vi "SentinelCtrlSim v25 - Copy.vi"() -> ()   [LabVIEW 2011]
uses:
  <userlib>/configTool/configTool.llb/initConfigGlobal.vi
  <userlib>/configTool/configTool.llb/loadConfigFile.vi
  <userlib>/configTool/configTool.llb/closeConfig.vi
  <userlib>/configTool/configTool.llb/getProperty(DBL).vi
  <userlib>/configTool/configTool.llb/getProperty(I32).vi
  <userlib>/configTool/configTool.llb/getProperty(U32).vi
  <userlib>/configTool/configTool.llb/getProperty(BOOL).vi
  <userlib>/configTool/configTool.llb/getProperty(STR).vi
panel:
  in  "Data log path and filename":path=path "configuraitons/default_configuraiton.cfg"
  in  "Panels":T1(tab)
  in  "Test cell ID":string="default"
  in  "Operator name":string="default"
  in  "Lot number":string="default"
  in  "Configuration file path and filename":path
  in  "POWER":bool=TRUE
  in  "H1 low yield warning":dbl=95.0 min=0.0 max=100.0 step=1.0
  in  "Ignore alarms until AFTER this many cycles":i32=20
  in  "H1 low yield alarm":dbl=85.0 min=0.0 max=100.0 step=1.0
  in  "H1 low UPH warning (%)":dbl=95.0 min=1.0 max=48000.0 step=1.0
  in  "H1 low UPH alarm (%)":dbl=90.0 min=1.0 max=48000.0 step=1.0
  in  "Enable data logging of all events":bool=TRUE
  in  "Enable electronic notification of alarms":bool
  in  "H2 low UPH alarm (%)":dbl=90.0 min=1.0 max=48000.0 step=1.0
  in  "H2 low UPH warning (%)":dbl=95.0 min=1.0 max=48000.0 step=1.0
  in  "H2 low yield alarm":dbl=90.0 min=0.0 max=100.0 step=1.0
  in  "H2  low yield warning":dbl=95.0 min=0.0 max=100.0 step=1.0
  in  "H1 enable halt\non yield alarm":bool
  in  "H2 enable halt\non yield alarm":bool
  in  "H1 enable halt\non UPH alarm":bool
  in  "H2 enable halt\non UPH alarm":bool
  out "IT lock 1":bool caption="Index time\noptimization ON:\nmanual control of index time is LOCKED"
  in  "Parallelism":u32(slide)=8 min=1 max=16 step=1 scale=1.0..16.0
  in  "Simulate at max speed":bool=TRUE
  in  "H2 yield\nvariation (%)":i32(slide) min=-20 max=0 step=1
  in  "H1 yield\nvariation (%)":i32(slide) min=-20 max=0 step=1
  in  "H2 index time\nvariation (%)":i32(slide) min=-20 max=20 step=1 scale=-20.0..20.0
  in  "H1 index time\nvariation (%)":i32(slide) min=-20 max=20 step=1 scale=-20.0..20.0
  in  "H2 yield set":dbl(slide)=100.0 min=0.0 max=100.0 step=1.0 scale=0.0..100.0
  in  "H1 yield  set":dbl(slide)=100.0 min=0.0 max=100.0 step=1.0 scale=0.0..100.0
  in  "H2 index\ntime set":dbl(slide)=1.7000000000000004 min=0.5 max=10.0 step=0.1 scale=0.5..10.0 scale format="%.1f"
  in  "Test time\nvariation (%)":i32(slide) min=-100 max=100 step=1 scale=-50.0..100.0
  in  "H1 index\ntime set":dbl(slide)=1.7000000000000004 min=0.5 max=10.0 step=0.1 scale=0.5..10.0 scale format="%#.1f"
  in  "Test time set":dbl(slide)=1.8 min=0.5 max=10.0 step=0.01 scale=0.5..10.0 scale format="%.2f"
  in  "H1 IT orig":dbl
  in  "H2 IT orig":dbl
  in  "Min Test Time":dbl=0.499 min=0.1 max=1.0 step=0.1 format="%#.1g"
  out "H2 Single Handler UPH":dbl
  out "H1 Single Handler UPH":dbl
  out "UPH averaging":u32=20 min=2 max=100 step=1
  out "Yield averaging":u32=20 min=2 max=100 step=1
  in  "Push to reset charts":bool
  in  "Run / Stop":bool
  in  "Optimize handler speed":bool
  out "H1 parallelism":u8
  out "Utilization averaging":i32=6 min=2 max=20 step=1
  out "H2 nominal 2":bool=TRUE
  out "H2 warning 2":bool
  out "H2 alarm 2":bool
  out "H1 nominal 2":bool=TRUE
  out "H1 warning 2":bool
  out "H1 alarm 2":bool
  out "H2 Lock":bool
  out "H1 Lock":bool
  out "System UPH":u32(knob) caption="Sys UPH" scale=0.0..16800.0 scale format="%#.0f"
  out "Time Accerlation  Factor":dbl caption="Time acceleration \nfactor" format="%.1f"
  out "H2 Test Time":dbl caption="Index Time" format="%.2f"
  out "H2 Index Time":dbl caption="Index Time" format="%.2f"
  out "H2 Yield Guage":cluster{dbl, dbl}(knob) caption="H2 yield" scale=0.0..100.0
  out "H2 UPH":cluster{u32, u32}(knob) scale=0.0..8000.0 scale format="%#.0f"
  out "H2 nominal":bool=TRUE
  out "H2 warning":bool
  out "H2 alarm":bool
  out "H2 Indexing":bool
  out "H2 Testing":bool
  out "H2 Waiting":bool
  out "H2 Device Count":u32 caption="Device Count"
  out "H2 On/Off-line":bool
  out "H1 Test Time":dbl caption="Index Time" format="%.2f"
  out "H1 Index Time":dbl caption="Index Time" format="%.2f"
  out "H1 Yield Guage":cluster{dbl, dbl}(knob) caption="H1 yield" scale=0.0..100.0
  out "H1 UPH":cluster{u32, u32}(knob) scale=0.0..8000.0 scale format="%#.0f"
  out "H1 nominal":bool=TRUE
  out "H1 warning":bool
  out "H1 alarm":bool
  out "H1 Indexing":bool
  out "H1 Testing":bool
  out "H1 Waiting":bool
  out "H1 Device Count":u32 caption="Decvice Count"
  out "H1 On/Off-line":bool
  out "H1 Wait Time":dbl caption="Index Time" format="%.2f"
  out "H2 Wait Time":dbl caption="Index Time" format="%.2f"
  out "H1 Good Units":u32 caption="Decvice Count"
  out "H2 Good Units":u32 caption="Device Count"
  out "Sys utilization":dbl(knob) caption="Yield" scale=0.0..100.0
  out "H1 Yield Mon":dbl format="%.1f"
  out "H2 Yield  Mon":dbl format="%.1f"
  in  "H2 online":bool=TRUE
  in  "H1 online":bool=TRUE
  in  "Tester ready":bool=TRUE
  in  "Alert volume":u32(knob)=5 max=10 step=1 scale=0.0..10.0
  in  "Audio On / Off":bool=TRUE
  out "H1 results":u32
  out "H2 results":u32
  out "SysUtilMon":cluster{i32, i32}(graph)
  out "H2 parallelism":u8 caption="H2 Paralellism"
  out "H1 Pass":bool=TRUE
  out "H2 Pass":bool=TRUE
  in  "system statuts":T2(ring)
  in  "system states":T3(ring)
  out "YieldMon":cluster{i32, i32, i32, i32}(graph)
  in  "Utilization (%)":u32=80 min=10 max=100 step=10
  out "Calendar days required\nfor testing all units":dbl format="%.1f"
  in  "# of devices to test":u32=10000000 min=1000 max=100000000 step=1000
  out "$ saved":i64 format="%#.0f"
  out "H2 calc UPH":dbl format="%#.0f"
  out "H2 IT (scycle)":dbl format="%.2f"
  out "H2 TT (s/cycle)":dbl format="%.2f"
  out "H2 WT (s/cycle)":dbl format="%.2f"
  out "H1 WT (s/cycle)":dbl format="%.2f"
  out "H1 IT (s/cycle)":dbl format="%.2f"
  out "H1 TT (s/cycle)":dbl format="%.2f"
  out "H2 units/cycle":dbl caption="H1 Parallelism"
  out "H1 Parallelism 2":dbl caption="H1 units/cycle"
  out "Sim H1 UPH":u32
  out "Sim H2 UPH":u32
  out "H1 Index Time 2":dbl caption="H1 index time"
  out "H1 Test Time 2":dbl caption="H1 test time"
  out "H1 parallelism":dbl
  out "Unit cost (cents/device)":cluster{dbl, dbl}(graph)
  out "UPH per unit area":cluster{dbl, dbl}(graph)
  out "H2 UPH per unit area":dbl format="%.1f"
  out "H1 calc UPH":dbl format="%#.0f"
  out "Std cell floorspace area":dbl
  out "Tandem unit cost\n(cents/device)":dbl format="%.3f"
  out "Hours per month 2":dbl caption="Hours per month"
  out "Total Mo Costs ($/mo) 3":dbl caption="Tandem mo cost ($/mo)"
  out "Total Mo Costs ($/mo) 2":dbl caption="Std mo cost ($/mo)"
  out "H1 UPH per unit area":dbl format="%.1f"
  out "Std mo cost ($/mo)":dbl
  out "Simulated\nsystem UPH":u32 caption="Simulated\nSystem UPH"
  out "Std unit cost\n(cents/device)":dbl format="%.3g"
  out "H1 calc UPH":dbl format="%#.0f"
  out "Tandem\nfloorspace area":dbl
  out "Tandem UPH\nper unit area":dbl format="%.1f"
  in  "Second handler cost ($/mo)":dbl=2500.0 min=0.0 max=10000.0 step=100.0
  out "Tandem hourly\ncost ($/hr)":dbl format="%.2f"
  in  "Hours per month":i32=730
  out "Std hourly\ncost ($/hr)":dbl format="%.2f"
  in  "Celerint licensing cost ($/mo)":dbl=1000.0 min=0.0 max=10000.0 step=100.0
  in  "Celerint hardware cost ($/mo)":dbl min=0.0 max=10000.0 step=1.0
  in  "Additional floorspace\nfor second handler":i32=50 min=0 max=1000 step=10
  in  "Std cell \nfloorspace area":i32=200 min=10 max=1000 step=10
  in  "Overhead ($/mo)":dbl=1000.0 min=0.0 max=10000.0 step=100.0
  in  "Handler cost ($/mo)":dbl=2500.0 min=0.0 max=100000.0 step=100.0
  in  "Tester cost ($/mo)":dbl=8500.0 min=0.0 max=100000.0 step=500.0
  in  "Cost \nupper\nlimit":dbl(slide)=0.3293436293436293 min=0.1 scale=0.1..10.0 scale format="%.1f"
  in  "Cost 10X":bool caption="10X"
  in  "UPH \nupper\nlimit":dbl(slide)=100.0 min=1.0 scale=0.009000000000000001..100.0
  in  "UPH 10X":bool caption="10X"
  out "Number of text alerts":dbl caption="Number of alerts\nsent as notifications"
  in  "Enable text notification":bool
  out "Notifications Lot Display":string="default" caption="Lot number (not editable)"
  in  "Include\ndata log as\nattachment":bool=TRUE
  out "Number of email alerts":dbl caption="Number of alerts\nsent as notifications"
  out "Email alert - attachment (not editable)":path
  in  "Email alert - message":string="An alarm event has ocurred on a semiconductor test lot that you have requested to monitor.  Please see the attached data log for event details.\n\nThis message is generated automatically by the Sentinel Controller program.\n\nTo stop these messages, please contact the test floor operator and disable automatic alert notifictions.\n\n"
  in  "Email alert - engineer":string="harry@celerint.com"
  in  "Email alert - CC":string="hjr@celerint.com"
  in  "Enable email notification":bool
  in  "Carrier":enum16{"T-Mobile", "AT&T", "Verizon", "Sprint"}(ring)=enum."AT&T"
  in  "Phone number":string="5128263411"
  in  "Subject":string="From: Sentinel Controller"
  in  "Body":string="An alarm event has ocurred"
  out "H1 UPH warning limit":dbl
  out "H1 UPH alarm limit":dbl
  out "H2 UPH warning limit":dbl
  out "H2 UPH alarm limit":dbl
  # "Sentinel Controller\nTandlem Handler\nTest Cell \nwww.celerint.com"
  # "Turning off POWER will stop execution the Sentinel Controller Program"
  # "INPUT FILE"
  # "LOT INFORMATION"
  # "Celerint Sentinel Controller Simulator"
  # "HANDLER PERFORMANCE THRESHOLDS"
  # "Handler  1"
  # "Handler 2"
  # "Set UPH thresholds as % of max UPH"
  # "Set UPH thresholds as % of max UPH"
  # "test cycles (insertions)"
  # "Celerint Sentinel Controller Simulator"
  # "Handler 2"
  # "Handler 1"
  # "Yield"
  # "UPH"
  # "Yield"
  # "UPH"
  # "Data"
  # "Avg"
  # "lot yield (%)"
  # "good devices"
  # "devices tested"
  # "wait time"
  # "index time"
  # "test time"
  # "H1"
  # "H2"
  # "waiting"
  # "testing"
  # "indexing"
  # "on/off-line"
  # "Celerint Sentinel Controller Simulator"
  # "STANDARD SETUP"
  # "H2 calculated\nsimilarly"
  # "3600"
  # "TANDEM HANDLER SETUP"
  # "SAVINGS"
  # "3600 (s/hr)"
  # "3600 (s/hr)"
  # "Sentinel Controller\nTandlem Handler\nTest Cell \nwww.celerint.com"
  # "Lot number will be appended automatically:"
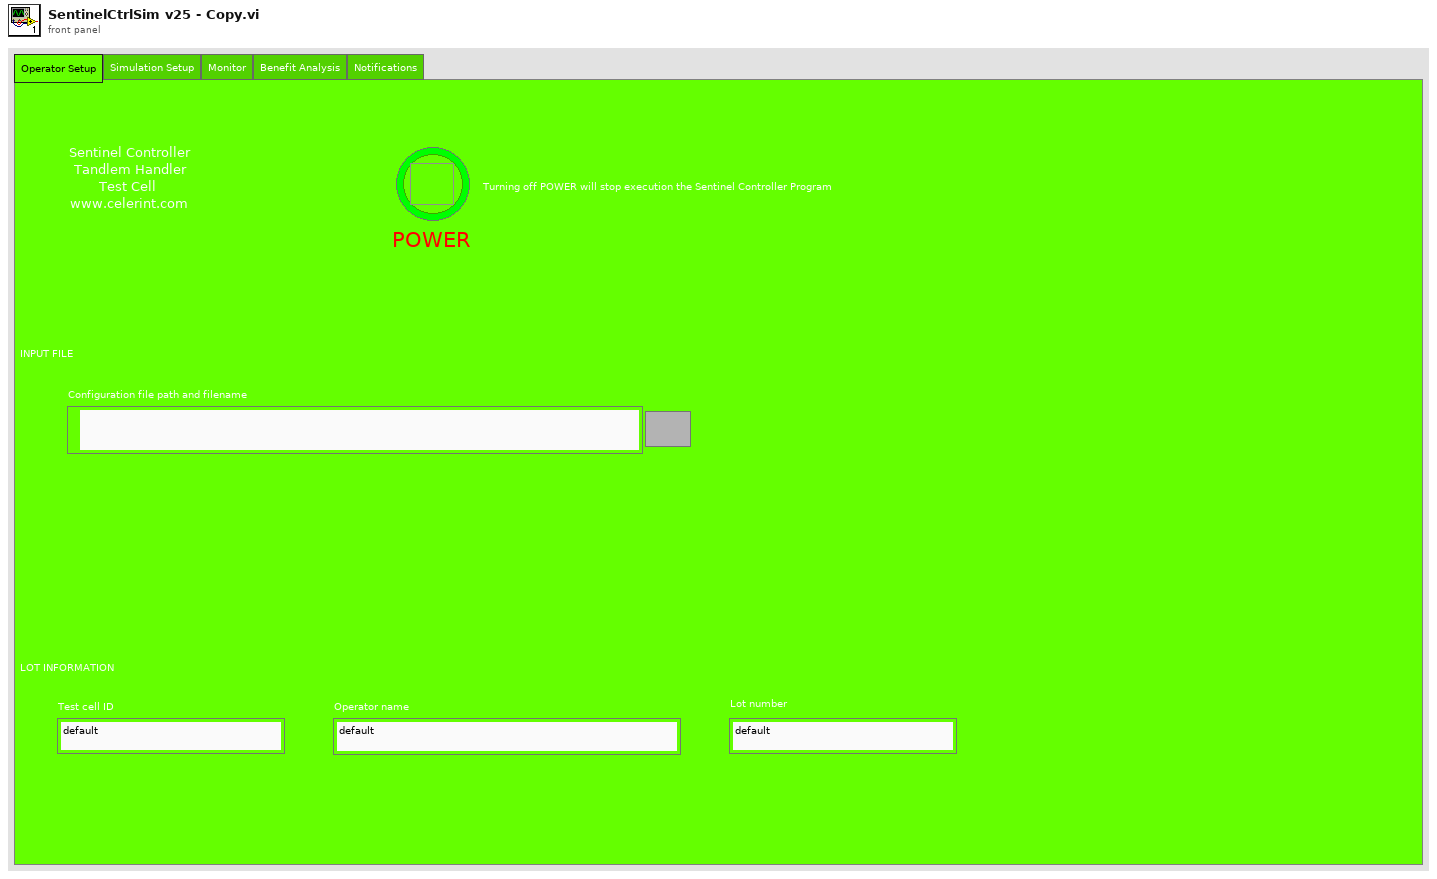
[diagram p1: front panel]
types:
  T1 = enum32{"Operator Setup", "Simulation Setup", "Monitor", "Benefit Analysis", "Notifications"}
  T2 = enum16{"H1NH2N", "H1NH2W", "H1NH2A", "H1WH2N", "H1WH2W", "H1WH2A", "H1AH2N", "H1AH2W", "H1AH2A"}
  T3 = enum16{"H1 Ready", "H2 Ready", "No Handler Ready"}
  T4 = enum16{"open", "replace", "create", "open or create", "replace or create", "replace or create with confirmation"}
  T5 = typedef "configRef.ctl" = refnum<vi>
  T6 = cluster{"rolling avg out":dbl, dbl, "H1 low yield alarm":dbl, "H2 low yield alarm":dbl}
  T7 = cluster{"rolling avg out":dbl, "H1 low yield alarm":dbl}
  T8 = cluster{dbl, "rolling avg out":dbl, "H1 low yield alarm":dbl, "H2 low yield alarm":dbl}
  T9 = cluster{"rolling avg out":dbl, "H2 low yield alarm":dbl}
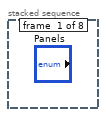
[diagram p2: hidden frame]
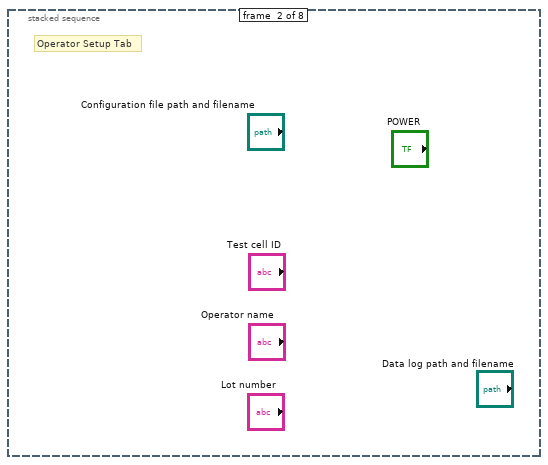
[diagram p3: hidden frame]
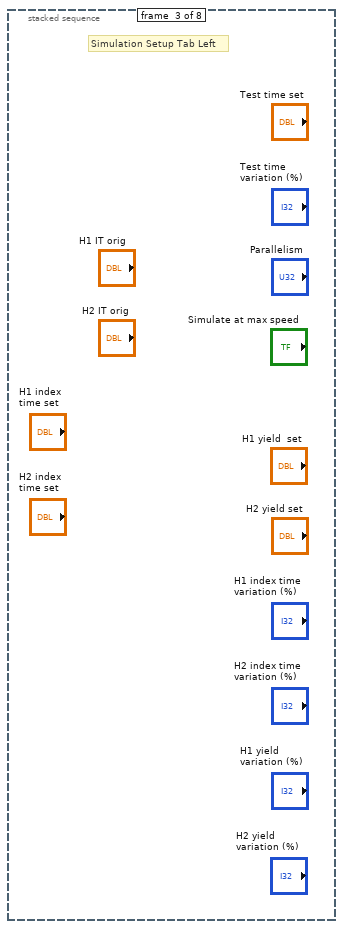
[diagram p4: hidden frame]
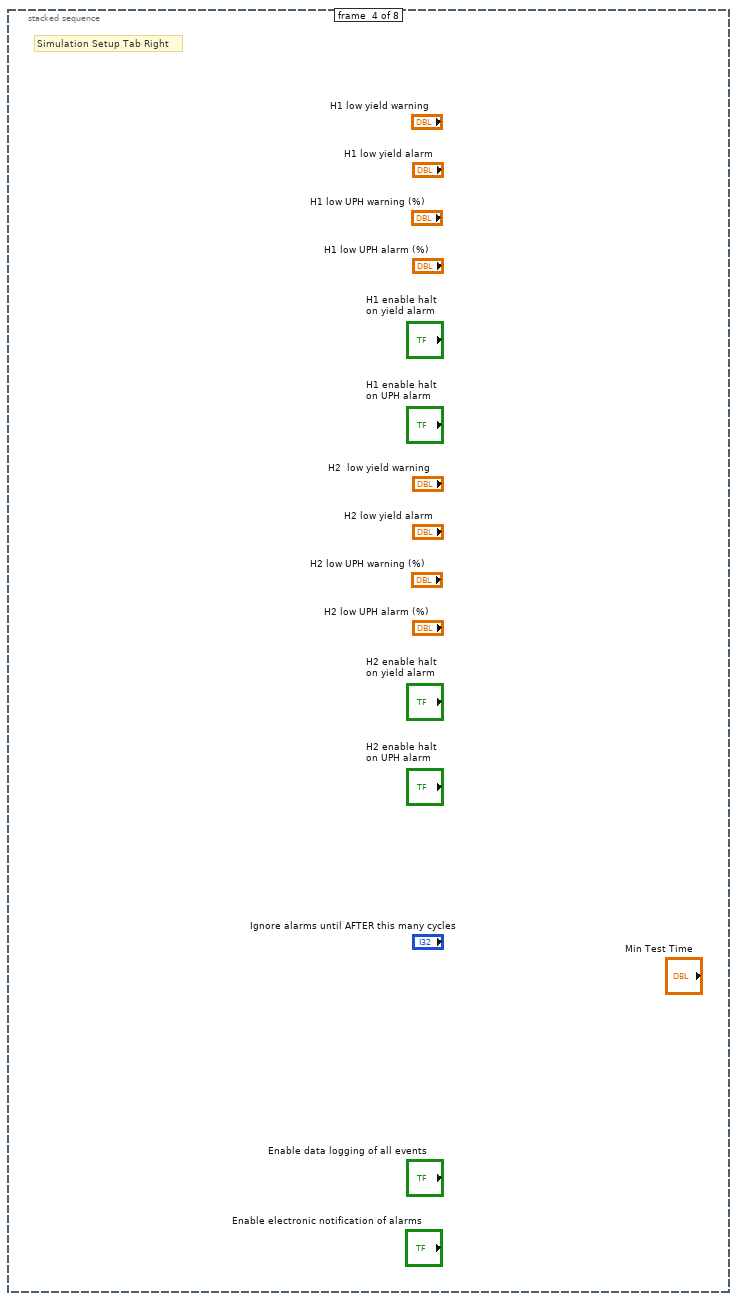
[diagram p5: hidden frame]
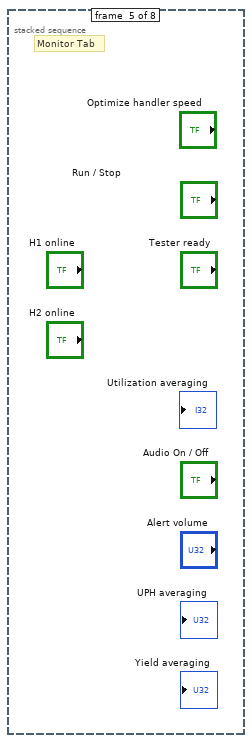
[diagram p6: hidden frame]
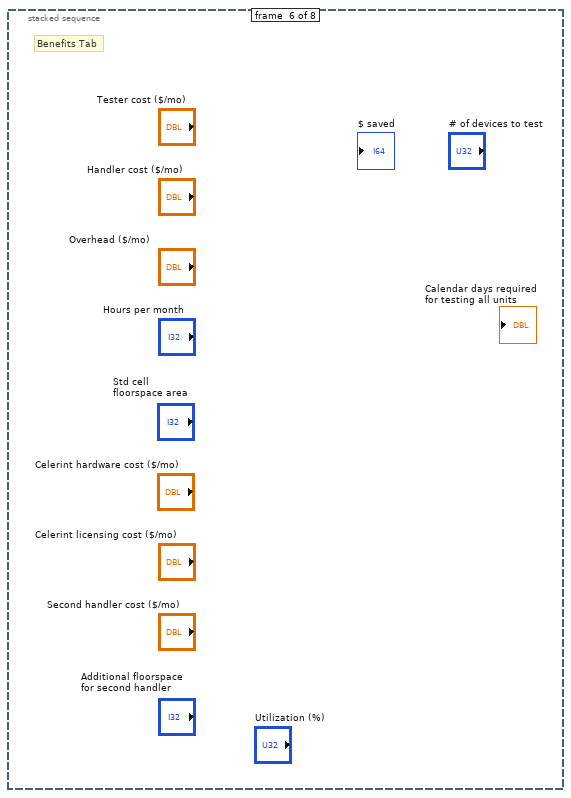
[diagram p7: hidden frame]
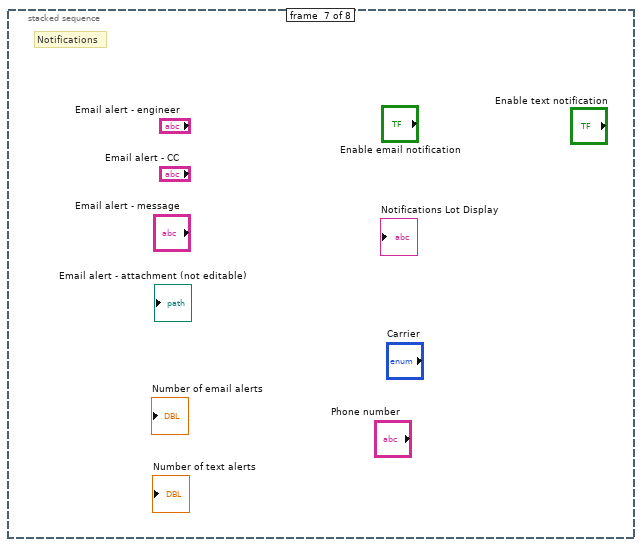
[diagram p8: hidden frame]
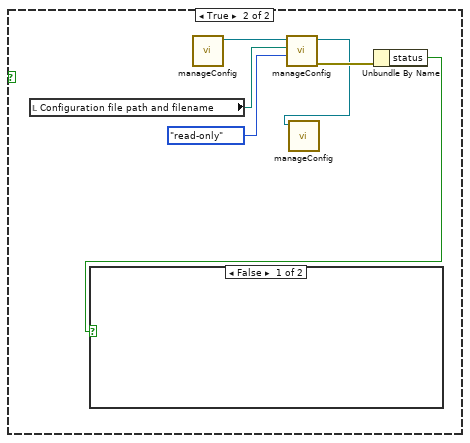
[diagram p9: hidden frame]
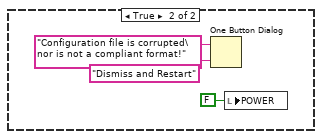
[diagram p10: hidden frame]
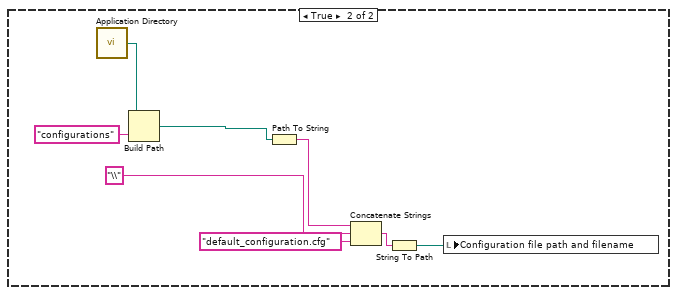
[diagram p11: hidden frame]
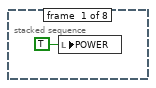
[diagram p13: hidden frame]
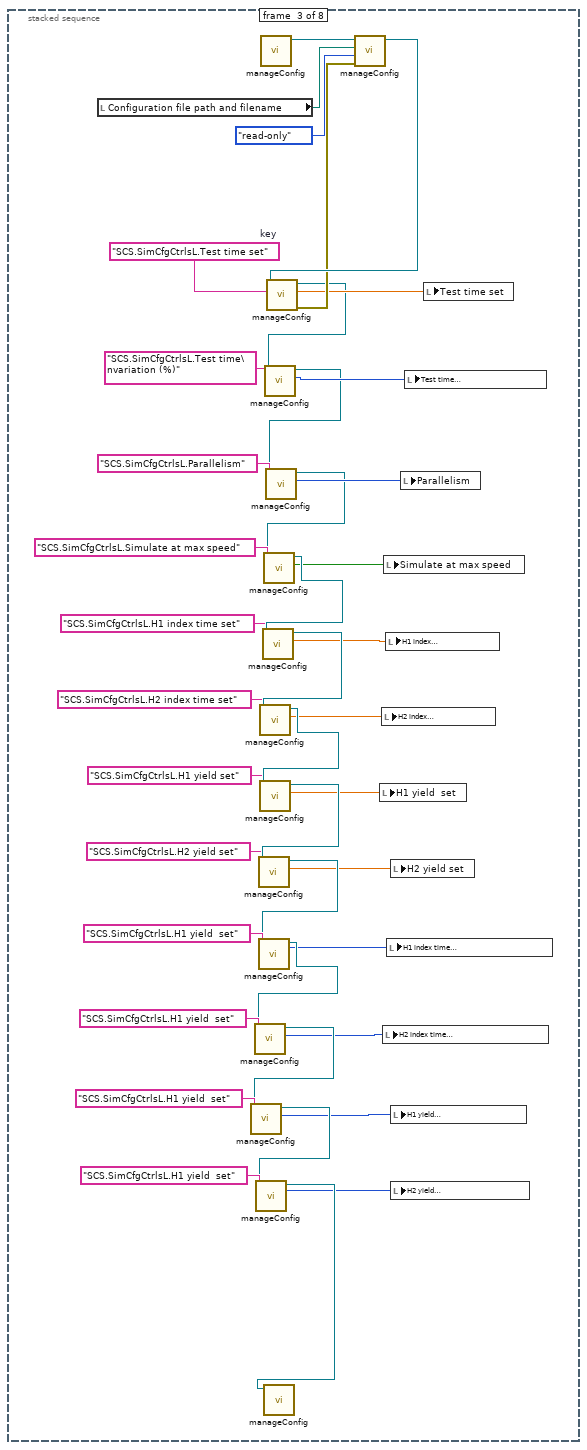
[diagram p15: hidden frame]
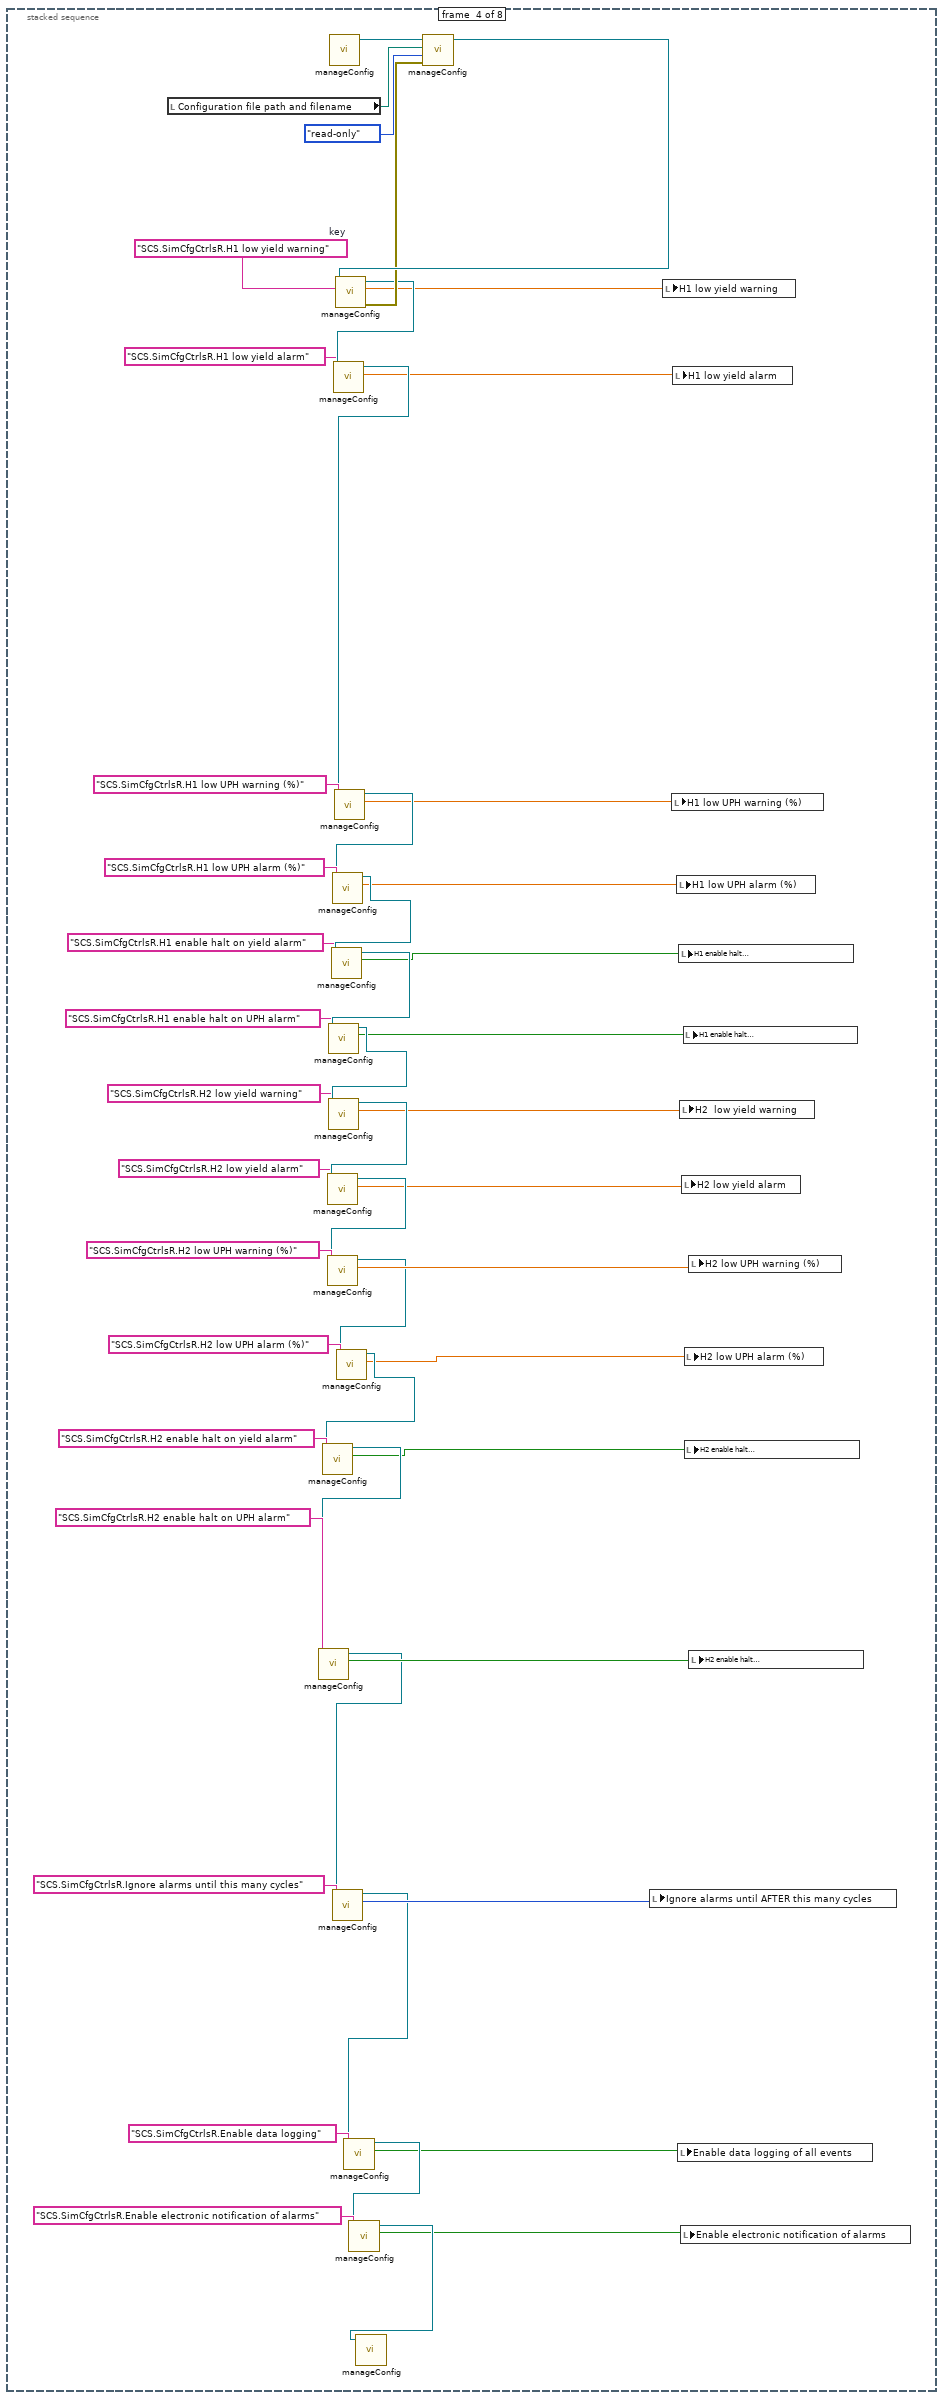
[diagram p16: hidden frame]
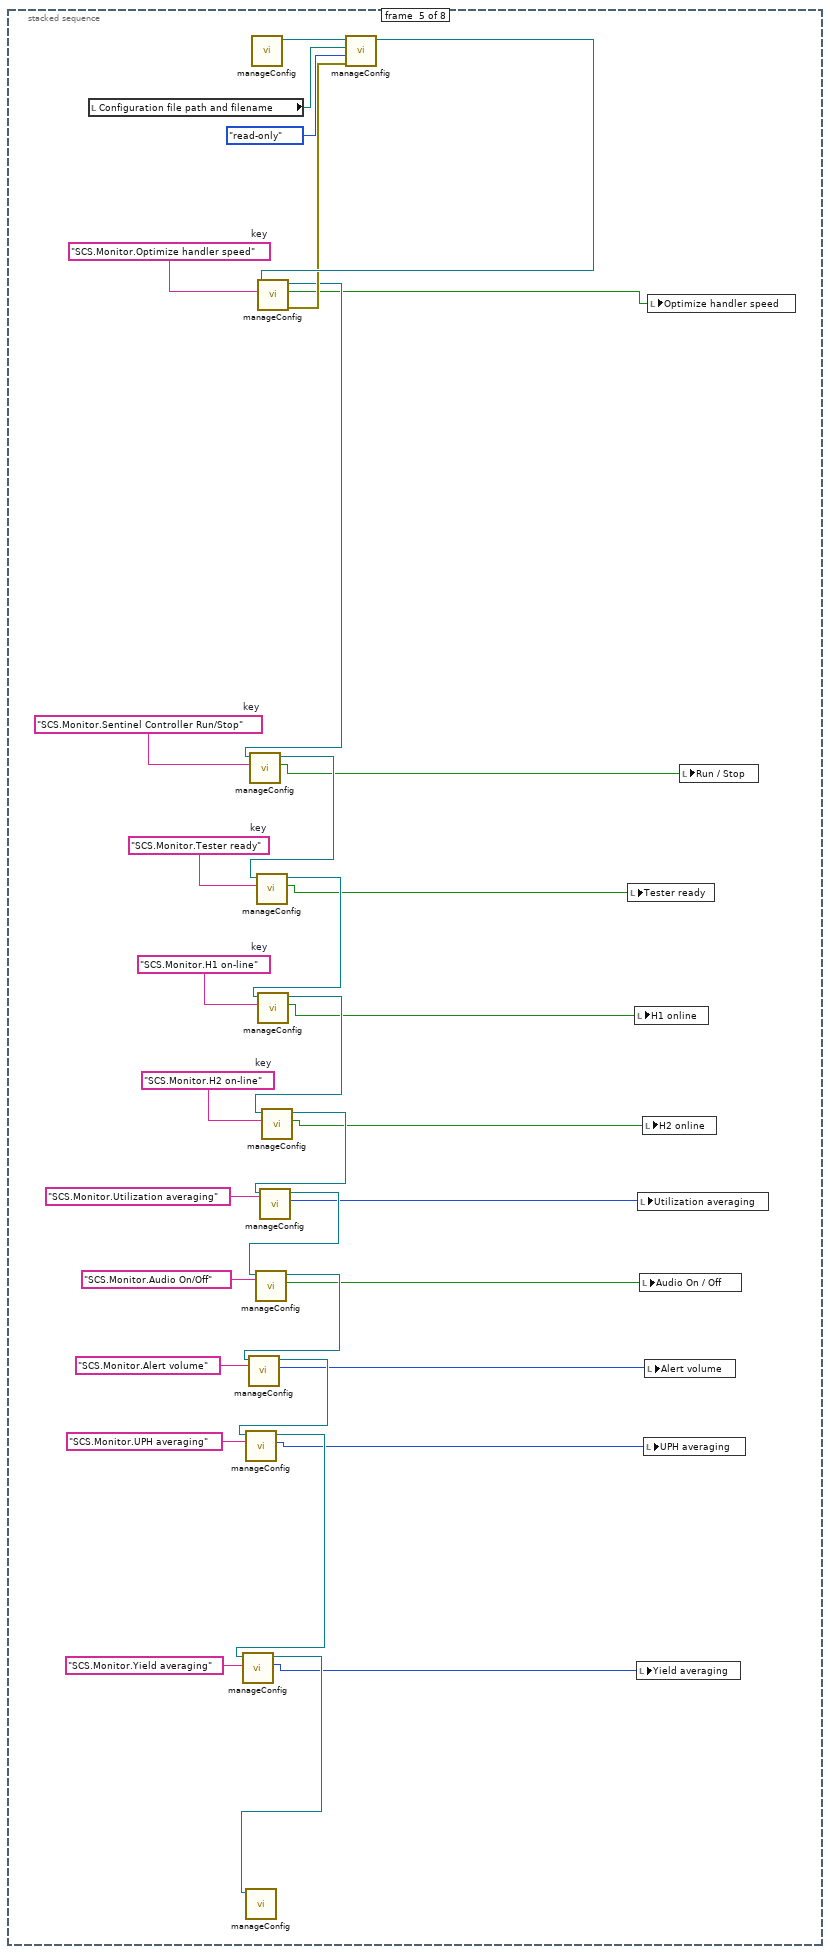
[diagram p17: hidden frame]
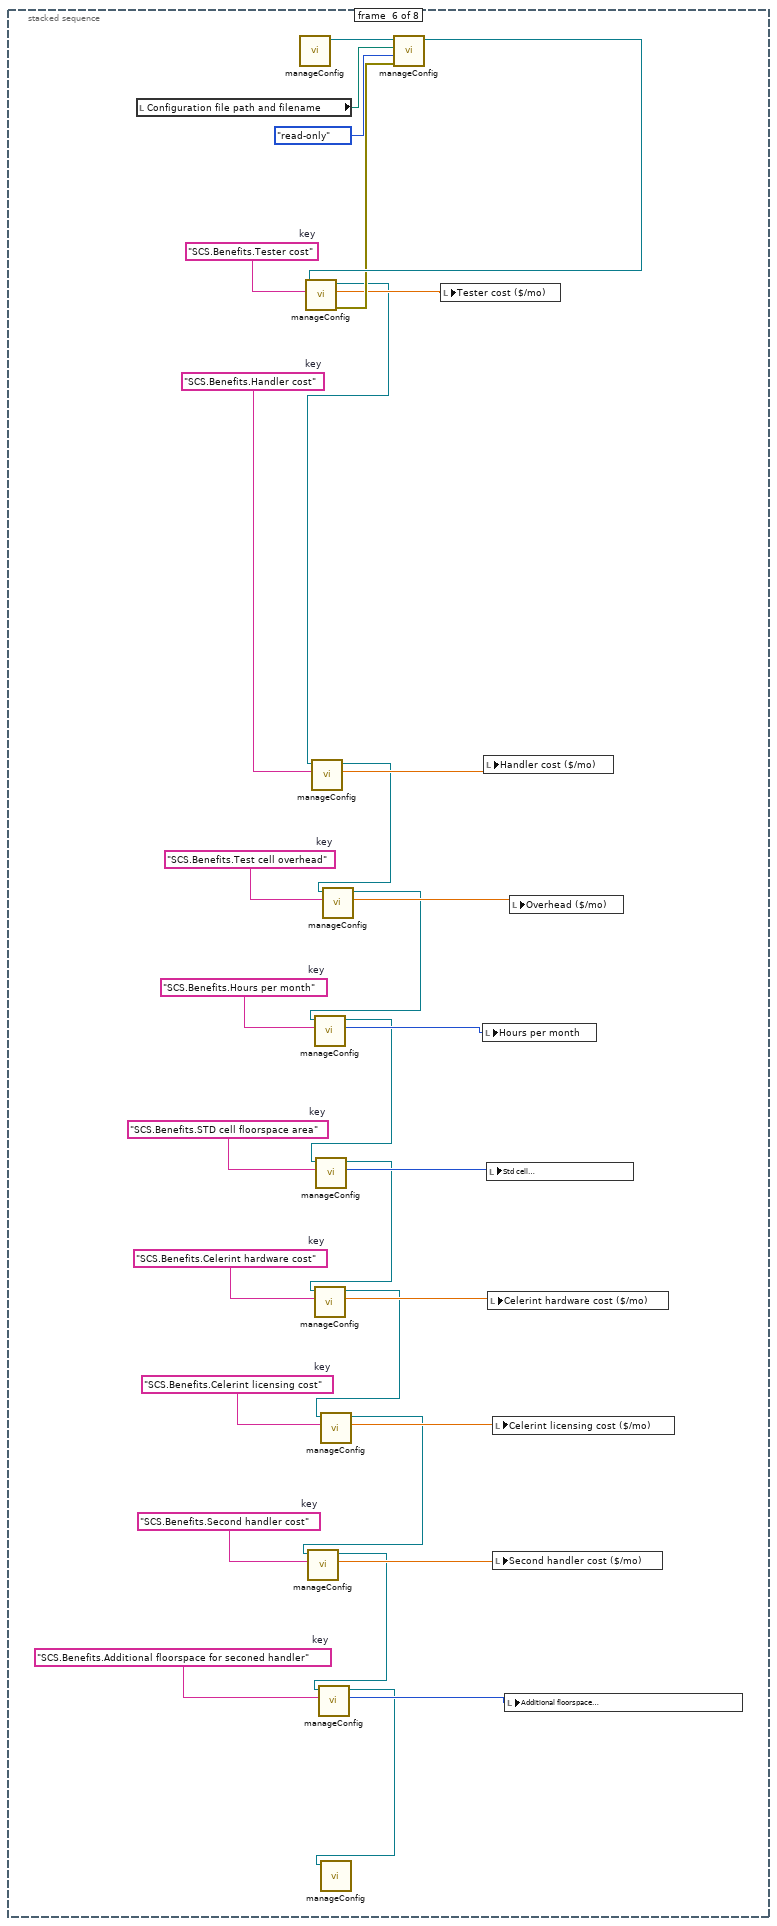
[diagram p18: hidden frame]
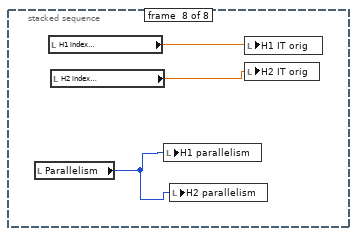
[diagram p19: hidden frame]
diagram:
  n1 = flat-sequence {
    frame #0 {
      # "This stacked sequence has all controls and indicators organized by the front panel panes."
      n2 = stacked-sequence {
        frame #0 {
        }
        frame #1 {
          # "Operator Setup Tab"
        }
        frame #2 {
          # "Simulation Setup Tab Left"
        }
        frame #3 {
          # "Simulation Setup Tab Right"
        }
        frame #4 {
          # "Monitor Tab"
        }
        frame #5 {
          # "Benefits Tab"
        }
        frame #6 {
          # "Notifications"
        }
        frame #7 {
          # "These are mostly indicators indicators"
        }
      }
    }
    frame #1 {
      n3 = local write "POWER"(TRUE ("POWER")) -> ()
    }
    frame #2 {
      n4 = local read "Configuration file path and filename"() -> (w4:path)
      n5 = Equal?(x=w4, y=path "") -> (x = y?=w3:bool)
      n6 = case shown="False" w3 {
        tunnel: w4 -> [w26 _]
        frame False {
          n7 = call <vilib>:"Check if File or Folder Exists.vi"("path"=w26) -> ("file or folder exists?"=w25:bool)  [unwired: 8 in, 2 out]
          n8 = case shown="False" w25 {
            frame False {
              n9 = local write "POWER"(FALSE ("POWER")) -> ()
              n10 = One Button Dialog(message="Configuration file does not exist!", button name ("OK")="Dismiss and Restart") -> ()  [unwired: 1 out]
            }
            frame True {
              n11 = local read "Configuration file path and filename"() -> (w33:path)
              n12 = call-poly <userlib>:"manageConfig.vi"() -> ("config ref out"=w34:T5)  [unwired: 10 in, 1 out]
              n13 = call-poly <userlib>:"manageConfig.vi"("access (0:read/write)"=enum16{"read/write", "read-only", "write-only"}."read-only", "config file path"=w33, "config ref"=w34) -> ("error out"=w32:errorcluster, "config ref out"=w30:T5)  [unwired: 6 in, 1 out]
              n14 = call-poly <userlib>:"manageConfig.vi"("config ref"=w30) -> ()  [unwired: 10 in, 1 out]
              n15 = Unbundle By Name(w32) -> ("status"=w31:bool)
              n16 = case shown="False" w31 {
                frame False {
                }
                frame True {
                  n17 = One Button Dialog(message="Configuration file is corrupted\nor is not a compliant format!", button name ("OK")="Dismiss and Restart") -> ()  [unwired: 1 out]
                  n18 = local write "POWER"(FALSE ("POWER")) -> ()
                }
              }
            }
          }
        }
        frame True {
          n19 = call <vilib>:"Application Directory.vi"() -> ("Application Directory"=w42:path)
          n20 = Build Path(base path=w42, name or relative path="configurations") -> (appended path=w39:path)
          n21 = Path To String(path=w39) -> (string=w44:string)
          n22 = Concatenate Strings(w44, "\\" ("string"), "default_configuration.cfg" ("string")) -> (w45:string)
          n23 = String To Path(string=w45) -> (path=w46:path)
          n24 = local write "Configuration file path and filename"(w46) -> ()
        }
      }
      n25 = Get Date/Time String(want seconds? (F)=TRUE) -> (date string=w19:string, time string=w11:string)  [unwired: 2 in]
      n26 = call <vilib>:"Application Directory.vi"() -> ("Application Directory"=w6:path)
      n27 = Build Path(base path=w6, name or relative path="datalogs") -> (appended path=w24:path)
      n28 = Search and Replace String(replace all?=TRUE ("replace all? (F)"), input string=w19, search string="/", replace string="-" ("replace string (\"\")")) -> (result string=w9:string)  [unwired: 4 in, 3 out]
      n29 = Search and Replace String(replace all?=TRUE ("replace all? (F)"), input string=w11, search string=":", replace string="." ("replace string (\"\")")) -> (result string=w10:string)  [unwired: 4 in, 3 out]
      n30 = Path To String(path=w24) -> (string=w15:string)
      n31 = Concatenate Strings(w15, "\\" ("string"), w9, " " ("string"), w10, ".txt" ("string")) -> (w21:string)
      n32 = String To Path(string=w21) -> (path=w23:path)
      n33 = local write "Data log path and filename"(w23) -> ()
    }
    frame #3 {
      n34 = local read "POWER"() -> (w47:bool)
      n35 = case shown="True" w47 {
        frame False {
        }
        frame True {
          n36 = stacked-sequence {
            frame #0 {
              n37 = local write "POWER"(TRUE ("POWER")) -> ()
            }
            frame #1 {
              # "nothing to do for the operator frame"
            }
            frame #2 {
              w88 = "SCS.SimCfgCtrlsL.Test time set"  # key
              n38 = local read "Configuration file path and filename"() -> (w84:path)
              n39 = call-poly <userlib>:"manageConfig.vi"() -> ("config ref out"=w85:T5)  [unwired: 10 in, 1 out]
              n40 = call-poly <userlib>:"manageConfig.vi"("access (0:read/write)"=enum16{"read/write", "read-only", "write-only"}."read-only", "config file path"=w84, "config ref"=w85) -> ("error out"=w87:errorcluster, "config ref out"=w89:T5)  [unwired: 6 in, 1 out]
              n41 = call-poly <userlib>:"manageConfig.vi"("error in"=w87, "property path"=w88, "config ref"=w89) -> ("data"=w81:dbl, "config ref out"=w63:T5)  [unwired: 5 in, 2 out]
              n42 = call-poly <userlib>:"manageConfig.vi"("property path"="SCS.SimCfgCtrlsL.Test time\nvariation (%)", "config ref"=w63) -> ("value"=w80:i32, "config ref out"=w62:T5)  [unwired: 6 in, 2 out]
              n43 = call-poly <userlib>:"manageConfig.vi"("property path"="SCS.SimCfgCtrlsL.Parallelism", "config ref"=w62) -> ("value"=w79:u32, "config ref out"=w64:T5)  [unwired: 6 in, 2 out]
              n44 = call-poly <userlib>:"manageConfig.vi"("property path"="SCS.SimCfgCtrlsL.Simulate at max speed", "config ref"=w64) -> ("value"=w61:bool, "config ref out"=w65:T5)  [unwired: 6 in, 2 out]
              n45 = call-poly <userlib>:"manageConfig.vi"("property path"="SCS.SimCfgCtrlsL.H1 index time set", "config ref"=w65) -> ("data"=w60:dbl, "config ref out"=w66:T5)  [unwired: 6 in, 2 out]
              n46 = call-poly <userlib>:"manageConfig.vi"("property path"="SCS.SimCfgCtrlsL.H2 index time set", "config ref"=w66) -> ("data"=w59:dbl, "config ref out"=w67:T5)  [unwired: 6 in, 2 out]
              n47 = call-poly <userlib>:"manageConfig.vi"("property path"="SCS.SimCfgCtrlsL.H1 yield set", "config ref"=w67) -> ("data"=w58:dbl, "config ref out"=w68:T5)  [unwired: 6 in, 2 out]
              n48 = call-poly <userlib>:"manageConfig.vi"("property path"="SCS.SimCfgCtrlsL.H2 yield set", "config ref"=w68) -> ("data"=w57:dbl, "config ref out"=w69:T5)  [unwired: 6 in, 2 out]
              n49 = call-poly <userlib>:"manageConfig.vi"("property path"="SCS.SimCfgCtrlsL.H1 yield  set", "config ref"=w69) -> ("value"=w56:i32, "config ref out"=w70:T5)  [unwired: 6 in, 2 out]
              n50 = call-poly <userlib>:"manageConfig.vi"("property path"="SCS.SimCfgCtrlsL.H1 yield  set", "config ref"=w70) -> ("value"=w55:i32, "config ref out"=w71:T5)  [unwired: 6 in, 2 out]
              n51 = call-poly <userlib>:"manageConfig.vi"("property path"="SCS.SimCfgCtrlsL.H1 yield  set", "config ref"=w71) -> ("value"=w54:i32, "config ref out"=w72:T5)  [unwired: 6 in, 2 out]
              n52 = call-poly <userlib>:"manageConfig.vi"("property path"="SCS.SimCfgCtrlsL.H1 yield  set", "config ref"=w72) -> ("value"=w53:i32, "config ref out"=w73:T5)  [unwired: 6 in, 2 out]
              n53 = call-poly <userlib>:"manageConfig.vi"("config ref"=w73) -> ()  [unwired: 10 in, 1 out]
              n54 = local write "H1 yield  set"(w58) -> ()
              n55 = local write "H2 index\ntime set"(w59) -> ()
              n56 = local write "H2 index time\nvariation (%)"(w55) -> ()
              n57 = local write "Simulate at max speed"(w61) -> ()
              n58 = local write "H1 index\ntime set"(w60) -> ()
              n59 = local write "H1 index time\nvariation (%)"(w56) -> ()
              n60 = local write "H2 yield set"(w57) -> ()
              n61 = local write "H1 yield\nvariation (%)"(w54) -> ()
              n62 = local write "H2 yield\nvariation (%)"(w53) -> ()
              n63 = local write "Parallelism"(w79) -> ()
              n64 = local write "Test time\nvariation (%)"(w80) -> ()
              n65 = local write "Test time set"(w81) -> ()
            }
            frame #3 {
              w138 = "SCS.SimCfgCtrlsR.H1 low yield warning"  # key
              n66 = local read "Configuration file path and filename"() -> (w134:path)
              n67 = call-poly <userlib>:"manageConfig.vi"() -> ("config ref out"=w135:T5)  [unwired: 10 in, 1 out]
              n68 = call-poly <userlib>:"manageConfig.vi"("access (0:read/write)"=enum16{"read/write", "read-only", "write-only"}."read-only", "config file path"=w134, "config ref"=w135) -> ("error out"=w137:errorcluster, "config ref out"=w139:T5)  [unwired: 6 in, 1 out]
              n69 = call-poly <userlib>:"manageConfig.vi"("error in"=w137, "property path"=w138, "config ref"=w139) -> ("data"=w110:dbl, "config ref out"=w121:T5)  [unwired: 5 in, 2 out]
              n70 = call-poly <userlib>:"manageConfig.vi"("property path"="SCS.SimCfgCtrlsR.H1 low yield alarm", "config ref"=w121) -> ("data"=w109:dbl, "config ref out"=w120:T5)  [unwired: 6 in, 2 out]
              n71 = call-poly <userlib>:"manageConfig.vi"("property path"="SCS.SimCfgCtrlsR.H1 low UPH warning (%)", "config ref"=w120) -> ("data"=w108:dbl, "config ref out"=w122:T5)  [unwired: 6 in, 2 out]
              n72 = call-poly <userlib>:"manageConfig.vi"("property path"="SCS.SimCfgCtrlsR.H1 low UPH alarm (%)", "config ref"=w122) -> ("data"=w107:dbl, "config ref out"=w123:T5)  [unwired: 6 in, 2 out]
              n73 = call-poly <userlib>:"manageConfig.vi"("property path"="SCS.SimCfgCtrlsR.H1 enable halt on yield alarm", "config ref"=w123) -> ("value"=w106:bool, "config ref out"=w124:T5)  [unwired: 6 in, 2 out]
              n74 = call-poly <userlib>:"manageConfig.vi"("property path"="SCS.SimCfgCtrlsR.H1 enable halt on UPH alarm", "config ref"=w124) -> ("value"=w105:bool, "config ref out"=w125:T5)  [unwired: 6 in, 2 out]
              n75 = call-poly <userlib>:"manageConfig.vi"("property path"="SCS.SimCfgCtrlsR.H2 low yield warning", "config ref"=w125) -> ("data"=w104:dbl, "config ref out"=w126:T5)  [unwired: 6 in, 2 out]
              n76 = call-poly <userlib>:"manageConfig.vi"("property path"="SCS.SimCfgCtrlsR.H2 low yield alarm", "config ref"=w126) -> ("data"=w103:dbl, "config ref out"=w127:T5)  [unwired: 6 in, 2 out]
              n77 = call-poly <userlib>:"manageConfig.vi"("property path"="SCS.SimCfgCtrlsR.H2 low UPH warning (%)", "config ref"=w127) -> ("data"=w102:dbl, "config ref out"=w94:T5)  [unwired: 6 in, 2 out]
              n78 = call-poly <userlib>:"manageConfig.vi"("property path"="SCS.SimCfgCtrlsR.H2 low UPH alarm (%)", "config ref"=w94) -> ("data"=w92:dbl, "config ref out"=w93:T5)  [unwired: 6 in, 2 out]
              n79 = call-poly <userlib>:"manageConfig.vi"("property path"="SCS.SimCfgCtrlsR.H2 enable halt on yield alarm", "config ref"=w93) -> ("value"=w101:bool, "config ref out"=w128:T5)  [unwired: 6 in, 2 out]
              n80 = call-poly <userlib>:"manageConfig.vi"("property path"="SCS.SimCfgCtrlsR.H2 enable halt on UPH alarm", "config ref"=w128) -> ("value"=w100:bool, "config ref out"=w91:T5)  [unwired: 6 in, 2 out]
              n81 = call-poly <userlib>:"manageConfig.vi"("property path"="SCS.SimCfgCtrlsR.Ignore alarms until this many cycles", "config ref"=w91) -> ("value"=w99:i32, "config ref out"=w90:T5)  [unwired: 6 in, 2 out]
              n82 = call-poly <userlib>:"manageConfig.vi"("property path"="SCS.SimCfgCtrlsR.Enable data logging", "config ref"=w90) -> ("value"=w98:bool, "config ref out"=w112:T5)  [unwired: 6 in, 2 out]
              n83 = call-poly <userlib>:"manageConfig.vi"("property path"="SCS.SimCfgCtrlsR.Enable electronic notification of alarms", "config ref"=w112) -> ("value"=w97:bool, "config ref out"=w111:T5)  [unwired: 6 in, 2 out]
              n84 = call-poly <userlib>:"manageConfig.vi"("config ref"=w111) -> ()  [unwired: 10 in, 1 out]
              n85 = local write "Ignore alarms until AFTER this many cycles"(w99) -> ()
              n86 = local write "H1 low yield warning"(w110) -> ()
              n87 = local write "H1 low UPH warning (%)"(w108) -> ()
              n88 = local write "H1 low yield alarm"(w109) -> ()
              n89 = local write "H1 low UPH alarm (%)"(w107) -> ()
              n90 = local write "Enable data logging of all events"(w98) -> ()
              n91 = local write "H1 enable halt\non yield alarm"(w106) -> ()
              n92 = local write "H2  low yield warning"(w104) -> ()
              n93 = local write "Enable electronic notification of alarms"(w97) -> ()
              n94 = local write "H2 low yield alarm"(w103) -> ()
              n95 = local write "H1 enable halt\non UPH alarm"(w105) -> ()
              n96 = local write "H2 low UPH alarm (%)"(w92) -> ()
              n97 = local write "H2 enable halt\non yield alarm"(w101) -> ()
              n98 = local write "H2 low UPH warning (%)"(w102) -> ()
              n99 = local write "H2 enable halt\non UPH alarm"(w100) -> ()
            }
            frame #4 {
              w165 = "SCS.Monitor.H2 on-line"  # key
              w166 = "SCS.Monitor.H1 on-line"  # key
              w167 = "SCS.Monitor.Tester ready"  # key
              w168 = "SCS.Monitor.Sentinel Controller Run/Stop"  # key
              w173 = "SCS.Monitor.Optimize handler speed"  # key
              n100 = local read "Configuration file path and filename"() -> (w169:path)
              n101 = call-poly <userlib>:"manageConfig.vi"() -> ("config ref out"=w170:T5)  [unwired: 10 in, 1 out]
              n102 = call-poly <userlib>:"manageConfig.vi"("access (0:read/write)"=enum16{"read/write", "read-only", "write-only"}."read-only", "config file path"=w169, "config ref"=w170) -> ("error out"=w172:errorcluster, "config ref out"=w174:T5)  [unwired: 6 in, 1 out]
              n103 = call-poly <userlib>:"manageConfig.vi"("error in"=w172, "property path"=w173, "config ref"=w174) -> ("value"=w149:bool, "config ref out"=w164:T5)  [unwired: 5 in, 2 out]
              n104 = call-poly <userlib>:"manageConfig.vi"("property path"=w168, "config ref"=w164) -> ("value"=w148:bool, "config ref out"=w163:T5)  [unwired: 6 in, 2 out]
              n105 = call-poly <userlib>:"manageConfig.vi"("property path"=w167, "config ref"=w163) -> ("value"=w147:bool, "config ref out"=w162:T5)  [unwired: 6 in, 2 out]
              n106 = call-poly <userlib>:"manageConfig.vi"("property path"=w166, "config ref"=w162) -> ("value"=w146:bool, "config ref out"=w161:T5)  [unwired: 6 in, 2 out]
              n107 = call-poly <userlib>:"manageConfig.vi"("property path"=w165, "config ref"=w161) -> ("value"=w145:bool, "config ref out"=w160:T5)  [unwired: 6 in, 2 out]
              n108 = call-poly <userlib>:"manageConfig.vi"("property path"="SCS.Monitor.Utilization averaging", "config ref"=w160) -> ("value"=w140:i32, "config ref out"=w159:T5)  [unwired: 6 in, 2 out]
              n109 = call-poly <userlib>:"manageConfig.vi"("property path"="SCS.Monitor.Audio On/Off", "config ref"=w159) -> ("value"=w144:bool, "config ref out"=w158:T5)  [unwired: 6 in, 2 out]
              n110 = call-poly <userlib>:"manageConfig.vi"("property path"="SCS.Monitor.Alert volume", "config ref"=w158) -> ("value"=w143:u32, "config ref out"=w157:T5)  [unwired: 6 in, 2 out]
              n111 = call-poly <userlib>:"manageConfig.vi"("property path"="SCS.Monitor.UPH averaging", "config ref"=w157) -> ("value"=w142:u32, "config ref out"=w156:T5)  [unwired: 6 in, 2 out]
              n112 = call-poly <userlib>:"manageConfig.vi"("property path"="SCS.Monitor.Yield averaging", "config ref"=w156) -> ("value"=w141:u32, "config ref out"=w155:T5)  [unwired: 6 in, 2 out]
              n113 = call-poly <userlib>:"manageConfig.vi"("config ref"=w155) -> ()  [unwired: 10 in, 1 out]
              n114 = local write "Tester ready"(w147) -> ()
              n115 = local write "H1 online"(w146) -> ()
              n116 = local write "Yield averaging"(w141) -> ()
              n117 = local write "Utilization averaging"(w140) -> ()
              n118 = local write "Audio On / Off"(w144) -> ()
              n119 = local write "H2 online"(w145) -> ()
              n120 = local write "UPH averaging"(w142) -> ()
              n121 = local write "Alert volume"(w143) -> ()
              n122 = local write "Optimize handler speed"(w149) -> ()
              n123 = local write "Run / Stop"(w148) -> ()
            }
            frame #5 {
              w193 = "SCS.Benefits.Additional floorspace for seconed handler"  # key
              w194 = "SCS.Benefits.Second handler cost"  # key
              w195 = "SCS.Benefits.Celerint licensing cost"  # key
              w196 = "SCS.Benefits.Celerint hardware cost"  # key
              w197 = "SCS.Benefits.STD cell floorspace area"  # key
              w198 = "SCS.Benefits.Hours per month"  # key
              w199 = "SCS.Benefits.Test cell overhead"  # key
              w200 = "SCS.Benefits.Handler cost"  # key
              w205 = "SCS.Benefits.Tester cost"  # key
              n124 = local read "Configuration file path and filename"() -> (w201:path)
              n125 = call-poly <userlib>:"manageConfig.vi"() -> ("config ref out"=w202:T5)  [unwired: 10 in, 1 out]
              n126 = call-poly <userlib>:"manageConfig.vi"("access (0:read/write)"=enum16{"read/write", "read-only", "write-only"}."read-only", "config file path"=w201, "config ref"=w202) -> ("error out"=w204:errorcluster, "config ref out"=w206:T5)  [unwired: 6 in, 1 out]
              n127 = call-poly <userlib>:"manageConfig.vi"("error in"=w204, "property path"=w205, "config ref"=w206) -> ("data"=w192:dbl, "config ref out"=w183:T5)  [unwired: 5 in, 2 out]
              n128 = call-poly <userlib>:"manageConfig.vi"("property path"=w200, "config ref"=w183) -> ("data"=w191:dbl, "config ref out"=w182:T5)  [unwired: 6 in, 2 out]
              n129 = call-poly <userlib>:"manageConfig.vi"("property path"=w199, "config ref"=w182) -> ("data"=w190:dbl, "config ref out"=w181:T5)  [unwired: 6 in, 2 out]
              n130 = call-poly <userlib>:"manageConfig.vi"("property path"=w198, "config ref"=w181) -> ("value"=w189:i32, "config ref out"=w180:T5)  [unwired: 6 in, 2 out]
              n131 = call-poly <userlib>:"manageConfig.vi"("property path"=w197, "config ref"=w180) -> ("value"=w188:i32, "config ref out"=w179:T5)  [unwired: 6 in, 2 out]
              n132 = call-poly <userlib>:"manageConfig.vi"("property path"=w196, "config ref"=w179) -> ("data"=w187:dbl, "config ref out"=w178:T5)  [unwired: 6 in, 2 out]
              n133 = call-poly <userlib>:"manageConfig.vi"("property path"=w195, "config ref"=w178) -> ("data"=w186:dbl, "config ref out"=w177:T5)  [unwired: 6 in, 2 out]
              n134 = call-poly <userlib>:"manageConfig.vi"("property path"=w194, "config ref"=w177) -> ("data"=w185:dbl, "config ref out"=w176:T5)  [unwired: 6 in, 2 out]
              n135 = call-poly <userlib>:"manageConfig.vi"("property path"=w193, "config ref"=w176) -> ("value"=w184:i32, "config ref out"=w175:T5)  [unwired: 6 in, 2 out]
              n136 = call-poly <userlib>:"manageConfig.vi"("config ref"=w175) -> ()  [unwired: 10 in, 1 out]
              n137 = local write "Tester cost ($/mo)"(w192) -> ()
              n138 = local write "Hours per month"(w189) -> ()
              n139 = local write "Handler cost ($/mo)"(w191) -> ()
              n140 = local write "Std cell \nfloorspace area"(w188) -> ()
              n141 = local write "Celerint hardware cost ($/mo)"(w187) -> ()
              n142 = local write "Celerint licensing cost ($/mo)"(w186) -> ()
              n143 = local write "Second handler cost ($/mo)"(w185) -> ()
              n144 = local write "Additional floorspace\nfor second handler"(w184) -> ()
              n145 = local write "Overhead ($/mo)"(w190) -> ()
            }
            frame #6 {
              w211 = "SCS.Notification.Enable text notification"  # key
              w217 = "SCS.Notification.Phone Number"  # key
              w218 = "SCS.Notification.Enable email notification"  # key
              w227 = "SCS.Notification.Email alert - Engineer"  # key
              n146 = local read "Configuration file path and filename"() -> (w224:path)
              n147 = local read "Lot number"() -> (w219:string)
              n148 = call-poly <userlib>:"manageConfig.vi"() -> ("config ref out"=w225:T5)  [unwired: 10 in, 1 out]
              n149 = local write "Number of email alerts"(0.0 ("Number of Emails Alerts Sent")) -> ()
              n150 = local write "Number of text alerts"(0.0 ("Number of Emails Alerts Sent")) -> ()
              n151 = local write "Notifications Lot Display"(w219) -> ()
              n152 = call-poly <userlib>:"manageConfig.vi"("access (0:read/write)"=enum16{"read/write", "read-only", "write-only"}."read-only", "config file path"=w224, "config ref"=w225) -> ("config ref out"=w228:T5)  [unwired: 6 in, 2 out]
              n153 = call-poly <userlib>:"manageConfig.vi"("property path"=w227, "config ref"=w228) -> ("value"=w222:string, "config ref out"=w216:T5)  [unwired: 6 in, 2 out]
              n154 = call-poly <userlib>:"manageConfig.vi"("property path"="SCS.Notification.Email alert CC", "config ref"=w216) -> ("value"=w221:string, "config ref out"=w215:T5)  [unwired: 6 in, 2 out]
              n155 = call-poly <userlib>:"manageConfig.vi"("property path"=w218, "config ref"=w215) -> ("value"=w213:bool, "config ref out"=w210:T5)  [unwired: 6 in, 2 out]
              n156 = call-poly <userlib>:"manageConfig.vi"("property path"=w211, "config ref"=w210) -> ("value"=w208:bool, "config ref out"=w209:T5)  [unwired: 6 in, 2 out]
              n157 = call-poly <userlib>:"manageConfig.vi"("property path"=w217, "config ref"=w209) -> ("value"=w212:string, "config ref out"=w214:T5)  [unwired: 6 in, 2 out]
              n158 = call-poly <userlib>:"manageConfig.vi"("config ref"=w214) -> ()  [unwired: 10 in, 1 out]
              n159 = local write "Email alert - engineer"(w222) -> ()
              n160 = local write "Phone number"(w212) -> ()
              n161 = local write "Email alert - CC"(w221) -> ()
              n162 = local write "Enable text notification"(w208) -> ()
              n163 = local write "Enable email notification"(w213) -> ()
            }
            frame #7 {
              n164 = local read "Parallelism"() -> (w231:u32)
              n165 = local read "H1 index\ntime set"() -> (w229:dbl)
              n166 = local read "H2 index\ntime set"() -> (w230:dbl)
              n167 = local write "H1 parallelism"(w231) -> ()
              n168 = local write "H2 parallelism"(w231) -> ()
              n169 = local write "H1 IT orig"(w229) -> ()
              n170 = local write "H2 IT orig"(w230) -> ()
            }
          }
        }
      }
    }
    frame #4 {
      n171 = local read "POWER"() -> (w232:bool)
      n172 = case shown="True" w232 {
        frame False {
        }
        frame True {
          w238 = "\r\n"
          n173 = local read "Data log path and filename"() -> (w233:path)
          n174 = local read "H1 online"() -> (w250:bool)
          n175 = local read "H2 online"() -> (w251:bool)
          n176 = local read "H1 UPH warning limit"() -> (w246:dbl)
          n177 = local read "H2 UPH warning limit"() -> (w248:dbl)
          n178 = local read "H2  low yield warning"() -> (w247:dbl)
          n179 = local read "H1 low yield warning"() -> (w245:dbl)
          n180 = case shown="True" w250 {
            tunnel: ["H1 Off-Line" "H1 On-Line"] -> w252
            frame False {
            }
            frame True {
            }
          }
          n181 = case shown="True" w251 {
            tunnel: ["H2 Off-Line" "H2 On-Line"] -> w257
            frame False {
            }
            frame True {
            }
          }
          n182 = local read "Operator name"() -> (w244:string)
          n183 = local read "Lot number"() -> (w242:string)
          n184 = local read "Test cell ID"() -> (w240:string)
          n185 = Number To Decimal String(number=w245) -> (decimal integer string=w254:string)  [unwired: 1 in]
          n186 = Number To Decimal String(number=w246) -> (decimal integer string=w256:string)  [unwired: 1 in]
          n187 = Number To Decimal String(number=w247) -> (decimal integer string=w259:string)  [unwired: 1 in]
          n188 = Number To Decimal String(number=w248) -> (decimal integer string=w261:string)  [unwired: 1 in]
          n189 = Get Date/Time String() -> (date string=w235:string, time string=w237:string)  [unwired: 3 in]
          n190 = Concatenate Strings(w235, "   " ("string"), w237, w238, "Test Cell ID: ", w240, w238, "Lot Number: ", w242, w238, "Operator Name:  ", w244, w238, "System Started", w238, w252, w238, "H1 Low Yield Warning Limit: ", w254, w238, "H1 Low UPH Warning Limit: ", w256, w238, w257, w238, "H2 Low Yield Warning Limit: ", w259, w238, "H2 Low UPH Warning Limit: ", w261, w238, w238) -> (w262:string)
          n191 = call "SentinelDatalog.vi"("operation (0:open)"=T4."open or create", "String"=w262, "data log path"=w233) -> ()  [unwired: 8 in, 1 out]
          n192 = local write "Email alert - attachment (not editable)"(w233) -> ()
        }
      }
    }
    frame #5 {
      n193 = local read "POWER"() -> (w267:bool)
      n194 = case shown="True" w267 {
        frame False {
        }
        frame True {
          n195 = while {
            stop <- w268 stop-if-true
            # "Sentinel operating loop\n- tester loop\n- H1 loop\n- H2 loop\n- controls loop\n- alarm state machine loop\nExit with Power off"
            n196 = local read "POWER"() -> (w269:bool)
            n197 = Not(x=w269) -> (.not. x?=w268:bool)
            n198 = Wait (ms)(milliseconds to wait=u32 100) -> ()  [unwired: 1 out]
            n199 = local read "Run / Stop"() -> (w270:bool)
            n200 = case shown="True" w270 {
              frame False {
              }
              frame True {
                w280 = 0.0
                w282 = 0.0
                w283 = 0.0
                w284 = 0.0
                w287 = 0.0
                n201 = while {
                  shift-right: [w1013] -> _
                  shift-left: FALSE ("Optimize Handler Speed") -> [w1017]
                  i -> [w1001]
                  stop <- w1052 stop-if-true
                  n202 = local read "Additional floorspace\nfor second handler"() -> (w1003:i32)
                  n203 = local read "Celerint hardware cost ($/mo)"() -> (w1006:dbl)
                  n204 = local read "Celerint licensing cost ($/mo)"() -> (w1005:dbl)
                  n205 = local read "Second handler cost ($/mo)"() -> (w1004:dbl)
                  n206 = local read "Overhead ($/mo)"() -> (w1009:dbl)
                  n207 = local read "Handler cost ($/mo)"() -> (w1010:dbl)
                  n208 = local read "Tester cost ($/mo)"() -> (w1011:dbl)
                  n209 = local read "POWER"() -> (w1055:bool)
                  n210 = local read "Std cell \nfloorspace area"() -> (w1048:i32)
                  n211 = local read "H2 index\ntime set"() -> (w1021:dbl)
                  n212 = local read "H1 index\ntime set"() -> (w1018:dbl)
                  "H1 Index Time 2" <- w1018
                  n213 = local read "Simulate at max speed"() -> (w1040:bool)
                  n214 = local read "Push to reset charts"() -> (w999:bool)
                  n215 = local read "Run / Stop"() -> (w1002:bool)
                  n216 = local read "Test time set"() -> (w1033:dbl)
                  "H1 Test Time 2" <- w1033
                  n217 = local read "Hours per month"() -> (w1008:i32)
                  "Hours per month 2" <- w1008
                  n218 = local read "Parallelism"() -> (w1032:u32)
                  "H1 parallelism" <- w1032
                  "H1 Parallelism 2" <- w1032
                  "H2 units/cycle" <- w1032
                  n219 = Not(x=w1055) -> (.not. x?=w1053:bool)
                  n220 = local read "Optimize handler speed"() -> (w1013:bool)
                  "IT lock 1" <- w1013
                  n221 = local read "Alert volume"() -> (w1012:u32)
                  n222 = Compound Arithmetic op=ADD(w1006, w1005, w1004) -> (w1038:dbl)
                  n223 = Compound Arithmetic op=ADD(w1011, w1010, w1009) -> (w1037:dbl)
                  n224 = Compound Arithmetic op=ADD(w1011, w1009) -> (→"Std mo cost ($/mo)" →"Total Mo Costs ($/mo) 2":dbl)
                  n225 = local read "H1 IT orig"() -> (w1015:dbl)
                  n226 = local read "H2 IT orig"() -> (w1016:dbl)
                  n227 = Not(x=w1002) -> (.not. x?=w1054:bool)
                  n228 = Add(x=w1003, y=w1048) -> (x+y=→"Tandem\nfloorspace area":i32)
                  n229 = Add(x=w1038, y=w1037) -> (x+y=→"Total Mo Costs ($/mo) 3":dbl)
                  n230 = Divide(x=w1038, y=w1008) -> (x/y=w1049:dbl)
                  n231 = Divide(x=w1037, y=w1008) -> (x/y=w1046:dbl)
                  "Std hourly\ncost ($/hr)" <- w1046
                  n232 = case shown="True" w999 {
                    frame False {
                    }
                    frame True {
                      w1072 = cluster{dbl, dbl}[] [] ("History Data")
                      (unwired) cluster{dbl, dbl, dbl}[] [] ("History Data")
                      n233 = property on="YieldMon" class="WFChart (strict)"("History Data"=cluster{dbl, dbl, dbl, dbl}[] []) -> ()  [unwired: 2 in, 2 out]
                      n234 = property on="Unit cost (cents/device)" class="WFChart (strict)"("History Data"=w1072) -> ()  [unwired: 2 in, 2 out]
                      n235 = property on="UPH per unit area" class="WFChart (strict)"("History Data"=w1072) -> ()  [unwired: 2 in, 2 out]
                      n236 = property on="SysUtilMon" class="WFChart (strict)"("History Data"=w1072) -> ()  [unwired: 2 in, 2 out]
                    }
                  }
                  n237 = property on="Unit cost (cents/device)" class="WFChart (strict)"("YScale.Maximum"="Cost \nupper\nlimit") -> ()  [unwired: 2 in, 2 out]
                  n238 = case shown="False" "Cost 10X" {
                    frame False {
                      n239 = property on="Cost \nupper\nlimit" class="Slide (strict)"("Scale.Maximum"=10.0 ("Scale.Range:Maximum")) -> ()  [unwired: 2 in, 2 out]
                    }
                    frame True {
                      n240 = property on="Cost \nupper\nlimit" class="Slide (strict)"("Scale.Maximum"=100.0 ("Scale.Range:Maximum")) -> ()  [unwired: 2 in, 2 out]
                    }
                  }
                  n241 = property on="UPH per unit area" class="WFChart (strict)"("YScale.Maximum"="UPH \nupper\nlimit") -> ()  [unwired: 2 in, 2 out]
                  n242 = case shown="True" "UPH 10X" {
                    frame False {
                      n243 = property on="UPH \nupper\nlimit" class="Slide (strict)"("Scale.Maximum"=100.0 ("Scale.Range:Maximum")) -> ()  [unwired: 2 in, 2 out]
                    }
                    frame True {
                      n244 = property on="UPH \nupper\nlimit" class="Slide (strict)"("Scale.Maximum"=1000.0 ("Scale.Range:Maximum")) -> ()  [unwired: 2 in, 2 out]
                    }
                  }
                  n245 = case shown="True" w1040 {
                    frame False {
                      n246 = local write "Time Accerlation  Factor"(1.0 ("Time Accerlation  Factor")) -> ()
                    }
                    frame True {
                      n247 = local read "Min Test Time"() -> (w1102:dbl)
                      n248 = local read "Test time set"() -> (w1101:dbl)
                      n249 = Divide(x=w1101, y=w1102) -> (x/y=w1100:dbl)
                      n250 = local write "Time Accerlation  Factor"(w1100) -> ()
                    }
                  }
                  n251 = Compound Arithmetic op=OR(w1053, w1054) -> (w1052:bool)
                  n252 = Add(x=w1046, y=w1049) -> (x+y=→"Tandem hourly\ncost ($/hr)":dbl)
                  n253 = Equal To 0?(x=w1012) -> (x = 0?=w1014:bool)
                  n254 = formula code="H1UPHorig=P*3600/(T+H1ITorig);\nH2UPHorig=P*3600/(T+H2ITorig);\nSYSH1WT=T-H1I;\nSYSH2WT=T-H2I;"("T"=w1033, "H1I"=w1018, "H2I"=w1021, "P"=w1032, "H1ITorig"=w1015, "H2ITorig"=w1016) -> ("H1UPHorig"=→"H1 calc UPH" →"H1 calc UPH":dbl, "H2UPHorig"=→"H2 calc UPH":dbl, "SYSH1WT"=w1025:dbl, "SYSH2WT"=w1024:dbl)
                  n255 = case shown="True" w1014 {
                    frame False {
                    }
                    frame True {
                      n256 = local write "Audio On / Off"(FALSE ("Audio On/Off")) -> ()
                    }
                  }
                  n257 = case shown="False" w1013 {
                    selector: w1013 -> [w1076 _]
                    tunnel: w1017 -> [w1080 _]
                    frame False {
                      n258 = Equal?(x=w1080, y=TRUE) -> (x = y?=w1078:bool)
                      n259 = Equal?(x=FALSE, y=w1076) -> (x = y?=w1077:bool)
                      n260 = And(x=w1078, y=w1077) -> (x .and. y?=w1074:bool)
                      n261 = case shown="False" w1074 {
                        frame False {
                          n262 = local read "H2 index\ntime set"() -> (w1081:dbl)
                          n263 = local read "H1 index\ntime set"() -> (w1082:dbl)
                          n264 = local write "H2 IT orig"(w1081) -> ()
                          n265 = local write "H1 IT orig"(w1082) -> ()
                        }
                        frame True {
                          n266 = local read "H1 IT orig"() -> (w1084:dbl)
                          n267 = local read "H2 IT orig"() -> (w1083:dbl)
                          n268 = local write "H1 index\ntime set"(w1084) -> ()
                          n269 = local write "H2 index\ntime set"(w1083) -> ()
                        }
                      }
                    }
                    frame True {
                      n270 = local read "Test time set"() -> (w1089:dbl)
                      n271 = local read "Test time set"() -> (w1087:dbl)
                      n272 = local read "H1 IT orig"() -> (w1088:dbl)
                      n273 = local read "H2 IT orig"() -> (w1085:dbl)
                      n274 = Greater Or Equal?(x=w1089, y=w1088) -> (x >= y?=w1090:bool)
                      n275 = Greater Or Equal?(x=w1087, y=w1085) -> (x >= y?=w1086:bool)
                      n276 = case shown="False" w1090 {
                        frame False {
                          n277 = local read "H1 IT orig"() -> (w1095:dbl)
                          n278 = local write "H1 index\ntime set"(w1095) -> ()
                        }
                        frame True {
                          n279 = local read "Test time set"() -> (w1098:dbl)
                          n280 = Multiply(x=w1098, y=0.95) -> (x*y=w1096:dbl)
                          n281 = local write "H1 index\ntime set"(w1096) -> ()
                        }
                      }
                      n282 = case shown="False" w1086 {
                        frame False {
                          n283 = local read "H2 IT orig"() -> (w1091:dbl)
                          n284 = local write "H2 index\ntime set"(w1091) -> ()
                        }
                        frame True {
                          n285 = local read "Test time set"() -> (w1094:dbl)
                          n286 = Multiply(x=w1094, y=0.95) -> (x*y=w1092:dbl)
                          n287 = local write "H2 index\ntime set"(w1092) -> ()
                        }
                      }
                    }
                  }
                  n288 = Less Than 0?(x=w1025) -> (x < 0?=w1026:bool)
                  n289 = Less Than 0?(x=w1024) -> (x < 0?=w1027:bool)
                  n290 = local read "Test time set"() -> (w1042:dbl)
                  n291 = Equal To 0?(x=w1001) -> (x = 0?=w1000:bool)
                  n292 = case shown="True" w1000 {
                    frame False {
                    }
                    frame True {
                      w1103 = 0
                      w1105 = cluster{dbl, dbl}[] [] ("History Data")
                      w1106 = 0
                      w1119 = cluster{dbl, dbl} {0.0, 0.0}
                      w1121 = 100
                      w1123 = 0
                      w1124 = FALSE ("H1 alarm")
                      # "graphs and charts - declared here, displayed elsewhere"
                      n293 = Bundle(w1121, w1121, w1121, w1121) -> (→"YieldMon":cluster{i32, i32, i32, i32})  [unwired: 1 in]
                      n294 = Bundle(w1123, w1123) -> (→"SysUtilMon":cluster{i32, i32})  [unwired: 1 in]
                      n295 = local write "H2 warning 2"(FALSE ("H1 warning")) -> ()
                      n296 = local write "H1 alarm"(FALSE ("H1 warning")) -> ()
                      n297 = local write "H2 nominal 2"(TRUE ("H1 nominal")) -> ()
                      n298 = local write "H2 alarm 2"(FALSE ("H1 warning")) -> ()
                      n299 = local write "H2 nominal"(TRUE ("H1 nominal")) -> ()
                      n300 = local write "H2 alarm"(FALSE ("H1 warning")) -> ()
                      n301 = local write "H1 nominal 2"(TRUE ("H1 nominal")) -> ()
                      n302 = local write "H1 alarm 2"(FALSE ("H1 warning")) -> ()
                      n303 = local write "H2 warning"(FALSE ("H1 warning")) -> ()
                      n304 = local write "H1 nominal"(TRUE ("H1 nominal")) -> ()
                      n305 = local write "H1 warning 2"(FALSE ("H1 warning")) -> ()
                      n306 = local write "H1 warning"(FALSE ("H1 warning")) -> ()
                      n307 = property on="YieldMon" class="WFChart (strict)"("History Data"=cluster{dbl, dbl, dbl, dbl}[] []) -> ()  [unwired: 2 in, 2 out]
                      n308 = property on="SysUtilMon" class="WFChart (strict)"("History Data"=w1105) -> ()  [unwired: 2 in, 2 out]
                      n309 = local write "system statuts"(T2."H1NH2N" ("system statuts")) -> ()
                      n310 = local write "H1 alarm"(w1124) -> ()
                      n311 = local write "H2 alarm"(w1124) -> ()
                      n312 = local write "H2 Good Units"(w1106) -> ()
                      n313 = local write "H1 Device Count"(w1106) -> ()
                      n314 = local write "H1 Good Units"(w1106) -> ()
                      n315 = local write "H2 Device Count"(w1106) -> ()
                      n316 = property on="UPH per unit area" class="WFChart (strict)"("History Data"=w1105) -> ()  [unwired: 2 in, 2 out]
                      n317 = property on="Unit cost (cents/device)" class="WFChart (strict)"("History Data"=w1105) -> ()  [unwired: 2 in, 2 out]
                      n318 = local write "H2 alarm 2"(w1124) -> ()
                      n319 = local write "H1 alarm 2"(w1124) -> ()
                      n320 = property on="System UPH" class="Knob (strict)"("Scale.Minimum"=w1103) -> ()  [unwired: 2 in, 2 out]
                      n321 = property on="H1 UPH" class="Knob (strict)"("Scale.Minimum"=w1103) -> ()  [unwired: 2 in, 2 out]
                      n322 = property on="H2 UPH" class="Knob (strict)"("Scale.Minimum"=w1103) -> ()  [unwired: 2 in, 2 out]
                      "Sys utilization" <- 0.0
                      "UPH per unit area" <- w1119
                      "Unit cost (cents/device)" <- w1119
                    }
                  }
                  n323 = Select(t=0.0, s=w1026, f=w1025) -> (s? t:f=w1020:dbl)
                  n324 = Select(t=0.0, s=w1027, f=w1024) -> (s? t:f=w1019:dbl)
                  n325 = formula code="ExpH1UPH=P*3600/(T+SYSH1I+SYSH1WT);\nExpH2UPH=P*3600/(T+SYSH2I+SYSH2WT);\nMaxUPH=Margin*(ExpH1UPH+ExpH2UPH);"("P"=w1032, "T"=w1042, "SYSH1I"=w1018, "SYSH2I"=w1021, "Margin"=1.05 ("input variable"), "SYSH1WT"=w1020, "SYSH2WT"=w1019) -> ("MaxUPH"=w1043:dbl, "ExpH1UPH"=w1023:dbl, "ExpH2UPH"=w1022:dbl)
                  n326 = property on="System UPH" class="Knob (strict)"("Scale.Maximum"=w1043) -> ()  [unwired: 2 in, 2 out]
                  n327 = property on="H1 UPH" class="Knob (strict)"("Scale.Maximum"=w1023) -> ()  [unwired: 2 in, 2 out]
                  n328 = property on="H2 UPH" class="Knob (strict)"("Scale.Maximum"=w1022) -> ()  [unwired: 2 in, 2 out]
                  n329 = local read "Optimize handler speed"() -> (w998:bool)
                  n330 = local read "Std cell \nfloorspace area"() -> (→"Std cell floorspace area":i32)
                  n331 = Wait (ms)(milliseconds to wait=u32 200) -> ()  [unwired: 1 out]
                  n332 = case shown="True" w998 {
                    frame False {
                    }
                    frame True {
                      w1065 = FALSE
                      n333 = local read "H1 online"() -> (w1067:bool)
                      n334 = local read "H2 online"() -> (w1066:bool)
                      n335 = Equal?(x=w1067, y=w1065) -> (x = y?=w1069:bool)
                      n336 = Equal?(x=w1065, y=w1066) -> (x = y?=w1068:bool)
                      n337 = Or(x=w1069, y=w1068) -> (x .or. y?=w1064:bool)
                      n338 = case shown="True" w1064 {
                        frame False {
                        }
                        frame True {
                          n339 = local write "Optimize handler speed"(FALSE ("Optimize Handler Speed")) -> ()
                        }
                      }
                    }
                  }
                  n340 = local read "H1 online"() -> (w997:bool)
                  n341 = local read "H2 online"() -> (w996:bool)
                  n342 = Not(x=w996) -> (.not. x?=w993:bool)
                  "H2 On/Off-line" <- w993
                  n343 = Not(x=w997) -> (.not. x?=w994:bool)
                  "H1 On/Off-line" <- w994
                  n344 = And(x=w994, y=w993) -> (x .and. y?=w995:bool)
                  n345 = case shown="True" w994 {
                    frame False {
                    }
                    frame True {
                      n346 = local write "H1 nominal"(TRUE) -> ()
                      n347 = local write "H1 warning"(TRUE) -> ()
                      n348 = local write "H1 alarm"(TRUE) -> ()
                    }
                  }
                  n349 = case shown="True" w993 {
                    frame False {
                    }
                    frame True {
                      n350 = local write "H2 warning"(TRUE) -> ()
                      n351 = local write "H2 nominal"(TRUE) -> ()
                      n352 = local write "H2 alarm"(TRUE) -> ()
                    }
                  }
                  n353 = case shown="True" w995 {
                    frame False {
                    }
                    frame True {
                      n354 = local write "Sys utilization"(0.0 ("Sys utilization")) -> ()
                      n355 = local write "System UPH"(u32 0 ("System UPH")) -> ()
                    }
                  }
                }
                n356 = local read "UPH averaging"() -> (w276:u32)
                n357 = local read "Yield averaging"() -> (w275:u32)
                n358 = Initialize Array(w284, w276) -> (w286:dbl[])
                n359 = Initialize Array(w282, w275) -> (w281:dbl[])
                n360 = while {
                  shift-right: [w412] -> _
                  shift-left: T2."H1NH2N" ("system statuts") -> [w411]
                  stop <- w415 stop-if-true
                  # "System Status Handler"
                  n361 = local read "Run / Stop"() -> (w413:bool)
                  n362 = local read "H1 Device Count"() -> (w410:u32)
                  n363 = local read "H2 Device Count"() -> (w409:u32)
                  n364 = local read "POWER"() -> (w416:bool)
                  n365 = Add(x=w410, y=w409) -> (x+y=w408:u32)
                  n366 = Not(x=w416) -> (.not. x?=w418:bool)
                  n367 = Not(x=w413) -> (.not. x?=w417:bool)
                  n368 = local read "Parallelism"() -> (w407:u32)
                  n369 = Compound Arithmetic op=OR(w418, w417) -> (w415:bool)
                  n370 = Divide(x=w408, y=w407) -> (x/y=w406:dbl)
                  n371 = local read "Ignore alarms until AFTER this many cycles"() -> (w405:i32)
                  n372 = Greater?(x=w406, y=w405) -> (0:w404:bool)
                  n373 = case shown="True" w404 {
                    tunnel: [w419 w421] -> w412
                    tunnel: w411 -> [w419 w420]
                    frame False {
                    }
                    frame True {
                      n374 = flat-sequence {
                        tunnel: [w517] -> w421
                        tunnel: w420 -> [w518]
                        frame #0 {
                          # "Determine current state for System Status state-machine"
                          n375 = stacked-sequence {
                            frame #0 {
                              n376 = local read "H1 nominal 2"() -> (w425:bool)
                              n377 = local read "H2 nominal 2"() -> (w423:bool)
                              n378 = local read "H1 nominal"() -> (w426:bool)
                              n379 = local read "H2 nominal"() -> (w424:bool)
                              n380 = Compound Arithmetic op=AND(w426, w425, w424, w423) -> (w422:bool)
                              n381 = case shown="True" w422 {
                                frame False {
                                }
                                frame True {
                                n382 = local write "system statuts"(T2."H1NH2N" ("system statuts")) -> ()
                                }
                              }
                            }
                            frame #1 {
                              n383 = local read "H2 warning 2"() -> (w430:bool)
                              n384 = local read "H2 warning"() -> (w431:bool)
                              n385 = local read "H1 nominal 2"() -> (w432:bool)
                              n386 = local read "H1 nominal"() -> (w433:bool)
                              n387 = Or(x=w431, y=w430) -> (x .or. y?=w429:bool)
                              n388 = Compound Arithmetic op=AND(w433, w432, w429) -> (w428:bool)
                              n389 = case shown="False" w428 {
                                frame False {
                                }
                                frame True {
                                n390 = local write "system statuts"(T2."H1NH2W" ("system statuts")) -> ()
                                }
                              }
                            }
                            frame #2 {
                              n391 = local read "H1 nominal 2"() -> (w440:bool)
                              n392 = local read "H1 nominal"() -> (w441:bool)
                              n393 = local read "H2 alarm 2"() -> (w438:bool)
                              n394 = local read "H2 alarm"() -> (w439:bool)
                              n395 = Or(x=w439, y=w438) -> (x .or. y?=w436:bool)
                              n396 = And(x=w441, y=w440) -> (x .and. y?=w437:bool)
                              n397 = And(x=w437, y=w436) -> (x .and. y?=w435:bool)
                              n398 = case shown="True" w435 {
                                frame False {
                                }
                                frame True {
                                n399 = local write "system statuts"(T2."H1NH2A" ("system statuts")) -> ()
                                }
                              }
                            }
                            frame #3 {
                              n400 = local read "H1 alarm 2"() -> (w451:bool)
                              n401 = local read "H1 alarm"() -> (w452:bool)
                              n402 = local read "H2 nominal 2"() -> (w454:bool)
                              n403 = local read "H1 warning 2"() -> (w447:bool)
                              n404 = local read "H1 warning"() -> (w448:bool)
                              n405 = local read "H2 nominal"() -> (w453:bool)
                              n406 = Not(x=w452) -> (.not. x?=w450:bool)
                              n407 = Not(x=w451) -> (.not. x?=w449:bool)
                              n408 = Or(x=w448, y=w447) -> (x .or. y?=w445:bool)
                              n409 = And(x=w450, y=w449) -> (x .and. y?=w444:bool)
                              n410 = And(x=w453, y=w454) -> (x .and. y?=w443:bool)
                              n411 = Compound Arithmetic op=AND(w445, w444, w443) -> (w446:bool)
                              n412 = case shown="True" w446 {
                                frame False {
                                }
                                frame True {
                                n413 = local write "system statuts"(T2."H1WH2N" ("system statuts")) -> ()
                                }
                              }
                            }
                            frame #4 {
                              n414 = local read "H1 alarm 2"() -> (w466:bool)
                              n415 = local read "H2 alarm 2"() -> (w471:bool)
                              n416 = local read "H1 alarm"() -> (w465:bool)
                              n417 = local read "H2 alarm"() -> (w472:bool)
                              n418 = local read "H1 warning 2"() -> (w462:bool)
                              n419 = local read "H2 warning 2"() -> (w463:bool)
                              n420 = local read "H1 warning"() -> (w461:bool)
                              n421 = local read "H2 warning"() -> (w464:bool)
                              n422 = Not(x=w465) -> (.not. x?=w467:bool)
                              n423 = Not(x=w466) -> (.not. x?=w468:bool)
                              n424 = Not(x=w472) -> (.not. x?=w470:bool)
                              n425 = Not(x=w471) -> (.not. x?=w469:bool)
                              n426 = Or(x=w461, y=w462) -> (x .or. y?=w459:bool)
                              n427 = Or(x=w464, y=w463) -> (x .or. y?=w457:bool)
                              n428 = And(x=w467, y=w468) -> (x .and. y?=w458:bool)
                              n429 = And(x=w470, y=w469) -> (x .and. y?=w456:bool)
                              n430 = Compound Arithmetic op=AND(w459, w458, w457, w456) -> (w460:bool)
                              n431 = case shown="True" w460 {
                                frame False {
                                }
                                frame True {
                                n432 = local write "system statuts"(T2."H1WH2W" ("system statuts")) -> ()
                                }
                              }
                            }
                            frame #5 {
                              n433 = local read "H1 alarm 2"() -> (w479:bool)
                              n434 = local read "H1 alarm"() -> (w480:bool)
                              n435 = local read "H1 warning 2"() -> (w482:bool)
                              n436 = local read "H1 warning"() -> (w483:bool)
                              n437 = local read "H2 alarm 2"() -> (w484:bool)
                              n438 = local read "H2 alarm"() -> (w485:bool)
                              n439 = Not(x=w480) -> (.not. x?=w478:bool)
                              n440 = Not(x=w479) -> (.not. x?=w477:bool)
                              n441 = Or(x=w483, y=w482) -> (x .or. y?=w476:bool)
                              n442 = Or(x=w485, y=w484) -> (x .or. y?=w474:bool)
                              n443 = And(x=w478, y=w477) -> (x .and. y?=w475:bool)
                              n444 = Compound Arithmetic op=AND(w476, w475, w474) -> (w481:bool)
                              n445 = case shown="True" w481 {
                                frame False {
                                }
                                frame True {
                                n446 = local write "system statuts"(T2."H1WH2A" ("system statuts")) -> ()
                                }
                              }
                            }
                            frame #6 {
                              n447 = local read "H2 nominal 2"() -> (w492:bool)
                              n448 = local read "H2 nominal"() -> (w493:bool)
                              n449 = local read "H1 alarm 2"() -> (w490:bool)
                              n450 = local read "H1 alarm"() -> (w491:bool)
                              n451 = Or(x=w491, y=w490) -> (x .or. y?=w488:bool)
                              n452 = And(x=w493, y=w492) -> (x .and. y?=w487:bool)
                              n453 = And(x=w488, y=w487) -> (x .and. y?=w489:bool)
                              n454 = case shown="True" w489 {
                                frame False {
                                }
                                frame True {
                                n455 = local write "system statuts"(T2."H1AH2N" ("system statuts")) -> ()
                                }
                              }
                            }
                            frame #7 {
                              n456 = local read "H2 alarm 2"() -> (w497:bool)
                              n457 = local read "H2 alarm"() -> (w498:bool)
                              n458 = local read "H2 warning 2"() -> (w503:bool)
                              n459 = local read "H2 warning"() -> (w504:bool)
                              n460 = local read "H1 alarm 2"() -> (w505:bool)
                              n461 = local read "H1 alarm"() -> (w506:bool)
                              n462 = Not(x=w498) -> (.not. x?=w496:bool)
                              n463 = Not(x=w497) -> (.not. x?=w495:bool)
                              n464 = Or(x=w506, y=w505) -> (x .or. y?=w501:bool)
                              n465 = Or(x=w504, y=w503) -> (x .or. y?=w500:bool)
                              n466 = And(x=w496, y=w495) -> (x .and. y?=w499:bool)
                              n467 = Compound Arithmetic op=AND(w501, w500, w499) -> (w502:bool)
                              n468 = case shown="True" w502 {
                                frame False {
                                }
                                frame True {
                                n469 = local write "system statuts"(T2."H1AH2W" ("system statuts")) -> ()
                                }
                              }
                            }
                            frame #8 {
                              n470 = local read "H1 alarm 2"() -> (w512:bool)
                              n471 = local read "H2 alarm 2"() -> (w511:bool)
                              n472 = local read "H1 alarm"() -> (w513:bool)
                              n473 = local read "H2 alarm"() -> (w510:bool)
                              n474 = Or(x=w513, y=w512) -> (x .or. y?=w508:bool)
                              n475 = Or(x=w510, y=w511) -> (x .or. y?=w509:bool)
                              n476 = And(x=w508, y=w509) -> (x .and. y?=w514:bool)
                              n477 = case shown="True" w514 {
                                frame False {
                                }
                                frame True {
                                n478 = local write "system statuts"(T2."H1AH2A" ("system statuts")) -> ()
                                }
                              }
                            }
                          }
                        }
                        frame #1 {
                          n479 = local read "system statuts"() -> (w517:T2)
                          n480 = Not Equal?(x=w517, y=w518) -> (x != y?=w516:bool)
                          n481 = case shown="True" w516 {
                            tunnel: w517 -> [_ w520]
                            frame False {
                            }
                            frame True {
                              n482 = local read "Enable data logging of all events"() -> (w519:bool)
                              n483 = case shown="True" w519 {
                                tunnel: w520 -> [_ w521]
                                frame False {
                                }
                                frame True {
                                n484 = stacked-sequence {
                                tunnel: w521 -> [w522 _ _ _]
                                frame #0 {
                                n485 = case shown="\"H1NH2N\", Default" w522 {
                                frame "H1NH2N", Default {
                                w525 = "\r\n"
                                n486 = local read "H1 online"() -> (w546:bool)
                                n487 = local read "H2 online"() -> (w547:bool)
                                n488 = local read "H1 Yield Guage"() -> (w535:cluster{dbl, dbl})
                                n489 = local read "H2 Yield Guage"() -> (w533:cluster{dbl, dbl})
                                n490 = local read "H1 UPH warning limit"() -> (w542:dbl)
                                n491 = local read "H2 UPH warning limit"() -> (w544:dbl)
                                n492 = local read "H2  low yield warning"() -> (w543:dbl)
                                n493 = local read "H1 low yield warning"() -> (w541:dbl)
                                n494 = local read "H1 UPH"() -> (w531:cluster{u32, u32})
                                n495 = local read "H2 UPH"() -> (w529:cluster{u32, u32})
                                n496 = local read "Number of email alerts"() -> (w523:dbl)
                                n497 = case shown="True" w546 {
                                tunnel: ["H1 Off-Line" "H1 On-Line"] -> w548
                                frame False {
                                }
                                frame True {
                                }
                                }
                                n498 = case shown="True" w547 {
                                tunnel: ["H2 Off-Line" "H2 On-Line"] -> w557
                                frame False {
                                }
                                frame True {
                                }
                                }
                                n499 = Unbundle(w535) -> (w534:dbl)  [unwired: 1 out]
                                n500 = Unbundle(w531) -> (w530:u32)  [unwired: 1 out]
                                n501 = Unbundle(w533) -> (w532:dbl)  [unwired: 1 out]
                                n502 = Unbundle(w529) -> (w528:u32)  [unwired: 1 out]
                                n503 = local read "Data log path and filename"() -> (w527:path)
                                n504 = Number To Decimal String(number=w541) -> (decimal integer string=w550:string)  [unwired: 1 in]
                                n505 = Number To Decimal String(number=w534) -> (decimal integer string=w552:string)  [unwired: 1 in]
                                n506 = Number To Decimal String(number=w542) -> (decimal integer string=w554:string)  [unwired: 1 in]
                                n507 = Number To Decimal String(number=w530) -> (decimal integer string=w556:string)  [unwired: 1 in]
                                n508 = Number To Decimal String(number=w543) -> (decimal integer string=w559:string)  [unwired: 1 in]
                                n509 = Number To Decimal String(number=w532) -> (decimal integer string=w561:string)  [unwired: 1 in]
                                n510 = Number To Decimal String(number=w544) -> (decimal integer string=w563:string)  [unwired: 1 in]
                                n511 = Number To Decimal String(number=w528) -> (decimal integer string=w565:string)  [unwired: 1 in]
                                n512 = Number To Decimal String(number=w523) -> (decimal integer string=w524:string)  [unwired: 1 in]
                                n513 = Get Date/Time String(want seconds? (F)=TRUE) -> (date string=w539:string, time string=w540:string)  [unwired: 2 in]
                                n514 = Concatenate Strings(w524, w525, w539, "   " ("string"), w540, w525, "H1 Nominal, H2 Nominal", w525, w548, w525, "H1 Low Yield Warning Limit: ", w550, ", H1 yield = ", w552, w525, "H1 Low UPH Warning Limit: ", w554, ", H1 UPH = ", w556, w525, w557, w525, "H2 Low Yield Warning Limit: ", w559, ", H2 yield = ", w561, w525, "H2 Low UPH Warning Limit: ", w563, ", H2 UPH = ", w565, w525, w525) -> (w537:string)
                                n515 = call "SentinelDatalog.vi"("operation (0:open)"=T4."open", "String"=w537, "data log path"=w527) -> ()  [unwired: 8 in, 1 out]
                                }
                                frame "H1NH2W" {
                                w570 = "\r\n"
                                n516 = local read "H1 online"() -> (w593:bool)
                                n517 = local read "H2 online"() -> (w594:bool)
                                n518 = local read "H1 Yield Guage"() -> (w582:cluster{dbl, dbl})
                                n519 = local read "H2 Yield Guage"() -> (w580:cluster{dbl, dbl})
                                n520 = local read "H1 UPH warning limit"() -> (w589:dbl)
                                n521 = local read "H2 UPH warning limit"() -> (w591:dbl)
                                n522 = local read "H2  low yield warning"() -> (w590:dbl)
                                n523 = local read "H1 low yield warning"() -> (w588:dbl)
                                n524 = local read "H1 UPH"() -> (w578:cluster{u32, u32})
                                n525 = local read "H2 UPH"() -> (w576:cluster{u32, u32})
                                n526 = local read "Number of email alerts"() -> (w572:dbl)
                                n527 = case shown="True" w593 {
                                tunnel: ["H1 Off-Line" "H1 On-Line"] -> w595
                                frame False {
                                }
                                frame True {
                                }
                                }
                                n528 = case shown="True" w594 {
                                tunnel: ["H2 Off-Line" "H2 On-Line"] -> w604
                                frame False {
                                }
                                frame True {
                                }
                                }
                                n529 = Unbundle(w582) -> (w581:dbl)  [unwired: 1 out]
                                n530 = Unbundle(w578) -> (w577:u32)  [unwired: 1 out]
                                n531 = Unbundle(w580) -> (w579:dbl)  [unwired: 1 out]
                                n532 = Unbundle(w576) -> (w575:u32)  [unwired: 1 out]
                                n533 = Number To Decimal String(number=w588) -> (decimal integer string=w597:string)  [unwired: 1 in]
                                n534 = Number To Decimal String(number=w581) -> (decimal integer string=w599:string)  [unwired: 1 in]
                                n535 = Number To Decimal String(number=w589) -> (decimal integer string=w601:string)  [unwired: 1 in]
                                n536 = Number To Decimal String(number=w577) -> (decimal integer string=w603:string)  [unwired: 1 in]
                                n537 = Number To Decimal String(number=w590) -> (decimal integer string=w606:string)  [unwired: 1 in]
                                n538 = Number To Decimal String(number=w579) -> (decimal integer string=w608:string)  [unwired: 1 in]
                                n539 = Number To Decimal String(number=w591) -> (decimal integer string=w610:string)  [unwired: 1 in]
                                n540 = Number To Decimal String(number=w575) -> (decimal integer string=w612:string)  [unwired: 1 in]
                                n541 = Number To Decimal String(number=w572) -> (decimal integer string=w571:string)  [unwired: 1 in]
                                n542 = local read "Data log path and filename"() -> (w574:path)
                                n543 = Get Date/Time String(want seconds? (F)=TRUE) -> (date string=w586:string, time string=w587:string)  [unwired: 2 in]
                                n544 = Concatenate Strings(w571, w570, w586, "   " ("string"), w587, w570, "H1 Nominal, H2 Warning", w570, w595, w570, "H1 Low Yield Warning Limit: ", w597, ", H1 yield = ", w599, w570, "H1 Low UPH Warning Limit: ", w601, ", H1 UPH = ", w603, w570, w604, w570, "H2 Low Yield Warning Limit: ", w606, ", H2 yield = ", w608, w570, "H2 Low UPH Warning Limit: ", w610, ", H2 UPH = ", w612, w570, w570) -> (w584:string)
                                n545 = call "SentinelDatalog.vi"("operation (0:open)"=T4."open", "String"=w584, "data log path"=w574) -> ()  [unwired: 8 in, 1 out]
                                }
                                frame "H1NH2A" {
                                w618 = "\r\n"
                                n546 = local read "H1 online"() -> (w640:bool)
                                n547 = local read "H2 online"() -> (w641:bool)
                                n548 = local read "H1 Yield Guage"() -> (w629:cluster{dbl, dbl})
                                n549 = local read "H2 Yield Guage"() -> (w628:cluster{dbl, dbl})
                                n550 = local read "Number of email alerts"() -> (w619:dbl)
                                n551 = local read "H1 UPH warning limit"() -> (w636:dbl)
                                n552 = local read "H1 low yield warning"() -> (w635:dbl)
                                n553 = local read "H2 UPH alarm limit"() -> (w638:dbl)
                                n554 = local read "H1 UPH"() -> (w627:cluster{u32, u32})
                                n555 = local read "H2 low yield alarm"() -> (w637:dbl)
                                n556 = local read "H2 UPH"() -> (w626:cluster{u32, u32})
                                n557 = case shown="True" w640 {
                                tunnel: ["H1 Off-Line" "H1 On-Line"] -> w642
                                frame False {
                                }
                                frame True {
                                }
                                }
                                n558 = case shown="True" w641 {
                                tunnel: ["H2 Off-Line" "H2 On-Line"] -> w651
                                frame False {
                                }
                                frame True {
                                }
                                }
                                n559 = Number To Decimal String(number=w619) -> (decimal integer string=w617:string)  [unwired: 1 in]
                                n560 = Unbundle(w629) -> (w622:dbl)  [unwired: 1 out]
                                n561 = Unbundle(w627) -> (w623:u32)  [unwired: 1 out]
                                n562 = Unbundle(w628) -> (w624:dbl)  [unwired: 1 out]
                                n563 = Unbundle(w626) -> (w625:u32)  [unwired: 1 out]
                                n564 = Number To Decimal String(number=w635) -> (decimal integer string=w644:string)  [unwired: 1 in]
                                n565 = Number To Decimal String(number=w622) -> (decimal integer string=w646:string)  [unwired: 1 in]
                                n566 = Number To Decimal String(number=w636) -> (decimal integer string=w648:string)  [unwired: 1 in]
                                n567 = Number To Decimal String(number=w623) -> (decimal integer string=w650:string)  [unwired: 1 in]
                                n568 = Number To Decimal String(number=w637) -> (decimal integer string=w653:string)  [unwired: 1 in]
                                n569 = Number To Decimal String(number=w624) -> (decimal integer string=w655:string)  [unwired: 1 in]
                                n570 = Number To Decimal String(number=w638) -> (decimal integer string=w657:string)  [unwired: 1 in]
                                n571 = Number To Decimal String(number=w625) -> (decimal integer string=w659:string)  [unwired: 1 in]
                                n572 = local read "Data log path and filename"() -> (w621:path)
                                n573 = Get Date/Time String(want seconds? (F)=TRUE) -> (date string=w633:string, time string=w634:string)  [unwired: 2 in]
                                n574 = Concatenate Strings(w617, w618, w633, "   " ("string"), w634, w618, "H1 Nominal, H2 Alarming", w618, w642, w618, "H1 Low Yield Warning Limit: ", w644, ", H1 yield = ", w646, w618, "H1 Low UPH Warning Limit: ", w648, ", H1 UPH = ", w650, w618, w651, w618, "H2 Low Yield Alarm Limit: ", w653, ", H2 yield = ", w655, w618, "H2 Low UPH Alarm Limit: ", w657, ", H2 UPH = ", w659, w618, w618) -> (w631:string)
                                n575 = call "SentinelDatalog.vi"("operation (0:open)"=T4."open", "String"=w631, "data log path"=w621) -> ()  [unwired: 8 in, 1 out]
                                }
                                frame "H1WH2N" {
                                w666 = "\r\n"
                                n576 = local read "H1 online"() -> (w688:bool)
                                n577 = local read "H2 online"() -> (w689:bool)
                                n578 = local read "H1 Yield Guage"() -> (w676:cluster{dbl, dbl})
                                n579 = local read "H2 Yield Guage"() -> (w675:cluster{dbl, dbl})
                                n580 = local read "H1 UPH warning limit"() -> (w684:dbl)
                                n581 = local read "H2 UPH warning limit"() -> (w686:dbl)
                                n582 = local read "H2  low yield warning"() -> (w685:dbl)
                                n583 = local read "H1 low yield warning"() -> (w683:dbl)
                                n584 = local read "H1 UPH"() -> (w674:cluster{u32, u32})
                                n585 = local read "H2 UPH"() -> (w673:cluster{u32, u32})
                                n586 = case shown="True" w688 {
                                tunnel: ["H1 Off-Line" "H1 On-Line"] -> w677
                                frame False {
                                }
                                frame True {
                                }
                                }
                                n587 = case shown="True" w689 {
                                tunnel: ["H2 Off-Line" "H2 On-Line"] -> w698
                                frame False {
                                }
                                frame True {
                                }
                                }
                                n588 = local read "Number of email alerts"() -> (w665:dbl)
                                n589 = Unbundle(w676) -> (w669:dbl)  [unwired: 1 out]
                                n590 = Unbundle(w674) -> (w670:u32)  [unwired: 1 out]
                                n591 = Unbundle(w675) -> (w671:dbl)  [unwired: 1 out]
                                n592 = Unbundle(w673) -> (w672:u32)  [unwired: 1 out]
                                n593 = Number To Decimal String(number=w683) -> (decimal integer string=w691:string)  [unwired: 1 in]
                                n594 = Number To Decimal String(number=w669) -> (decimal integer string=w693:string)  [unwired: 1 in]
                                n595 = Number To Decimal String(number=w684) -> (decimal integer string=w695:string)  [unwired: 1 in]
                                n596 = Number To Decimal String(number=w670) -> (decimal integer string=w697:string)  [unwired: 1 in]
                                n597 = Number To Decimal String(number=w685) -> (decimal integer string=w700:string)  [unwired: 1 in]
                                n598 = Number To Decimal String(number=w671) -> (decimal integer string=w702:string)  [unwired: 1 in]
                                n599 = Number To Decimal String(number=w686) -> (decimal integer string=w704:string)  [unwired: 1 in]
                                n600 = Number To Decimal String(number=w672) -> (decimal integer string=w706:string)  [unwired: 1 in]
                                n601 = local read "Data log path and filename"() -> (w668:path)
                                n602 = Number To Decimal String(number=w665) -> (decimal integer string=w664:string)  [unwired: 1 in]
                                n603 = Get Date/Time String(want seconds? (F)=TRUE) -> (date string=w681:string, time string=w682:string)  [unwired: 2 in]
                                n604 = Concatenate Strings(w664, w666, w681, "   " ("string"), w682, w666, "H1 Warning, H2 Nominal", w666, w677, w666, "H1 Low Yield Warning Limit: ", w691, ", H1 yield = ", w693, w666, "H1 Low UPH Warning Limit: ", w695, ", H1 UPH = ", w697, w666, w698, w666, "H2 Low Yield Warning Limit: ", w700, ", H2 yield = ", w702, w666, "H2 Low UPH Warning Limit: ", w704, ", H2 UPH = ", w706, w666, w666) -> (w679:string)
                                n605 = call "SentinelDatalog.vi"("operation (0:open)"=T4."open", "String"=w679, "data log path"=w668) -> ()  [unwired: 8 in, 1 out]
                                }
                                frame "H1WH2W" {
                                w711 = "\r\n"
                                w724 = "\r\n"
                                n606 = local read "H1 online"() -> (w735:bool)
                                n607 = local read "H2 online"() -> (w736:bool)
                                n608 = local read "H1 Yield Guage"() -> (w723:cluster{dbl, dbl})
                                n609 = local read "H2 Yield Guage"() -> (w722:cluster{dbl, dbl})
                                n610 = local read "H1 UPH warning limit"() -> (w731:dbl)
                                n611 = local read "H2 UPH warning limit"() -> (w733:dbl)
                                n612 = local read "H2  low yield warning"() -> (w732:dbl)
                                n613 = local read "H1 low yield warning"() -> (w730:dbl)
                                n614 = local read "H1 UPH"() -> (w721:cluster{u32, u32})
                                n615 = local read "H2 UPH"() -> (w720:cluster{u32, u32})
                                n616 = case shown="True" w735 {
                                tunnel: ["H1 Off-Line" "H1 On-Line"] -> w737
                                frame False {
                                }
                                frame True {
                                }
                                }
                                n617 = case shown="True" w736 {
                                tunnel: ["H2 Off-Line" "H2 On-Line"] -> w746
                                frame False {
                                }
                                frame True {
                                }
                                }
                                n618 = Unbundle(w723) -> (w719:dbl)  [unwired: 1 out]
                                n619 = Unbundle(w721) -> (w718:u32)  [unwired: 1 out]
                                n620 = Unbundle(w722) -> (w717:dbl)  [unwired: 1 out]
                                n621 = Unbundle(w720) -> (w716:u32)  [unwired: 1 out]
                                n622 = local read "Number of email alerts"() -> (w713:dbl)
                                n623 = Number To Decimal String(number=w730) -> (decimal integer string=w739:string)  [unwired: 1 in]
                                n624 = Number To Decimal String(number=w719) -> (decimal integer string=w741:string)  [unwired: 1 in]
                                n625 = Number To Decimal String(number=w731) -> (decimal integer string=w743:string)  [unwired: 1 in]
                                n626 = Number To Decimal String(number=w718) -> (decimal integer string=w745:string)  [unwired: 1 in]
                                n627 = Number To Decimal String(number=w732) -> (decimal integer string=w748:string)  [unwired: 1 in]
                                n628 = Number To Decimal String(number=w717) -> (decimal integer string=w750:string)  [unwired: 1 in]
                                n629 = Number To Decimal String(number=w733) -> (decimal integer string=w752:string)  [unwired: 1 in]
                                n630 = Number To Decimal String(number=w716) -> (decimal integer string=w754:string)  [unwired: 1 in]
                                n631 = local read "Data log path and filename"() -> (w715:path)
                                n632 = Get Date/Time String(want seconds? (F)=TRUE) -> (date string=w728:string, time string=w729:string)  [unwired: 2 in]
                                n633 = Number To Decimal String(number=w713) -> (decimal integer string=w712:string)  [unwired: 1 in]
                                n634 = Concatenate Strings(w712, w711, w728, "   " ("string"), w729, w711, "H1 Warning, H2 Warning", w711, w737, w711, "H1 Low Yield Warning Limit: ", w739, ", H1 yield = ", w741, w724, "H1 Low UPH Warning Limit: ", w743, ", H1 UPH = ", w745, w724, w746, w724, "H2 Low Yield Warning Limit: ", w748, ", H2 yield = ", w750, w724, "H2 Low UPH Warning Limit: ", w752, ", H2 UPH = ", w754, w724, w724) -> (w726:string)
                                n635 = call "SentinelDatalog.vi"("operation (0:open)"=T4."open", "String"=w726, "data log path"=w715) -> ()  [unwired: 8 in, 1 out]
                                }
                                frame "H1WH2A" {
                                w761 = "\r\n"
                                n636 = local read "H1 online"() -> (w782:bool)
                                n637 = local read "H2 online"() -> (w783:bool)
                                n638 = local read "H1 Yield Guage"() -> (w771:cluster{dbl, dbl})
                                n639 = local read "H2 Yield Guage"() -> (w770:cluster{dbl, dbl})
                                n640 = local read "H1 UPH warning limit"() -> (w778:dbl)
                                n641 = local read "H1 low yield warning"() -> (w777:dbl)
                                n642 = local read "H2 UPH alarm limit"() -> (w780:dbl)
                                n643 = local read "H1 UPH"() -> (w769:cluster{u32, u32})
                                n644 = local read "H2 low yield alarm"() -> (w779:dbl)
                                n645 = local read "H2 UPH"() -> (w768:cluster{u32, u32})
                                n646 = case shown="True" w782 {
                                tunnel: ["H1 Off-Line" "H1 On-Line"] -> w784
                                frame False {
                                }
                                frame True {
                                }
                                }
                                n647 = case shown="True" w783 {
                                tunnel: ["H2 Off-Line" "H2 On-Line"] -> w793
                                frame False {
                                }
                                frame True {
                                }
                                }
                                n648 = Unbundle(w771) -> (w767:dbl)  [unwired: 1 out]
                                n649 = Unbundle(w769) -> (w766:u32)  [unwired: 1 out]
                                n650 = Unbundle(w770) -> (w765:dbl)  [unwired: 1 out]
                                n651 = Unbundle(w768) -> (w764:u32)  [unwired: 1 out]
                                n652 = local read "Number of email alerts"() -> (w760:dbl)
                                n653 = Number To Decimal String(number=w777) -> (decimal integer string=w786:string)  [unwired: 1 in]
                                n654 = Number To Decimal String(number=w767) -> (decimal integer string=w788:string)  [unwired: 1 in]
                                n655 = Number To Decimal String(number=w778) -> (decimal integer string=w790:string)  [unwired: 1 in]
                                n656 = Number To Decimal String(number=w766) -> (decimal integer string=w792:string)  [unwired: 1 in]
                                n657 = Number To Decimal String(number=w779) -> (decimal integer string=w795:string)  [unwired: 1 in]
                                n658 = Number To Decimal String(number=w765) -> (decimal integer string=w797:string)  [unwired: 1 in]
                                n659 = Number To Decimal String(number=w780) -> (decimal integer string=w799:string)  [unwired: 1 in]
                                n660 = Number To Decimal String(number=w764) -> (decimal integer string=w801:string)  [unwired: 1 in]
                                n661 = local read "Data log path and filename"() -> (w763:path)
                                n662 = Get Date/Time String(want seconds? (F)=TRUE) -> (date string=w775:string, time string=w776:string)  [unwired: 2 in]
                                n663 = Number To Decimal String(number=w760) -> (decimal integer string=w759:string)  [unwired: 1 in]
                                n664 = Concatenate Strings(w759, w761, w775, "   " ("string"), w776, w761, "H1 Warning, H2 Alarming", w761, w784, w761, "H1 Low Yield Warning Limit: ", w786, ", H1 yield = ", w788, w761, "H1 Low UPH Warning Limit: ", w790, ", H1 UPH = ", w792, w761, w793, w761, "H2 Low Yield Alarm Limit: ", w795, ", H2 yield = ", w797, w761, "H2 Low UPH Alarm Limit: ", w799, ", H2 UPH = ", w801, w761, w761) -> (w773:string)
                                n665 = call "SentinelDatalog.vi"("operation (0:open)"=T4."open", "String"=w773, "data log path"=w763) -> ()  [unwired: 8 in, 1 out]
                                }
                                frame "H1AH2N" {
                                w808 = "\r\n"
                                n666 = local read "H1 online"() -> (w829:bool)
                                n667 = local read "H2 online"() -> (w830:bool)
                                n668 = local read "H1 Yield Guage"() -> (w818:cluster{dbl, dbl})
                                n669 = local read "H2 Yield Guage"() -> (w817:cluster{dbl, dbl})
                                n670 = local read "H2 UPH warning limit"() -> (w827:dbl)
                                n671 = local read "H2  low yield warning"() -> (w826:dbl)
                                n672 = local read "H1 UPH alarm limit"() -> (w825:dbl)
                                n673 = local read "H1 low yield alarm"() -> (w824:dbl)
                                n674 = local read "H1 UPH"() -> (w816:cluster{u32, u32})
                                n675 = local read "H2 UPH"() -> (w815:cluster{u32, u32})
                                n676 = case shown="True" w829 {
                                tunnel: ["H1 Off-Line" "H1 On-Line"] -> w831
                                frame False {
                                }
                                frame True {
                                }
                                }
                                n677 = case shown="False" w830 {
                                tunnel: ["H2 Off-Line" "H2 On-Line"] -> w840
                                frame False {
                                }
                                frame True {
                                }
                                }
                                n678 = Unbundle(w818) -> (w814:dbl)  [unwired: 1 out]
                                n679 = Unbundle(w816) -> (w813:u32)  [unwired: 1 out]
                                n680 = Unbundle(w817) -> (w812:dbl)  [unwired: 1 out]
                                n681 = Unbundle(w815) -> (w811:u32)  [unwired: 1 out]
                                n682 = local read "Number of email alerts"() -> (w807:dbl)
                                n683 = Number To Decimal String(number=w824) -> (decimal integer string=w833:string)  [unwired: 1 in]
                                n684 = Number To Decimal String(number=w814) -> (decimal integer string=w835:string)  [unwired: 1 in]
                                n685 = Number To Decimal String(number=w825) -> (decimal integer string=w837:string)  [unwired: 1 in]
                                n686 = Number To Decimal String(number=w813) -> (decimal integer string=w839:string)  [unwired: 1 in]
                                n687 = Number To Decimal String(number=w826) -> (decimal integer string=w842:string)  [unwired: 1 in]
                                n688 = Number To Decimal String(number=w812) -> (decimal integer string=w844:string)  [unwired: 1 in]
                                n689 = Number To Decimal String(number=w827) -> (decimal integer string=w846:string)  [unwired: 1 in]
                                n690 = Number To Decimal String(number=w811) -> (decimal integer string=w848:string)  [unwired: 1 in]
                                n691 = local read "Data log path and filename"() -> (w810:path)
                                n692 = Get Date/Time String(want seconds? (F)=TRUE) -> (date string=w822:string, time string=w823:string)  [unwired: 2 in]
                                n693 = Number To Decimal String(number=w807) -> (decimal integer string=w806:string)  [unwired: 1 in]
                                n694 = Concatenate Strings(w806, w808, w822, "   " ("string"), w823, w808, "H1 Alarming, H2 Nominal", w808, w831, w808, "H1 Low Yield Alarm Limit: ", w833, ", H1 yield = ", w835, w808, "H1 Low UPH Alarm Limit: ", w837, ", H1 UPH = ", w839, w808, w840, w808, "H2 Low Yield Warning Limit: ", w842, ", H2 yield = ", w844, w808, "H2 Low UPH Warning Limit: ", w846, ", H2 UPH = ", w848, w808, w808) -> (w820:string)
                                n695 = call "SentinelDatalog.vi"("operation (0:open)"=T4."open", "String"=w820, "data log path"=w810) -> ()  [unwired: 8 in, 1 out]
                                }
                                frame "H1AH2W" {
                                w855 = "\r\n"
                                n696 = local read "H1 online"() -> (w876:bool)
                                n697 = local read "H2 online"() -> (w877:bool)
                                n698 = local read "H1 Yield Guage"() -> (w865:cluster{dbl, dbl})
                                n699 = local read "H2 Yield Guage"() -> (w864:cluster{dbl, dbl})
                                n700 = local read "H2 UPH warning limit"() -> (w874:dbl)
                                n701 = local read "H2  low yield warning"() -> (w873:dbl)
                                n702 = local read "H1 UPH alarm limit"() -> (w872:dbl)
                                n703 = local read "H1 low yield alarm"() -> (w871:dbl)
                                n704 = local read "H1 UPH"() -> (w863:cluster{u32, u32})
                                n705 = local read "H2 UPH"() -> (w862:cluster{u32, u32})
                                n706 = case shown="True" w876 {
                                tunnel: ["H1 Off-Line" "H1 On-Line"] -> w878
                                frame False {
                                }
                                frame True {
                                }
                                }
                                n707 = case shown="True" w877 {
                                tunnel: ["H2 Off-Line" "H2 On-Line"] -> w887
                                frame False {
                                }
                                frame True {
                                }
                                }
                                n708 = Unbundle(w865) -> (w861:dbl)  [unwired: 1 out]
                                n709 = Unbundle(w863) -> (w860:u32)  [unwired: 1 out]
                                n710 = Unbundle(w864) -> (w859:dbl)  [unwired: 1 out]
                                n711 = Unbundle(w862) -> (w858:u32)  [unwired: 1 out]
                                n712 = local read "Number of email alerts"() -> (w854:dbl)
                                n713 = Number To Decimal String(number=w871) -> (decimal integer string=w880:string)  [unwired: 1 in]
                                n714 = Number To Decimal String(number=w861) -> (decimal integer string=w882:string)  [unwired: 1 in]
                                n715 = Number To Decimal String(number=w872) -> (decimal integer string=w884:string)  [unwired: 1 in]
                                n716 = Number To Decimal String(number=w860) -> (decimal integer string=w886:string)  [unwired: 1 in]
                                n717 = Number To Decimal String(number=w873) -> (decimal integer string=w889:string)  [unwired: 1 in]
                                n718 = Number To Decimal String(number=w859) -> (decimal integer string=w891:string)  [unwired: 1 in]
                                n719 = Number To Decimal String(number=w874) -> (decimal integer string=w893:string)  [unwired: 1 in]
                                n720 = Number To Decimal String(number=w858) -> (decimal integer string=w895:string)  [unwired: 1 in]
                                n721 = local read "Data log path and filename"() -> (w857:path)
                                n722 = Get Date/Time String(want seconds? (F)=TRUE) -> (date string=w869:string, time string=w870:string)  [unwired: 2 in]
                                n723 = Number To Decimal String(number=w854) -> (decimal integer string=w853:string)  [unwired: 1 in]
                                n724 = Concatenate Strings(w853, w855, w869, "   " ("string"), w870, w855, "H1 Alarming, H2 Warning", w855, w878, w855, "H1 Low Yield Alarm Limit: ", w880, ", H1 yield = ", w882, w855, "H1 Low UPH Alarm Limit: ", w884, ", H1 UPH = ", w886, w855, w887, w855, "H2 Low Yield Warning Limit: ", w889, ", H2 yield = ", w891, w855, "H2 Low UPH Warning Limit: ", w893, ", H2 UPH = ", w895, w855) -> (w867:string)
                                n725 = call "SentinelDatalog.vi"("operation (0:open)"=T4."open", "String"=w867, "data log path"=w857) -> ()  [unwired: 8 in, 1 out]
                                }
                                frame "H1AH2A" {
                                w902 = "\r\n"
                                n726 = local read "H1 online"() -> (w923:bool)
                                n727 = local read "H2 online"() -> (w924:bool)
                                n728 = local read "H1 Yield Guage"() -> (w912:cluster{dbl, dbl})
                                n729 = local read "H2 Yield Guage"() -> (w911:cluster{dbl, dbl})
                                n730 = local read "H1 UPH alarm limit"() -> (w919:dbl)
                                n731 = local read "H2 UPH alarm limit"() -> (w921:dbl)
                                n732 = local read "H1 low yield alarm"() -> (w918:dbl)
                                n733 = local read "H1 UPH"() -> (w910:cluster{u32, u32})
                                n734 = local read "H2 low yield alarm"() -> (w920:dbl)
                                n735 = local read "H2 UPH"() -> (w909:cluster{u32, u32})
                                n736 = case shown="True" w923 {
                                tunnel: ["H1 Off-Line" "H1 On-Line"] -> w925
                                frame False {
                                }
                                frame True {
                                }
                                }
                                n737 = case shown="True" w924 {
                                tunnel: ["H2 Off-Line" "H2 On-Line"] -> w934
                                frame False {
                                }
                                frame True {
                                }
                                }
                                n738 = local read "Number of email alerts"() -> (w901:dbl)
                                n739 = Unbundle(w912) -> (w908:dbl)  [unwired: 1 out]
                                n740 = Unbundle(w910) -> (w907:u32)  [unwired: 1 out]
                                n741 = Unbundle(w911) -> (w906:dbl)  [unwired: 1 out]
                                n742 = Unbundle(w909) -> (w905:u32)  [unwired: 1 out]
                                n743 = Number To Decimal String(number=w918) -> (decimal integer string=w927:string)  [unwired: 1 in]
                                n744 = Number To Decimal String(number=w908) -> (decimal integer string=w929:string)  [unwired: 1 in]
                                n745 = Number To Decimal String(number=w919) -> (decimal integer string=w931:string)  [unwired: 1 in]
                                n746 = Number To Decimal String(number=w907) -> (decimal integer string=w933:string)  [unwired: 1 in]
                                n747 = Number To Decimal String(number=w920) -> (decimal integer string=w936:string)  [unwired: 1 in]
                                n748 = Number To Decimal String(number=w906) -> (decimal integer string=w938:string)  [unwired: 1 in]
                                n749 = Number To Decimal String(number=w921) -> (decimal integer string=w940:string)  [unwired: 1 in]
                                n750 = Number To Decimal String(number=w905) -> (decimal integer string=w942:string)  [unwired: 1 in]
                                n751 = local read "Data log path and filename"() -> (w904:path)
                                n752 = Get Date/Time String(want seconds? (F)=TRUE) -> (date string=w916:string, time string=w917:string)  [unwired: 2 in]
                                n753 = Number To Decimal String(number=w901) -> (decimal integer string=w900:string)  [unwired: 1 in]
                                n754 = Concatenate Strings(w900, w902, w916, "   " ("string"), w917, w902, "H1 Alarming, H2 Alarming", w902, w925, w902, "H1 Low Yield Alarm Limit: ", w927, ", H1 yield = ", w929, w902, "H1 Low UPH Alarm Limit: ", w931, ", H1 UPH = ", w933, w902, w934, w902, "H2 Low Yield Alarm Limit: ", w936, ", H2 yield = ", w938, w902, "H2 Low UPH Alarm Limit: ", w940, ", H2 UPH = ", w942, w902, w902) -> (w914:string)
                                n755 = call "SentinelDatalog.vi"("operation (0:open)"=T4."open", "String"=w914, "data log path"=w904) -> ()  [unwired: 8 in, 1 out]
                                }
                                }
                                }
                                frame #1 {
                                n756 = Wait (ms)(milliseconds to wait=u32 100) -> ()  [unwired: 1 out]
                                }
                                frame #2 {
                                n757 = local read "Enable electronic notification of alarms"() -> (w948:bool)
                                n758 = case shown="True" w948 {
                                frame False {
                                }
                                frame True {
                                n759 = stacked-sequence {
                                frame #0 {
                                # "Email"
                                n760 = local read "Enable email notification"() -> (w951:bool)
                                n761 = local read "Number of email alerts"() -> (w950:dbl)
                                n762 = Increment(x=w950) -> (x+1=w949:dbl)
                                n763 = local write "Number of email alerts"(w949) -> ()
                                n764 = case shown="True" w951 {
                                frame False {
                                }
                                frame True {
                                n765 = flat-sequence {
                                tunnel: [w958] -> w953
                                tunnel: [w966] -> w952
                                tunnel: w953 -> [w966]
                                tunnel: w952 -> [w967]
                                frame #0 {
                                n766 = local read "Data log path and filename"() -> (w963:path)
                                n767 = local read "Number of email alerts"() -> (w957:dbl)
                                n768 = Number To Decimal String(number=w957) -> (decimal integer string=w956:string)  [unwired: 1 in]
                                n769 = Strip Path(path=w963) -> (stripped path=w961:path, name=w955:string)
                                n770 = Path To String(path=w961) -> (string=w960:string)
                                n771 = Concatenate Strings(w960, "\\sent_#" ("string"), w956, "_" ("string"), w955) -> (w964:string)
                                n772 = String To Path(string=w964) -> (path=w959:path)
                                n773 = Copy(10:w959, 11:w963) -> (3:w958:path)  [unwired: 3 in, 2 out]
                                }
                                frame #1 {
                                n774 = Wait (ms)(milliseconds to wait=u32 1000) -> ()  [unwired: 1 out]
                                }
                                frame #2 {
                                n775 = local read "Email alert - engineer"() -> (w969:string)
                                n776 = local read "Email alert - CC"() -> (w968:string)
                                n777 = local read "Email alert - message"() -> (w970:string)
                                n778 = call "email_alert.vi"("Email Alert - Message"=w970, "Email Alert - Engineer"=w969, "Email Alert - CC"=w968, "Email ALert - Attachment"=w967) -> ()  [unwired: 8 in]
                                }
                                }
                                }
                                }
                                }
                                frame #1 {
                                n779 = Wait (ms)(milliseconds to wait=u32 200) -> ()  [unwired: 1 out]
                                }
                                frame #2 {
                                # "text"
                                n780 = local read "Enable text notification"() -> (w972:bool)
                                n781 = case shown="True" w972 {
                                frame False {
                                }
                                frame True {
                                n782 = local read "Number of text alerts"() -> (w974:dbl)
                                n783 = Increment(x=w974) -> (x+1=w973:dbl)
                                n784 = local write "Number of text alerts"(w973) -> ()
                                n785 = local read "Number of email alerts"() -> (w984:dbl)
                                n786 = local read "Carrier"() -> (w976:enum16{"T-Mobile", "AT&T", "Verizon", "Sprint"})
                                n787 = local read "Phone number"() -> (w975:string)
                                n788 = local read "Lot number"() -> (w977:string)
                                n789 = Number To Decimal String(number=w984) -> (decimal integer string=w979:string)  [unwired: 1 in]
                                n790 = Concatenate Strings("Body", ", # " ("string"), w979, ", Lot Number: " ("string"), w977) -> (w985:string)
                                n791 = local write "Notifications Lot Display"(w977) -> ()
                                n792 = call <userlib>:"Send SMS 2009.vi"("Body"=w985, "Carrier"=w976, "Subject"="Subject", "phone number"=w975, "smtp server"="smtp.gmail.com", "password"="sentinelcontroller", "email username"="sentinelcontroller@gmail.com") -> ("Error Out"=w983:errorcluster)  [unwired: 4 in]
                                n793 = Unbundle By Name(w983) -> ("status"=w982:bool)
                                n794 = case shown="True" w982 {
                                frame False {
                                }
                                frame True {
                                n795 = One Button Dialog(message="Error sending text message!\nTry changing the setting or\nswitch to email method", button name ("OK")="Dismiss") -> ()  [unwired: 1 out]
                                }
                                }
                                }
                                }
                                }
                                }
                                }
                                }
                                }
                                frame #3 {
                                n796 = Wait (ms)(milliseconds to wait=u32 100) -> ()  [unwired: 1 out]
                                }
                                }
                                }
                              }
                            }
                          }
                        }
                      }
                    }
                  }
                  n797 = Wait (ms)(milliseconds to wait=u32 100) -> ()  [unwired: 1 out]
                }
                n798 = local read "Yield averaging"() -> (w273:u32)
                n799 = local read "UPH averaging"() -> (w274:u32)
                n800 = Initialize Array(w280, w273) -> (w279:dbl[])
                n801 = Initialize Array(w283, w274) -> (w285:dbl[])
                n802 = while {
                  shift-right: [w1430] -> _
                  shift-left: w284 -> [w1428]
                  shift-right: [w1429] -> _
                  shift-left: w286 -> [w1427]
                  shift-right: [w1422] -> _
                  shift-left: w282 -> [w1425]
                  shift-right: [w1423] -> _
                  shift-left: w281 -> [w1424]
                  shift-right: [w1421] -> _
                  shift-left: TRUE -> [w1418]
                  tunnel: w276 -> [w1420]
                  tunnel: w275 -> [w1419]
                  i -> [w1426]
                  stop <- w1434 stop-if-true
                  # "H1 loop"
                  n803 = Wait (ms)(milliseconds to wait=u32 10) -> ()  [unwired: 1 out]
                  n804 = flat-sequence {
                    tunnel: w1426 -> [w1437]
                    tunnel: w1418 -> [w1459]
                    tunnel: [w1489] -> w1430
                    tunnel: [w1488] -> w1429
                    tunnel: w1428 -> [w1487]
                    tunnel: w1427 -> [w1486]
                    tunnel: w1426 -> [w1485]
                    tunnel: w1426 -> [w1484]
                    tunnel: w1425 -> [w1483]
                    tunnel: w1424 -> [w1482]
                    tunnel: [w1481] -> w1423
                    tunnel: [w1480] -> w1422
                    tunnel: w1418 -> [_]
                    tunnel: [w1476] -> w1421
                    tunnel: w1420 -> [w1479]
                    tunnel: w1419 -> [w1478]
                    frame #0 {
                      n805 = Equal To 0?(x=w1437) -> (x = 0?=w1438:bool)
                      n806 = case shown="True" w1438 {
                        frame False {
                        }
                        frame True {
                          w1449 = FALSE ("H1 Testing")
                          # "On first pass, H1 wait is shorter than\nH2 (200ms). It will always start first."
                          # "H1 first pass init"
                          n807 = local read "H1 low UPH alarm (%)"() -> (w1442:dbl)
                          n808 = local write "H1 Wait Time"(0.0 ("H1 Wait Time")) -> ()
                          n809 = local write "H1 Index Time"(0.0 ("H1 Index Time")) -> ()
                          n810 = local write "H1 Test Time"(0.0 ("H1 Test Time")) -> ()
                          n811 = local write "H1 Device Count"(0.0 ("H1 Device Count")) -> ()
                          n812 = local read "H1 low yield alarm"() -> (w1457:dbl)
                          n813 = Divide(x=w1442, y=100.0) -> (x/y=w1440:dbl)
                          n814 = Bundle(100.0, "H1 low yield alarm"=w1457) -> (w1456:cluster{dbl, "H1 low yield alarm":dbl})  [unwired: 1 in]
                          n815 = local write "H1 Yield Guage"(w1456) -> ()
                          n816 = property on="H1 UPH" class="Knob (strict)"() -> ("Scale.Maximum"=w1443:dbl)  [unwired: 2 in, 2 out]
                          n817 = Multiply(x=w1443, y=w1440) -> (x*y=w1439:dbl)
                          n818 = Bundle("Scale.Maximum"=w1443, w1439) -> (w1458:cluster{"Scale.Maximum":dbl, dbl})  [unwired: 1 in]
                          n819 = Wait (ms)(milliseconds to wait=u32 50) -> ()  [unwired: 1 out]
                          n820 = local write "H1 UPH"(w1458) -> ()
                          "H1 Pass" <- TRUE ("H1 Result")
                          "H1 Testing" <- w1449
                          "H1 Waiting" <- w1449
                          "H1 Indexing" <- w1449
                          "H1 Device Count" <- u32 0
                          "H1 Good Units" <- u32 0
                          "H1 results" <- u32 0 ("H1 Results")
                          "H1 Yield Mon" <- 100.0 ("H1 Yield Mon")
                        }
                      }
                    }
                    frame #1 {
                      n821 = local read "H1 online"() -> (w1460:bool)
                      n822 = Not Equal?(x=w1460, y=w1459) -> (x != y?=w1461:bool)
                      n823 = case shown="True" w1461 {
                        frame False {
                        }
                        frame True {
                          n824 = local read "Enable data logging of all events"() -> (w1462:bool)
                          n825 = case shown="True" w1462 {
                            frame False {
                            }
                            frame True {
                              w1465 = "\r\n"
                              n826 = local read "H1 online"() -> (w1467:bool)
                              n827 = case shown="False" w1467 {
                                tunnel: ["H1 Off-Line" "H1 On-Line"] -> w1466
                                frame False {
                                }
                                frame True {
                                }
                              }
                              n828 = local read "Data log path and filename"() -> (w1464:path)
                              n829 = Get Date/Time String(want seconds? (F)=TRUE) -> (date string=w1470:string, time string=w1469:string)  [unwired: 2 in]
                              n830 = Concatenate Strings(w1470, "   " ("string"), w1469, w1465, "Change in H1 Status: ", w1466, w1465, w1465) -> (w1472:string)
                              n831 = call "SentinelDatalog.vi"("operation (0:open)"=T4."open", "String"=w1472, "data log path"=w1464) -> ()  [unwired: 8 in, 1 out]
                            }
                          }
                        }
                      }
                    }
                    frame #2 {
                      n832 = local read "H1 online"() -> (w1477:bool)
                      n833 = case shown="False" w1477 {
                        frame False {
                          n834 = while {
                            stop <- w1494 stop-if-true
                            w1491 = 0.0
                            n835 = local write "Sim H1 UPH"(u32 0 ("Sim H1 UPH")) -> ()
                            n836 = Wait (ms)(milliseconds to wait=u32 100) -> ()  [unwired: 1 out]
                            n837 = local read "H1 online"() -> (w1494:bool)
                            n838 = Bundle(w1491, w1491) -> (w1490:cluster{dbl, dbl})  [unwired: 1 in]
                            n839 = local write "H1 Yield Guage"(w1490) -> ()
                            n840 = local write "H1 UPH"(w1490) -> ()
                          }
                        }
                        frame True {
                        }
                      }
                      n841 = local read "H1 online"() -> (w1476:bool)
                      n842 = case shown="True" w1476 {
                        tunnel: [w1497 w1522] -> w1489
                        tunnel: [w1499 w1521] -> w1488
                        tunnel: w1487 -> [w1498 w1520]
                        tunnel: w1486 -> [w1500 w1519]
                        tunnel: w1485 -> [w1496 w1518]
                        tunnel: w1484 -> [w1505 w1517]
                        tunnel: w1483 -> [w1507 w1516]
                        tunnel: w1482 -> [w1508 w1515]
                        tunnel: [w1509 w1514] -> w1481
                        tunnel: [w1506 w1513] -> w1480
                        tunnel: w1479 -> [_ w1512]
                        tunnel: w1478 -> [w1495 w1511]
                        frame False {
                          n843 = local write "H1 Waiting"(FALSE ("H1 Ready")) -> ()
                          n844 = local read "H1 Yield Guage"() -> (w1504:cluster{dbl, dbl})
                          n845 = Unbundle(w1504) -> (w1503:dbl)  [unwired: 1 out]
                          n846 = call "moving_avg_core.vi"("Array in"=w1508, "avg"=w1495, "accumulator in"=w1507, "i"=w1505, "data in"=w1503) -> ("Array out"=w1509:dbl[], "accumulator out"=w1506:dbl)  [unwired: 4 in, 1 out]
                          n847 = local read "H1 UPH"() -> (w1501:cluster{u32, u32})
                          n848 = Unbundle(w1501) -> (w1502:u32)  [unwired: 1 out]
                          n849 = call "moving_avg_core.vi"("Array in"=w1500, "accumulator in"=w1498, "i"=w1496, "data in"=w1502) -> ("Array out"=w1499:dbl[], "accumulator out"=w1497:dbl)  [unwired: 5 in, 1 out]
                        }
                        frame True {
                          w1539 = FALSE ("H1 Testing")
                          # "H1 is now unlocked by tester\nand free to continue with binning\nMeanwhile, H2 can begin testing while H\nis binning."
                          # "H1 SOT sent to tester"
                          n850 = local write "H1 Indexing"(w1539) -> ()
                          n851 = local write "H1 Waiting"(TRUE ("H1 Ready")) -> ()
                          n852 = local write "H1 Testing"(w1539) -> ()
                          n853 = flat-sequence {
                            tunnel: [w1625] -> w1538
                            tunnel: w1538 -> [w1626]
                            tunnel: [w1626] -> w1537
                            tunnel: w1537 -> [w1637]
                            tunnel: [w1637] -> w1536
                            tunnel: [w1636] -> w1535
                            tunnel: w1536 -> [w1639]
                            tunnel: [w1639] -> w1528
                            tunnel: [w1638] -> w1527
                            tunnel: w1535 -> [w1638]
                            tunnel: w1528 -> [w1652]
                            tunnel: [w1652] -> w1526
                            tunnel: w1527 -> [w1651]
                            tunnel: [w1651] -> w1524
                            tunnel: w1526 -> [w1657]
                            tunnel: [w1657] -> w1525
                            tunnel: w1524 -> [w1656]
                            tunnel: [w1656] -> w1523
                            tunnel: w1525 -> [w1685]
                            tunnel: [w1685] -> w1534
                            tunnel: [w1684] -> w1533
                            tunnel: w1523 -> [w1684]
                            tunnel: w1517 -> [w1671]
                            tunnel: w1516 -> [w1670]
                            tunnel: w1515 -> [w1669]
                            tunnel: [w1668] -> w1514
                            tunnel: [w1667] -> w1513
                            tunnel: w1511 -> [w1658]
                            tunnel: w1534 -> [w1703]
                            tunnel: w1533 -> [w1702]
                            tunnel: [w1703] -> w1542
                            tunnel: [w1702] -> w1541
                            tunnel: [w1701] -> w1540
                            frame #0 {
                              # "start of\nwait time"
                              n854 = Tick Count (ms)() -> (millisecond timer value=w1625:u32)
                            }
                            frame #1 {
                              # "H1 waiting"
                              n855 = while {
                                stop <- w1630 stop-if-true
                                # "SOT issued - thinks it is testing, but\nmay not be depending upon H2\nbeing in control of the tester."
                                n856 = local read "POWER"() -> (w1629:bool)
                                n857 = local read "Run / Stop"() -> (w1628:bool)
                                n858 = Wait (ms)(milliseconds to wait=u32 1) -> ()  [unwired: 1 out]
                                n859 = local read "H1 Lock"() -> (w1627:bool)
                                n860 = Not(x=w1629) -> (.not. x?=w1632:bool)
                                n861 = Not(x=w1628) -> (.not. x?=w1631:bool)
                                n862 = Compound Arithmetic op=OR(w1627, w1632, w1631) -> (w1630:bool)
                              }
                            }
                            frame #2 {
                              # "start of \ntest time"
                              n863 = local write "H1 Waiting"(FALSE ("H1 Ready")) -> ()
                              n864 = local write "H1 Testing"(TRUE ("H1 Testing")) -> ()
                              n865 = Tick Count (ms)() -> (millisecond timer value=w1636:u32)
                            }
                            frame #3 {
                              # "H1 testing"
                              n866 = while {
                                stop <- w1643 stop-if-true
                                # "H1 testing because tester sent EOT\nto H2 and this program knows it."
                                n867 = local read "POWER"() -> (w1641:bool)
                                n868 = local read "Run / Stop"() -> (w1640:bool)
                                n869 = Wait (ms)(milliseconds to wait=u32 10) -> ()  [unwired: 1 out]
                                n870 = local read "H1 Testing"() -> (w1647:bool)
                                n871 = Not(x=w1647) -> (.not. x?=w1642:bool)
                                n872 = Not(x=w1641) -> (.not. x?=w1645:bool)
                                n873 = Not(x=w1640) -> (.not. x?=w1644:bool)
                                n874 = Compound Arithmetic op=OR(w1642, w1645, w1644) -> (w1643:bool)
                              }
                            }
                            frame #4 {
                              n875 = local read "H1 Device Count"() -> (w1648:u32)
                              n876 = local read "Parallelism"() -> (w1650:u32)
                              n877 = Add(x=w1650, y=w1648) -> (x+y=w1649:u32)
                              n878 = local write "H1 Device Count"(w1649) -> ()
                            }
                            frame #5 {
                              n879 = local read "H1 results"() -> (w1655:u32)
                              n880 = local read "H1 Good Units"() -> (w1653:u32)
                              n881 = Add(x=w1655, y=w1653) -> (x+y=w1654:u32)
                              n882 = local write "H1 Good Units"(w1654) -> ()
                            }
                            frame #6 {
                              # "H1 binning and low yield alarms"
                              n883 = local read "H1 Device Count"() -> (w1680:u32)
                              n884 = local read "H1 parallelism"() -> (w1664:u8)
                              n885 = local read "H1 Good Units"() -> (w1679:u32)
                              n886 = local read "H1 results"() -> (w1665:u32)
                              n887 = Divide(x=w1679, y=w1680) -> (x/y=w1682:dbl)
                              n888 = Divide(x=w1665, y=w1664) -> (x/y=w1662:dbl)
                              n889 = Multiply(x=100, y=w1682) -> (x*y=w1666:dbl)
                              n890 = local write "H1 Yield Mon"(w1666) -> ()
                              n891 = local read "H1 low yield alarm"() -> (w1676:dbl)
                              n892 = Multiply(x=100, y=w1662) -> (x*y=w1661:dbl)
                              n893 = local read "H2 Yield Guage"() -> (w1660:cluster{dbl, dbl})
                              n894 = local read "H1 low yield alarm"() -> (w1675:dbl)
                              n895 = local read "H2 low yield alarm"() -> (w1674:dbl)
                              n896 = local read "H1 low yield warning"() -> (w1678:dbl)
                              n897 = Unbundle(w1660) -> (w1659:dbl)  [unwired: 1 out]
                              n898 = call "moving_avg_core.vi"("Array in"=w1669, "avg"=w1658, "accumulator in"=w1670, "i"=w1671, "data in"=w1661) -> ("Array out"=w1668:dbl[], "accumulator out"=w1667:dbl, "rolling avg out"=w1672:dbl)  [unwired: 4 in]
                              n899 = Less?(x=w1672, y=w1678) -> (x < y?=w1677:bool)
                              n900 = Bundle("rolling avg out"=w1672, w1659, "H1 low yield alarm"=w1675, "H2 low yield alarm"=w1674) -> (w1673:T6)  [unwired: 1 in]
                              n901 = case shown="True" w1677 {
                                tunnel: w1672 -> [_ w1691]
                                tunnel: w1676 -> [_ w1690]
                                frame False {
                                n902 = local write "H1 warning"(FALSE ("H1 warning")) -> ()
                                n903 = local write "H1 nominal"(TRUE ("H1 nominal")) -> ()
                                n904 = local write "H1 alarm"(FALSE ("H1 warning")) -> ()
                                }
                                frame True {
                                n905 = Less?(x=w1691, y=w1690) -> (x < y?=w1689:bool)
                                n906 = case shown="True" w1689 {
                                frame False {
                                n907 = local write "H1 warning"(TRUE ("H1 warning")) -> ()
                                n908 = local write "H1 nominal"(FALSE ("H1 nominal")) -> ()
                                n909 = local write "H1 alarm"(FALSE ("H1 warning")) -> ()
                                }
                                frame True {
                                n910 = local read "H1 enable halt\non yield alarm"() -> (w1695:bool)
                                n911 = case shown="True" w1695 {
                                frame False {
                                }
                                frame True {
                                n912 = local write "H1 online"(FALSE ("H1 Online")) -> ()
                                }
                                }
                                n913 = local write "H1 warning"(FALSE ("H1 warning")) -> ()
                                n914 = local write "H1 nominal"(FALSE ("H1 nominal")) -> ()
                                n915 = local write "H1 alarm"(TRUE ("H1 warning")) -> ()
                                }
                                }
                                }
                              }
                              n916 = Bundle("rolling avg out"=w1672, "H1 low yield alarm"=w1676) -> (→"H1 Yield Guage":T7)  [unwired: 1 in]
                              n917 = local write "YieldMon"(w1673) -> ()
                            }
                            frame #7 {
                              # "start of\nindex time"
                              n918 = local write "H1 Indexing"(TRUE ("H1 Indexing")) -> ()
                              n919 = local write "H1 Lock"(FALSE ("H1 Lock")) -> ()
                              n920 = Tick Count (ms)() -> (millisecond timer value=w1701:u32)
                            }
                          }
                          n921 = flat-sequence {
                            tunnel: [w1548] -> w1532
                            tunnel: [w1547] -> w1531
                            tunnel: w1542 -> [w1547]
                            tunnel: [w1546] -> w1530
                            tunnel: w1541 -> [w1546]
                            tunnel: [w1545] -> w1529
                            tunnel: w1540 -> [w1545]
                            tunnel: w1518 -> [w1559]
                            tunnel: w1519 -> [w1563]
                            tunnel: w1520 -> [w1564]
                            tunnel: [w1566] -> w1521
                            tunnel: [w1567] -> w1522
                            tunnel: w1532 -> [w1586]
                            tunnel: w1531 -> [w1585]
                            tunnel: w1530 -> [w1584]
                            tunnel: w1529 -> [w1583]
                            tunnel: w1512 -> [w1560]
                            frame #0 {
                              # "H1 indexing"
                              n922 = local read "H1 index time\nvariation (%)"() -> (w1557:i32)
                              n923 = local read "H1 index\ntime set"() -> (w1556:dbl)
                              n924 = Divide(x=w1557, y=100.0) -> (x/y=w1550:dbl)
                              n925 = Multiply(x=w1550, y=w1556) -> (x*y=w1553:dbl)
                              n926 = Random Number (0-1)() -> (number: 0 to 1=w1552:dbl)
                              n927 = local read "Time Accerlation  Factor"() -> (w1544:dbl)
                              n928 = Multiply(x=w1553, y=w1552) -> (x*y=w1549:dbl)
                              n929 = Add(x=w1549, y=w1556) -> (x+y=w1555:dbl)
                              n930 = Multiply(x=w1555, y=1000.0) -> (x*y=w1558:dbl)
                              n931 = Divide(x=w1558, y=w1544) -> (x/y=w1548:dbl)
                              n932 = Wait (ms)(milliseconds to wait=w1548) -> ()  [unwired: 1 out]
                            }
                            frame #1 {
                              # "calculate test, tindex, and wait times, UPH"
                              # "end of test time"
                              # "start of test time"
                              # "start of wait time"
                              # "Check H1 UPH against warning and alert limits"
                              n933 = local read "Time Accerlation  Factor"() -> (w1570:dbl)
                              n934 = local write "H1 Indexing"(FALSE ("H1 Indexing")) -> ()
                              n935 = Equal To 0?(x=w1559) -> (x = 0?=w1561:bool)
                              n936 = local read "Parallelism"() -> (w1595:u32)
                              n937 = local read "Parallelism"() -> (w1596:u32)
                              n938 = case shown="True" w1561 {
                                tunnel: w1585 -> [w1607 _]
                                tunnel: w1584 -> [w1606 _]
                                tunnel: [w1605 0] -> w1571
                                frame False {
                                n939 = Subtract(x=w1606, y=w1607) -> (x-y=w1609:u32)
                                n940 = Divide(x=w1609, y=1000.0) -> (x/y=w1605:dbl)
                                }
                                frame True {
                                }
                              }
                              n941 = Subtract(x=w1583, y=w1584) -> (x-y=w1602:u32)
                              n942 = Divide(x=w1602, y=1000.0) -> (x/y=w1572:dbl)
                              n943 = Divide(x=w1586, y=1000.0) -> (x/y=w1573:dbl)
                              n944 = Multiply(x=w1595, y=u32 3600 ("x")) -> (x*y=w1593:u32)
                              n945 = Multiply(x=w1596, y=u32 3600 ("x")) -> (x*y=w1598:u32)
                              n946 = Compound Arithmetic op=ADD(w1573, w1572, w1571) -> (w1600:dbl)
                              n947 = Compound Arithmetic op=ADD(w1573, w1572) -> (w1592:dbl)
                              n948 = Divide(x=w1593, y=w1592) -> (x/y=w1591:dbl)
                              n949 = Multiply(x=w1570, y=w1572) -> (x*y=→"H1 Test Time" →"H1 TT (s/cycle)":dbl)
                              n950 = Divide(x=w1598, y=w1600) -> (x/y=w1599:dbl)
                              n951 = Multiply(x=w1570, y=w1573) -> (x*y=→"H1 Index Time" →"H1 IT (s/cycle)":dbl)
                              n952 = Multiply(x=w1570, y=w1571) -> (x*y=→"H1 Wait Time" →"H1 WT (s/cycle)":dbl)
                              n953 = Divide(x=w1591, y=w1570) -> (x/y=→"H1 Single Handler UPH":dbl)
                              n954 = Divide(x=w1599, y=w1570) -> (x/y=w1568:dbl)
                              n955 = call "moving_avg_core.vi"("Array in"=w1563, "avg"=w1560, "accumulator in"=w1564, "i"=w1559, "data in"=w1568) -> ("Array out"=w1566:dbl[], "accumulator out"=w1567:dbl, "rolling avg out"=w1565:dbl)  [unwired: 4 in]
                              n956 = local read "H1 low UPH warning (%)"() -> (w1582:dbl)
                              n957 = local read "H1 low UPH alarm (%)"() -> (w1576:dbl)
                              n958 = property on="H1 UPH" class="Knob (strict)"() -> ("Scale.Maximum"=w1574:dbl)  [unwired: 2 in, 2 out]
                              n959 = Divide(x=w1576, y=100.0) -> (x/y=w1578:dbl)
                              n960 = Divide(x=w1582, y=100.0) -> (x/y=w1580:dbl)
                              n961 = Multiply(x=w1574, y=w1578) -> (x*y=w1562:dbl)
                              "H1 UPH alarm limit" <- w1562
                              n962 = Multiply(x=w1574, y=w1580) -> (x*y=w1581:dbl)
                              "H1 UPH warning limit" <- w1581
                              n963 = Less?(x=w1565, y=w1581) -> (x < y?=w1575:bool)
                              n964 = case shown="True" w1575 {
                                tunnel: w1565 -> [_ w1615]
                                tunnel: w1562 -> [_ w1614]
                                frame False {
                                n965 = local write "H1 warning 2"(FALSE ("H1 warning")) -> ()
                                n966 = local write "H1 nominal 2"(TRUE ("H1 nominal")) -> ()
                                n967 = local write "H1 alarm 2"(FALSE ("H1 warning")) -> ()
                                }
                                frame True {
                                n968 = Less?(x=w1615, y=w1614) -> (x < y?=w1616:bool)
                                n969 = case shown="True" w1616 {
                                frame False {
                                n970 = local write "H1 warning 2"(TRUE ("H1 warning")) -> ()
                                n971 = local write "H1 nominal 2"(FALSE ("H1 nominal")) -> ()
                                n972 = local write "H1 alarm 2"(FALSE ("H1 warning")) -> ()
                                }
                                frame True {
                                n973 = local read "H1 enable halt\non UPH alarm"() -> (w1620:bool)
                                n974 = local write "H1 warning 2"(FALSE ("H1 warning")) -> ()
                                n975 = local write "H1 nominal 2"(FALSE ("H1 nominal")) -> ()
                                n976 = local write "H1 alarm 2"(TRUE ("H1 warning")) -> ()
                                n977 = case shown="True" w1620 {
                                frame False {
                                }
                                frame True {
                                n978 = local write "H1 online"(FALSE ("H1 Online")) -> ()
                                }
                                }
                                }
                                }
                                }
                              }
                              n979 = Bundle("rolling avg out"=w1565, w1562) -> (→"H1 UPH":cluster{"rolling avg out":dbl, dbl})  [unwired: 1 in]
                            }
                          }
                        }
                      }
                    }
                  }
                  n980 = local read "Run / Stop"() -> (w1431:bool)
                  n981 = local read "POWER"() -> (w1433:bool)
                  n982 = Not(x=w1431) -> (.not. x?=w1436:bool)
                  n983 = Not(x=w1433) -> (.not. x?=w1435:bool)
                  n984 = Compound Arithmetic op=OR(w1436, w1435) -> (w1434:bool)
                }
                n985 = while {
                  shift-right: [w1143] -> _
                  shift-left: w283 -> [w1141]
                  shift-right: [w1142] -> _
                  shift-left: w285 -> [w1140]
                  shift-right: [w1135] -> _
                  shift-left: w280 -> [w1138]
                  shift-right: [w1136] -> _
                  shift-left: w279 -> [w1137]
                  shift-right: [w1134] -> _
                  shift-left: TRUE -> [w1131]
                  tunnel: w273 -> [w1133]
                  tunnel: w274 -> [w1132]
                  i -> [w1139]
                  stop <- w1147 stop-if-true
                  # "H2 loop"
                  n986 = flat-sequence {
                    tunnel: w1139 -> [w1150]
                    tunnel: w1131 -> [w1172]
                    tunnel: [w1202] -> w1143
                    tunnel: [w1201] -> w1142
                    tunnel: w1141 -> [w1200]
                    tunnel: w1140 -> [w1199]
                    tunnel: w1139 -> [w1198]
                    tunnel: w1139 -> [w1197]
                    tunnel: w1138 -> [w1196]
                    tunnel: w1137 -> [w1195]
                    tunnel: [w1194] -> w1136
                    tunnel: [w1193] -> w1135
                    tunnel: [w1189] -> w1134
                    tunnel: w1133 -> [w1192]
                    tunnel: w1132 -> [w1191]
                    frame #0 {
                      n987 = Equal To 0?(x=w1150) -> (x = 0?=w1151:bool)
                      n988 = case shown="True" w1151 {
                        frame False {
                        }
                        frame True {
                          w1163 = FALSE ("H2 Testing")
                          # "H2 first pass init"
                          n989 = local read "H2 low UPH alarm (%)"() -> (w1155:dbl)
                          n990 = local read "H2 low yield alarm"() -> (w1170:dbl)
                          n991 = local write "H2 Test Time"(0.0 ("H2 Test Time")) -> ()
                          n992 = local write "H2 Device Count"(0.0 ("H2 Device Count")) -> ()
                          n993 = local write "H2 Wait Time"(0.0 ("H2 Wait Time")) -> ()
                          n994 = local write "H2 Index Time"(0.0 ("H2 Index Time")) -> ()
                          n995 = property on="H2 UPH" class="Knob (strict)"() -> ("Scale.Maximum"=w1154:dbl)  [unwired: 2 in, 2 out]
                          n996 = Divide(x=w1155, y=100.0) -> (x/y=w1157:dbl)
                          n997 = Multiply(x=w1154, y=w1157) -> (x*y=w1153:dbl)
                          n998 = Bundle("Scale.Maximum"=w1154, w1153) -> (w1152:cluster{"Scale.Maximum":dbl, dbl})  [unwired: 1 in]
                          n999 = Bundle(100.0, "H2 low yield alarm"=w1170) -> (w1169:cluster{dbl, "H2 low yield alarm":dbl})  [unwired: 1 in]
                          n1000 = local write "H2 UPH"(w1152) -> ()
                          n1001 = local write "H2 Yield Guage"(w1169) -> ()
                          n1002 = Wait (ms)(milliseconds to wait=u32 200) -> ()  [unwired: 1 out]
                          "H2 Pass" <- TRUE ("H2 Result")
                          "H2 Testing" <- w1163
                          "H2 Waiting" <- w1163
                          "H2 Indexing" <- w1163
                          "H2 Good Units" <- 0
                          "H2 Device Count" <- 0
                          "H2 results" <- u32 0 ("H2 Results")
                          "H2 Yield  Mon" <- 100.0 ("H2 Yield  Mon")
                        }
                      }
                    }
                    frame #1 {
                      n1003 = local read "H2 online"() -> (w1174:bool)
                      n1004 = Not Equal?(x=w1174, y=w1172) -> (x != y?=w1173:bool)
                      n1005 = case shown="True" w1173 {
                        frame False {
                        }
                        frame True {
                          n1006 = local read "Enable data logging of all events"() -> (w1175:bool)
                          n1007 = case shown="True" w1175 {
                            frame False {
                            }
                            frame True {
                              w1178 = "\r\n"
                              n1008 = local read "H2 online"() -> (w1180:bool)
                              n1009 = local read "Data log path and filename"() -> (w1177:path)
                              n1010 = case shown="False" w1180 {
                                tunnel: ["H2 Off-Line" "H2 On-Line"] -> w1179
                                frame False {
                                }
                                frame True {
                                }
                              }
                              n1011 = Get Date/Time String(want seconds? (F)=TRUE) -> (date string=w1183:string, time string=w1182:string)  [unwired: 2 in]
                              n1012 = Concatenate Strings(w1183, "   " ("string"), w1182, w1178, "Change in H2 Status: ", w1179, w1178, w1178) -> (w1185:string)
                              n1013 = call "SentinelDatalog.vi"("operation (0:open)"=T4."open", "String"=w1185, "data log path"=w1177) -> ()  [unwired: 8 in, 1 out]
                            }
                          }
                        }
                      }
                    }
                    frame #2 {
                      n1014 = local read "H2 online"() -> (w1190:bool)
                      n1015 = case shown="False" w1190 {
                        frame False {
                          n1016 = while {
                            stop <- w1207 stop-if-true
                            w1204 = 0.0
                            n1017 = local read "H2 online"() -> (w1207:bool)
                            n1018 = Wait (ms)(milliseconds to wait=u32 100) -> ()  [unwired: 1 out]
                            n1019 = local write "Sim H2 UPH"(u32 0 ("Sim H2 UPH")) -> ()
                            n1020 = Bundle(w1204, w1204) -> (w1203:cluster{dbl, dbl})  [unwired: 1 in]
                            n1021 = local write "H2 Yield Guage"(w1203) -> ()
                            n1022 = local write "H2 UPH"(w1203) -> ()
                          }
                        }
                        frame True {
                        }
                      }
                      n1023 = local read "H2 online"() -> (w1189:bool)
                      n1024 = case shown="False" w1189 {
                        tunnel: [w1213 w1235] -> w1202
                        tunnel: [w1214 w1234] -> w1201
                        tunnel: w1200 -> [w1212 w1233]
                        tunnel: w1199 -> [w1215 w1232]
                        tunnel: w1198 -> [w1211 w1231]
                        tunnel: w1197 -> [w1217 w1230]
                        tunnel: w1196 -> [w1218 w1229]
                        tunnel: w1195 -> [w1221 w1228]
                        tunnel: [w1220 w1227] -> w1194
                        tunnel: [w1219 w1226] -> w1193
                        tunnel: w1192 -> [w1208 w1225]
                        tunnel: w1191 -> [_ w1224]
                        frame False {
                          n1025 = local write "H2 Waiting"(FALSE ("H2 Ready")) -> ()
                          n1026 = local read "H2 Yield Guage"() -> (w1222:cluster{dbl, dbl})
                          n1027 = Unbundle(w1222) -> (w1216:dbl)  [unwired: 1 out]
                          n1028 = call "moving_avg_core.vi"("Array in"=w1221, "avg"=w1208, "accumulator in"=w1218, "i"=w1217, "data in"=w1216) -> ("Array out"=w1220:dbl[], "accumulator out"=w1219:dbl)  [unwired: 4 in, 1 out]
                          n1029 = local read "H2 UPH"() -> (w1210:cluster{u32, u32})
                          n1030 = Unbundle(w1210) -> (w1209:u32)  [unwired: 1 out]
                          n1031 = call "moving_avg_core.vi"("Array in"=w1215, "accumulator in"=w1212, "i"=w1211, "data in"=w1209) -> ("Array out"=w1214:dbl[], "accumulator out"=w1213:dbl)  [unwired: 5 in, 1 out]
                        }
                        frame True {
                          w1252 = FALSE ("H2 Testing")
                          # "H2 is now unlocked by tester\nand free to continue with binning\nMeanwhile, H1 can begin testing while H2\nis binning."
                          # "H2 SOT sent to tester"
                          n1032 = local write "H2 Indexing"(w1252) -> ()
                          n1033 = local write "H2 Testing"(w1252) -> ()
                          n1034 = local write "H2 Waiting"(TRUE ("H2 Ready")) -> ()
                          n1035 = flat-sequence {
                            tunnel: [w1257] -> w1247
                            tunnel: [w1258] -> w1246
                            tunnel: w1247 -> [w1258]
                            tunnel: w1246 -> [w1269]
                            tunnel: [w1269] -> w1245
                            tunnel: [w1268] -> w1244
                            tunnel: [w1271] -> w1241
                            tunnel: [w1270] -> w1240
                            tunnel: w1245 -> [w1271]
                            tunnel: w1244 -> [w1270]
                            tunnel: w1241 -> [w1284]
                            tunnel: [w1284] -> w1239
                            tunnel: w1240 -> [w1283]
                            tunnel: [w1283] -> w1237
                            tunnel: w1239 -> [w1289]
                            tunnel: [w1289] -> w1238
                            tunnel: w1237 -> [w1288]
                            tunnel: [w1288] -> w1236
                            tunnel: w1238 -> [w1317]
                            tunnel: w1236 -> [w1316]
                            tunnel: [w1316] -> w1243
                            tunnel: [w1317] -> w1242
                            tunnel: w1230 -> [w1304]
                            tunnel: w1229 -> [w1303]
                            tunnel: w1228 -> [w1302]
                            tunnel: [w1301] -> w1227
                            tunnel: [w1300] -> w1226
                            tunnel: w1225 -> [w1290]
                            tunnel: [w1335] -> w1253
                            tunnel: [w1336] -> w1255
                            tunnel: w1243 -> [w1336]
                            tunnel: w1242 -> [w1335]
                            tunnel: [w1334] -> w1254
                            frame #0 {
                              # "start of\nwait time"
                              n1036 = Tick Count (ms)() -> (millisecond timer value=w1257:u32)
                            }
                            frame #1 {
                              # "H2 waiting"
                              n1037 = while {
                                stop <- w1262 stop-if-true
                                # "SOT issued - thinks it is testing, but\nmay not be depending upon H1\nbeing in control of the tester."
                                n1038 = local read "POWER"() -> (w1261:bool)
                                n1039 = local read "Run / Stop"() -> (w1259:bool)
                                n1040 = Wait (ms)(milliseconds to wait=u32 1) -> ()  [unwired: 1 out]
                                n1041 = local read "H2 Lock"() -> (w1260:bool)
                                n1042 = Not(x=w1261) -> (.not. x?=w1264:bool)
                                n1043 = Not(x=w1259) -> (.not. x?=w1263:bool)
                                n1044 = Compound Arithmetic op=OR(w1260, w1264, w1263) -> (w1262:bool)
                              }
                            }
                            frame #2 {
                              # "start of\ntest time"
                              n1045 = Tick Count (ms)() -> (millisecond timer value=w1268:u32)
                              n1046 = local write "H2 Waiting"(FALSE ("H2 Ready")) -> ()
                              n1047 = local write "H2 Testing"(TRUE ("H2 Testing")) -> ()
                            }
                            frame #3 {
                              # "H2 testing"
                              n1048 = while {
                                stop <- w1275 stop-if-true
                                # "H2 testing because tester sent EOT\nto H1 and this program knows it."
                                n1049 = local read "POWER"() -> (w1274:bool)
                                n1050 = local read "H2 Testing"() -> (w1279:bool)
                                n1051 = local read "Run / Stop"() -> (w1272:bool)
                                n1052 = Wait (ms)(milliseconds to wait=u32 10) -> ()  [unwired: 1 out]
                                n1053 = Not(x=w1279) -> (.not. x?=w1273:bool)
                                n1054 = Not(x=w1274) -> (.not. x?=w1277:bool)
                                n1055 = Not(x=w1272) -> (.not. x?=w1276:bool)
                                n1056 = Compound Arithmetic op=OR(w1273, w1277, w1276) -> (w1275:bool)
                              }
                            }
                            frame #4 {
                              n1057 = local read "H2 Device Count"() -> (w1282:u32)
                              n1058 = local read "Parallelism"() -> (w1280:u32)
                              n1059 = Add(x=w1280, y=w1282) -> (x+y=w1281:u32)
                              n1060 = local write "H2 Device Count"(w1281) -> ()
                            }
                            frame #5 {
                              n1061 = local read "H2 Good Units"() -> (w1287:u32)
                              n1062 = local read "H2 results"() -> (w1285:u32)
                              n1063 = Add(x=w1285, y=w1287) -> (x+y=w1286:u32)
                              n1064 = local write "H2 Good Units"(w1286) -> ()
                            }
                            frame #6 {
                              # "H2 binning and low yield alarms"
                              n1065 = local read "H2 parallelism"() -> (w1297:u8)
                              n1066 = local read "H2 Device Count"() -> (w1310:u32)
                              n1067 = local read "H2 Good Units"() -> (w1309:u32)
                              n1068 = local read "H2 results"() -> (w1296:u32)
                              n1069 = Divide(x=w1309, y=w1310) -> (x/y=w1311:dbl)
                              n1070 = Divide(x=w1296, y=w1297) -> (x/y=w1294:dbl)
                              n1071 = Multiply(x=100, y=w1311) -> (x*y=w1298:dbl)
                              n1072 = local write "H2 Yield  Mon"(w1298) -> ()
                              n1073 = Multiply(x=100, y=w1294) -> (x*y=w1293:dbl)
                              n1074 = local read "H2  low yield warning"() -> (w1314:dbl)
                              n1075 = local read "H1 Yield Guage"() -> (w1292:cluster{dbl, dbl})
                              n1076 = local read "H2 low yield alarm"() -> (w1315:dbl)
                              n1077 = Unbundle(w1292) -> (w1291:dbl)  [unwired: 1 out]
                              n1078 = local read "H1 low yield alarm"() -> (w1307:dbl)
                              n1079 = local read "H2 low yield alarm"() -> (w1306:dbl)
                              n1080 = call "moving_avg_core.vi"("Array in"=w1302, "avg"=w1290, "accumulator in"=w1303, "i"=w1304, "data in"=w1293) -> ("Array out"=w1301:dbl[], "accumulator out"=w1300:dbl, "rolling avg out"=w1299:dbl)  [unwired: 4 in]
                              n1081 = Less?(x=w1299, y=w1314) -> (x < y?=w1313:bool)
                              n1082 = Bundle(w1291, "rolling avg out"=w1299, "H1 low yield alarm"=w1307, "H2 low yield alarm"=w1306) -> (w1305:T8)  [unwired: 1 in]
                              n1083 = case shown="True" w1313 {
                                tunnel: w1299 -> [_ w1322]
                                tunnel: w1315 -> [_ w1321]
                                frame False {
                                n1084 = local write "H2 nominal"(TRUE ("H1 nominal")) -> ()
                                n1085 = local write "H2 warning"(FALSE ("H1 warning")) -> ()
                                n1086 = local write "H2 alarm"(FALSE ("H1 warning")) -> ()
                                }
                                frame True {
                                n1087 = Less?(x=w1322, y=w1321) -> (x < y?=w1323:bool)
                                n1088 = case shown="True" w1323 {
                                frame False {
                                n1089 = local write "H2 nominal"(FALSE ("H1 nominal")) -> ()
                                n1090 = local write "H2 warning"(TRUE ("H1 warning")) -> ()
                                n1091 = local write "H2 alarm"(FALSE ("H1 warning")) -> ()
                                }
                                frame True {
                                n1092 = local read "H2 enable halt\non yield alarm"() -> (w1327:bool)
                                n1093 = case shown="True" w1327 {
                                frame False {
                                }
                                frame True {
                                n1094 = local write "H2 online"(FALSE ("H1 Online")) -> ()
                                }
                                }
                                n1095 = local write "H2 nominal"(FALSE ("H1 nominal")) -> ()
                                n1096 = local write "H2 warning"(FALSE ("H1 warning")) -> ()
                                n1097 = local write "H2 alarm"(TRUE ("H1 warning")) -> ()
                                }
                                }
                                }
                              }
                              n1098 = local write "YieldMon"(w1305) -> ()
                              n1099 = Bundle("rolling avg out"=w1299, "H2 low yield alarm"=w1315) -> (→"H2 Yield Guage":T9)  [unwired: 1 in]
                            }
                            frame #7 {
                              # "start of\nindex time"
                              n1100 = local write "H2 Indexing"(TRUE ("H2 Indexing")) -> ()
                              n1101 = Tick Count (ms)() -> (millisecond timer value=w1334:u32)
                              n1102 = local write "H2 Lock"(FALSE ("H1 Lock")) -> ()
                            }
                          }
                          n1103 = flat-sequence {
                            tunnel: w1253 -> [w1349]
                            tunnel: w1254 -> [w1350]
                            tunnel: w1255 -> [w1351]
                            tunnel: [w1351] -> w1251
                            tunnel: [w1350] -> w1250
                            tunnel: [w1349] -> w1249
                            tunnel: [w1338] -> w1248
                            tunnel: w1248 -> [w1376]
                            tunnel: w1249 -> [w1377]
                            tunnel: w1250 -> [w1378]
                            tunnel: w1251 -> [w1379]
                            tunnel: [w1359] -> w1235
                            tunnel: [w1360] -> w1234
                            tunnel: w1233 -> [w1355]
                            tunnel: w1232 -> [w1356]
                            tunnel: w1231 -> [w1353]
                            tunnel: w1224 -> [w1352]
                            frame #0 {
                              # "index time"
                              # "H2 indexing"
                              n1104 = local read "H2 index time\nvariation (%)"() -> (w1340:i32)
                              n1105 = local read "H2 index\ntime set"() -> (w1341:dbl)
                              n1106 = Divide(x=w1340, y=100.0) -> (x/y=w1344:dbl)
                              n1107 = local read "Time Accerlation  Factor"() -> (w1337:dbl)
                              n1108 = Multiply(x=w1344, y=w1341) -> (x*y=w1346:dbl)
                              n1109 = Random Number (0-1)() -> (number: 0 to 1=w1348:dbl)
                              n1110 = Multiply(x=w1346, y=w1348) -> (x*y=w1347:dbl)
                              n1111 = Add(x=w1347, y=w1341) -> (x+y=w1342:dbl)
                              n1112 = Multiply(x=w1342, y=1000.0) -> (x*y=w1339:dbl)
                              n1113 = Divide(x=w1339, y=w1337) -> (x/y=w1338:dbl)
                              n1114 = Wait (ms)(milliseconds to wait=w1338) -> ()  [unwired: 1 out]
                            }
                            frame #1 {
                              # "calculate test, tindex, and wait times, UPH"
                              # "start of wait time"
                              # "end of test time"
                              # "start of test time"
                              # "Check H2 UPH against warning and alert limits"
                              n1115 = local write "H2 Indexing"(FALSE ("H2 Indexing")) -> ()
                              n1116 = local read "Time Accerlation  Factor"() -> (w1361:dbl)
                              n1117 = local read "Parallelism"() -> (w1391:u32)
                              n1118 = local read "Parallelism"() -> (w1388:u32)
                              n1119 = Equal To 0?(x=w1353) -> (x = 0?=w1354:bool)
                              n1120 = case shown="True" w1354 {
                                tunnel: w1379 -> [w1400 _]
                                tunnel: w1377 -> [w1399 _]
                                tunnel: [w1398 0] -> w1363
                                frame False {
                                n1121 = Subtract(x=w1400, y=w1399) -> (x-y=w1401:u32)
                                n1122 = Divide(x=w1401, y=1000.0) -> (x/y=w1398:dbl)
                                }
                                frame True {
                                }
                              }
                              n1123 = Subtract(x=w1378, y=w1379) -> (x-y=w1381:u32)
                              n1124 = Divide(x=w1376, y=1000.0) -> (x/y=w1365:dbl)
                              n1125 = Divide(x=w1381, y=1000.0) -> (x/y=w1364:dbl)
                              n1126 = Multiply(x=w1391, y=3600.0 ("x")) -> (x*y=w1390:dbl)
                              n1127 = Multiply(x=w1388, y=3600.0 ("x")) -> (x*y=w1386:dbl)
                              n1128 = Compound Arithmetic op=ADD(w1365, w1364, w1363) -> (w1384:dbl)
                              n1129 = Compound Arithmetic op=ADD(w1365, w1364) -> (w1396:dbl)
                              n1130 = Divide(x=w1390, y=w1396) -> (x/y=w1392:dbl)
                              n1131 = Multiply(x=w1361, y=w1365) -> (x*y=→"H2 Index Time" →"H2 IT (scycle)":dbl)
                              n1132 = Multiply(x=w1361, y=w1364) -> (x*y=→"H2 Test Time" →"H2 TT (s/cycle)":dbl)
                              n1133 = Divide(x=w1386, y=w1384) -> (x/y=w1385:dbl)
                              n1134 = Multiply(x=w1361, y=w1363) -> (x*y=→"H2 Wait Time" →"H2 WT (s/cycle)":dbl)
                              n1135 = Divide(x=w1392, y=w1361) -> (x/y=→"H2 Single Handler UPH":dbl)
                              n1136 = Divide(x=w1385, y=w1361) -> (x/y=w1357:dbl)
                              n1137 = call "moving_avg_core.vi"("Array in"=w1356, "avg"=w1352, "accumulator in"=w1355, "i"=w1353, "data in"=w1357) -> ("Array out"=w1360:dbl[], "accumulator out"=w1359:dbl, "rolling avg out"=w1358:dbl)  [unwired: 4 in]
                              n1138 = local read "H2 low UPH warning (%)"() -> (w1367:dbl)
                              n1139 = local read "H2 low UPH alarm (%)"() -> (w1373:dbl)
                              n1140 = property on="H2 UPH" class="Knob (strict)"() -> ("Scale.Maximum"=w1366:dbl)  [unwired: 2 in, 2 out]
                              n1141 = Divide(x=w1373, y=100.0) -> (x/y=w1371:dbl)
                              n1142 = Divide(x=w1367, y=100.0) -> (x/y=w1369:dbl)
                              n1143 = Multiply(x=w1366, y=w1371) -> (x*y=w1375:dbl)
                              "H2 UPH alarm limit" <- w1375
                              n1144 = Multiply(x=w1366, y=w1369) -> (x*y=w1368:dbl)
                              "H2 UPH warning limit" <- w1368
                              n1145 = Less?(x=w1358, y=w1368) -> (x < y?=w1374:bool)
                              n1146 = Bundle("rolling avg out"=w1358, w1375) -> (→"H2 UPH":cluster{"rolling avg out":dbl, dbl})  [unwired: 1 in]
                              n1147 = case shown="True" w1374 {
                                tunnel: w1358 -> [_ w1408]
                                tunnel: w1375 -> [_ w1407]
                                frame False {
                                n1148 = local write "H2 warning 2"(FALSE ("H1 warning")) -> ()
                                n1149 = local write "H2 nominal 2"(TRUE ("H1 nominal")) -> ()
                                n1150 = local write "H2 alarm 2"(FALSE ("H1 warning")) -> ()
                                }
                                frame True {
                                n1151 = Less?(x=w1408, y=w1407) -> (x < y?=w1409:bool)
                                n1152 = case shown="True" w1409 {
                                frame False {
                                n1153 = local write "H2 warning 2"(TRUE ("H1 warning")) -> ()
                                n1154 = local write "H2 nominal 2"(FALSE ("H1 nominal")) -> ()
                                n1155 = local write "H2 alarm 2"(FALSE ("H1 warning")) -> ()
                                }
                                frame True {
                                n1156 = local read "H2 enable halt\non UPH alarm"() -> (w1413:bool)
                                n1157 = local write "H2 warning 2"(FALSE ("H1 warning")) -> ()
                                n1158 = local write "H2 nominal 2"(FALSE ("H1 nominal")) -> ()
                                n1159 = local write "H2 alarm 2"(TRUE ("H1 warning")) -> ()
                                n1160 = case shown="True" w1413 {
                                frame False {
                                }
                                frame True {
                                n1161 = local write "H2 online"(FALSE ("H1 Online")) -> ()
                                }
                                }
                                }
                                }
                                }
                              }
                            }
                            frame #2 {
                              # "update monitors"
                            }
                          }
                        }
                      }
                    }
                  }
                  n1162 = Wait (ms)(milliseconds to wait=u32 10) -> ()  [unwired: 1 out]
                  n1163 = local read "Run / Stop"() -> (w1144:bool)
                  n1164 = local read "POWER"() -> (w1146:bool)
                  n1165 = Not(x=w1144) -> (.not. x?=w1149:bool)
                  n1166 = Not(x=w1146) -> (.not. x?=w1148:bool)
                  n1167 = Compound Arithmetic op=OR(w1149, w1148) -> (w1147:bool)
                }
                n1168 = while {
                  i -> [w294]
                  stop <- w307 stop-if-true
                  # "Play Audio Aert Loop"
                  n1169 = local read "Ignore alarms until AFTER this many cycles"() -> (w299:i32)
                  n1170 = local read "H1 Device Count"() -> (w304:u32)
                  n1171 = local read "H2 Device Count"() -> (w303:u32)
                  n1172 = local read "Parallelism"() -> (w301:u32)
                  n1173 = local read "Run / Stop"() -> (w296:bool)
                  n1174 = local read "POWER"() -> (w297:bool)
                  n1175 = Add(x=w304, y=w303) -> (x+y=w302:u32)
                  n1176 = Wait (ms)(milliseconds to wait=u32 100) -> ()  [unwired: 1 out]
                  n1177 = Divide(x=w302, y=w301) -> (x/y=w300:dbl)
                  n1178 = Greater?(x=w294, y=50) -> (0:w292:bool)
                  n1179 = Greater?(x=w300, y=w299) -> (0:w298:bool)
                  n1180 = Compound Arithmetic op=AND(w298, w297, w296, w292) -> (w295:bool)
                  n1181 = case shown="True" w295 {
                    frame False {
                    }
                    frame True {
                      n1182 = local read "system statuts"() -> (w311:T2)
                      n1183 = case shown="\"H1AH2W\"" w311 {
                        frame "H1NH2N", Default {
                          n1184 = Wait (ms)(milliseconds to wait=u32 50) -> ()  [unwired: 1 out]
                        }
                        frame "H1NH2W" {
                          n1185 = flat-sequence {
                            frame #0 {
                              n1186 = local read "Audio On / Off"() -> (w314:bool)
                              n1187 = local read "H2 online"() -> (w313:bool)
                              n1188 = And(x=w313, y=w314) -> (x .and. y?=w315:bool)
                              n1189 = case shown="True" w315 {
                                frame False {
                                }
                                frame True {
                                n1190 = local read "Run / Stop"() -> (w318:bool)
                                n1191 = case shown="True" w318 {
                                tunnel: [0.001 w320] -> w317
                                frame False {
                                }
                                frame True {
                                n1192 = local read "Alert volume"() -> (w320:u32)
                                }
                                }
                                n1193 = call "PlayAlarm.vi"("wavefilename"="audio\\4_synth_warning.wav", "alertvolume"=w317) -> ()  [unwired: 10 in]
                                }
                              }
                            }
                            frame #1 {
                              n1194 = local read "Run / Stop"() -> (w321:bool)
                              n1195 = case shown="True" w321 {
                                frame False {
                                }
                                frame True {
                                n1196 = Wait (ms)(milliseconds to wait=u32 5000) -> ()  [unwired: 1 out]
                                }
                              }
                            }
                          }
                        }
                        frame "H1NH2A" {
                          n1197 = flat-sequence {
                            frame #0 {
                              n1198 = local read "Audio On / Off"() -> (w325:bool)
                              n1199 = local read "H2 online"() -> (w324:bool)
                              n1200 = And(x=w324, y=w325) -> (x .and. y?=w323:bool)
                              n1201 = case shown="True" w323 {
                                frame False {
                                }
                                frame True {
                                n1202 = local read "Run / Stop"() -> (w328:bool)
                                n1203 = case shown="True" w328 {
                                tunnel: [0.001 w330] -> w327
                                frame False {
                                }
                                frame True {
                                n1204 = local read "Alert volume"() -> (w330:u32)
                                }
                                }
                                n1205 = call "PlayAlarm.vi"("wavefilename"="audio\\bass_synth_alarm.wav", "alertvolume"=w327) -> ()  [unwired: 10 in]
                                }
                              }
                            }
                            frame #1 {
                              n1206 = local read "Run / Stop"() -> (w331:bool)
                              n1207 = case shown="False" w331 {
                                frame False {
                                n1208 = Wait (ms)(milliseconds to wait=u32 50) -> ()  [unwired: 1 out]
                                }
                                frame True {
                                n1209 = Wait (ms)(milliseconds to wait=u32 5000) -> ()  [unwired: 1 out]
                                }
                              }
                            }
                          }
                        }
                        frame "H1WH2N" {
                          n1210 = flat-sequence {
                            frame #0 {
                              n1211 = local read "Audio On / Off"() -> (w336:bool)
                              n1212 = local read "H1 online"() -> (w335:bool)
                              n1213 = And(x=w335, y=w336) -> (x .and. y?=w334:bool)
                              n1214 = case shown="True" w334 {
                                frame False {
                                }
                                frame True {
                                n1215 = local read "Run / Stop"() -> (w339:bool)
                                n1216 = case shown="True" w339 {
                                tunnel: [0.001 w341] -> w338
                                frame False {
                                }
                                frame True {
                                n1217 = local read "Alert volume"() -> (w341:u32)
                                }
                                }
                                n1218 = call "PlayAlarm.vi"("wavefilename"="audio\\4_synth_warning.wav", "alertvolume"=w338) -> ()  [unwired: 10 in]
                                }
                              }
                            }
                            frame #1 {
                              n1219 = local read "Run / Stop"() -> (w342:bool)
                              n1220 = case shown="False" w342 {
                                frame False {
                                n1221 = Wait (ms)(milliseconds to wait=u32 50) -> ()  [unwired: 1 out]
                                }
                                frame True {
                                n1222 = Wait (ms)(milliseconds to wait=u32 5000) -> ()  [unwired: 1 out]
                                }
                              }
                            }
                          }
                        }
                        frame "H1WH2W" {
                          n1223 = flat-sequence {
                            frame #0 {
                              n1224 = local read "Audio On / Off"() -> (w348:bool)
                              n1225 = local read "H1 online"() -> (w345:bool)
                              n1226 = local read "H2 online"() -> (w347:bool)
                              n1227 = Compound Arithmetic op=AND(w345, w347, w348) -> (w346:bool)
                              n1228 = case shown="True" w346 {
                                frame False {
                                }
                                frame True {
                                n1229 = local read "Run / Stop"() -> (w351:bool)
                                n1230 = case shown="True" w351 {
                                tunnel: [0.001 w353] -> w350
                                frame False {
                                }
                                frame True {
                                n1231 = local read "Alert volume"() -> (w353:u32)
                                }
                                }
                                n1232 = call "PlayAlarm.vi"("wavefilename"="audio\\4_synth_warning.wav", "alertvolume"=w350) -> ()  [unwired: 10 in]
                                }
                              }
                            }
                            frame #1 {
                              n1233 = local read "Run / Stop"() -> (w354:bool)
                              n1234 = case shown="False" w354 {
                                frame False {
                                n1235 = Wait (ms)(milliseconds to wait=u32 50) -> ()  [unwired: 1 out]
                                }
                                frame True {
                                n1236 = Wait (ms)(milliseconds to wait=u32 5000) -> ()  [unwired: 1 out]
                                }
                              }
                            }
                          }
                        }
                        frame "H1WH2A" {
                          n1237 = flat-sequence {
                            frame #0 {
                              n1238 = local read "Audio On / Off"() -> (w360:bool)
                              n1239 = local read "H1 online"() -> (w358:bool)
                              n1240 = local read "H2 online"() -> (w359:bool)
                              n1241 = Compound Arithmetic op=AND(w358, w359, w360) -> (w357:bool)
                              n1242 = case shown="True" w357 {
                                frame False {
                                }
                                frame True {
                                n1243 = local read "Run / Stop"() -> (w363:bool)
                                n1244 = case shown="True" w363 {
                                tunnel: [0.001 w365] -> w362
                                frame False {
                                }
                                frame True {
                                n1245 = local read "Alert volume"() -> (w365:u32)
                                }
                                }
                                n1246 = call "PlayAlarm.vi"("wavefilename"="audio\\bass_synth_alarm.wav", "alertvolume"=w362) -> ()  [unwired: 10 in]
                                }
                              }
                            }
                            frame #1 {
                              n1247 = local read "Run / Stop"() -> (w366:bool)
                              n1248 = case shown="False" w366 {
                                frame False {
                                n1249 = Wait (ms)(milliseconds to wait=u32 50) -> ()  [unwired: 1 out]
                                }
                                frame True {
                                n1250 = Wait (ms)(milliseconds to wait=u32 5000) -> ()  [unwired: 1 out]
                                }
                              }
                            }
                          }
                        }
                        frame "H1AH2N" {
                          n1251 = flat-sequence {
                            frame #0 {
                              n1252 = local read "Audio On / Off"() -> (w371:bool)
                              n1253 = local read "H1 online"() -> (w369:bool)
                              n1254 = And(x=w369, y=w371) -> (x .and. y?=w370:bool)
                              n1255 = case shown="True" w370 {
                                frame False {
                                }
                                frame True {
                                n1256 = local read "Run / Stop"() -> (w374:bool)
                                n1257 = case shown="True" w374 {
                                tunnel: [0.001 w376] -> w373
                                frame False {
                                }
                                frame True {
                                n1258 = local read "Alert volume"() -> (w376:u32)
                                }
                                }
                                n1259 = call "PlayAlarm.vi"("wavefilename"="audio\\bass_synth_alarm.wav", "alertvolume"=w373) -> ()  [unwired: 10 in]
                                }
                              }
                            }
                            frame #1 {
                              n1260 = local read "Run / Stop"() -> (w377:bool)
                              n1261 = case shown="False" w377 {
                                frame False {
                                n1262 = Wait (ms)(milliseconds to wait=u32 50) -> ()  [unwired: 1 out]
                                }
                                frame True {
                                n1263 = Wait (ms)(milliseconds to wait=u32 5000) -> ()  [unwired: 1 out]
                                }
                              }
                            }
                          }
                        }
                        frame "H1AH2W" {
                          n1264 = flat-sequence {
                            frame #0 {
                              n1265 = local read "Audio On / Off"() -> (w383:bool)
                              n1266 = local read "H1 online"() -> (w381:bool)
                              n1267 = local read "H2 online"() -> (w382:bool)
                              n1268 = Compound Arithmetic op=AND(w381, w382, w383) -> (w380:bool)
                              n1269 = case shown="True" w380 {
                                frame False {
                                }
                                frame True {
                                n1270 = local read "Run / Stop"() -> (w386:bool)
                                n1271 = case shown="True" w386 {
                                tunnel: [0.001 w388] -> w385
                                frame False {
                                }
                                frame True {
                                n1272 = local read "Alert volume"() -> (w388:u32)
                                }
                                }
                                n1273 = call "PlayAlarm.vi"("wavefilename"="audio\\bass_synth_alarm.wav", "alertvolume"=w385) -> ()  [unwired: 10 in]
                                }
                              }
                            }
                            frame #1 {
                              n1274 = local read "Run / Stop"() -> (w389:bool)
                              n1275 = case shown="False" w389 {
                                frame False {
                                n1276 = Wait (ms)(milliseconds to wait=u32 50) -> ()  [unwired: 1 out]
                                }
                                frame True {
                                n1277 = Wait (ms)(milliseconds to wait=u32 5000) -> ()  [unwired: 1 out]
                                }
                              }
                            }
                          }
                        }
                        frame "H1AH2A" {
                          n1278 = flat-sequence {
                            frame #0 {
                              n1279 = local read "Audio On / Off"() -> (w395:bool)
                              n1280 = local read "H1 online"() -> (w393:bool)
                              n1281 = local read "H2 online"() -> (w394:bool)
                              n1282 = Compound Arithmetic op=AND(w393, w394, w395) -> (w392:bool)
                              n1283 = case shown="True" w392 {
                                frame False {
                                }
                                frame True {
                                n1284 = local read "Run / Stop"() -> (w398:bool)
                                n1285 = case shown="True" w398 {
                                tunnel: [0.001 w400] -> w397
                                frame False {
                                }
                                frame True {
                                n1286 = local read "Alert volume"() -> (w400:u32)
                                }
                                }
                                n1287 = call "PlayAlarm.vi"("wavefilename"="audio\\bass_synth_alarm.wav", "alertvolume"=w397) -> ()  [unwired: 10 in]
                                }
                              }
                            }
                            frame #1 {
                              n1288 = local read "Run / Stop"() -> (w401:bool)
                              n1289 = case shown="False" w401 {
                                frame False {
                                n1290 = Wait (ms)(milliseconds to wait=u32 50) -> ()  [unwired: 1 out]
                                }
                                frame True {
                                n1291 = Wait (ms)(milliseconds to wait=u32 5000) -> ()  [unwired: 1 out]
                                }
                              }
                            }
                          }
                        }
                      }
                    }
                  }
                  n1292 = local read "Run / Stop"() -> (w305:bool)
                  n1293 = local read "POWER"() -> (w308:bool)
                  n1294 = Not(x=w308) -> (.not. x?=w310:bool)
                  n1295 = Not(x=w305) -> (.not. x?=w309:bool)
                  n1296 = Compound Arithmetic op=OR(w310, w309) -> (w307:bool)
                }
                n1297 = local read "Utilization averaging"() -> (w272:i32)
                n1298 = Initialize Array(w287, w272) -> (w290:dbl[])
                n1299 = while {
                  shift-right: [w1705] -> _
                  shift-left: u32 0 ("millisecond timer value") -> [w1706]
                  shift-right: [w1712] -> _
                  shift-left: w287 -> [w1717]
                  shift-right: [w1713] -> _
                  shift-left: w290 -> [w1715]
                  tunnel: w272 -> [w1709]
                  shift-right: [w1707] -> _
                  shift-left: w272 -> [w1708]
                  i -> [w1711]
                  stop <- w1722 stop-if-true
                  # "last EOT"
                  # "tester loop"
                  n1300 = Equal?(x=w1708, y=w1709) -> (x = y?=w1710:bool)
                  n1301 = Select(t=w1708, s=w1710, f=w1709) -> (s? t:f=w1707:i32)
                  n1302 = local read "Run / Stop"() -> (w1720:bool)
                  n1303 = local read "POWER"() -> (w1721:bool)
                  n1304 = flat-sequence {
                    tunnel: [w1729] -> w1718
                    tunnel: w1717 -> [w1729]
                    tunnel: [w1728] -> w1716
                    tunnel: w1715 -> [w1728]
                    tunnel: [w1727] -> w1714
                    tunnel: w1711 -> [w1727]
                    tunnel: w1711 -> [w1725]
                    tunnel: w1706 -> [w1740]
                    tunnel: w1718 -> [w1739]
                    tunnel: w1716 -> [w1738]
                    tunnel: w1714 -> [w1737]
                    tunnel: [w1736] -> w1713
                    tunnel: [w1735] -> w1712
                    tunnel: w1707 -> [w1734]
                    tunnel: [w1733] -> w1705
                    frame #0 {
                      # "first pass init"
                      n1305 = Equal To 0?(x=w1725) -> (x = 0?=w1726:bool)
                      n1306 = case shown="True" w1726 {
                        frame False {
                        }
                        frame True {
                          n1307 = local write "H1 Waiting"(FALSE ("H1 SOT")) -> ()
                          n1308 = local write "H2 Waiting"(FALSE ("H2 SOT")) -> ()
                          n1309 = local write "system states"(T3."No Handler Ready" ("system states")) -> ()
                        }
                      }
                    }
                    frame #1 {
                      n1310 = local read "Tester ready"() -> (w1741:bool)
                      n1311 = case shown="True" w1741 {
                        tunnel: w1740 -> [w1742 w1755]
                        tunnel: w1739 -> [w1743 w1753]
                        tunnel: w1738 -> [w1744 w1751]
                        tunnel: w1737 -> [_ w1749]
                        tunnel: [w1744 w1748] -> w1736
                        tunnel: [w1743 w1747] -> w1735
                        tunnel: w1734 -> [_ w1746]
                        tunnel: [w1742 w1745] -> w1733
                        frame False {
                        }
                        frame True {
                          n1312 = flat-sequence {
                            tunnel: [w1758] -> w1754
                            tunnel: w1753 -> [w1758]
                            tunnel: [w1757] -> w1752
                            tunnel: w1751 -> [w1757]
                            tunnel: [w1756] -> w1750
                            tunnel: w1749 -> [w1756]
                            tunnel: w1755 -> [w1778]
                            tunnel: w1754 -> [w1777]
                            tunnel: w1752 -> [w1776]
                            tunnel: w1750 -> [w1775]
                            tunnel: [w1774] -> w1748
                            tunnel: [w1773] -> w1747
                            tunnel: w1746 -> [w1771]
                            tunnel: [w1770] -> w1745
                            frame #0 {
                              n1313 = local read "H1 Waiting"() -> (w1759:bool)
                              n1314 = case shown="False" w1759 {
                                frame False {
                                n1315 = local read "H2 Waiting"() -> (w1760:bool)
                                n1316 = case shown="False" w1760 {
                                frame False {
                                n1317 = local write "H2 Lock"(FALSE ("H2 Lock")) -> ()
                                n1318 = local write "system states"(T3."No Handler Ready" ("system states")) -> ()
                                n1319 = local write "H1 Lock"(FALSE ("H1 Lock")) -> ()
                                }
                                frame True {
                                n1320 = local write "H2 Lock"(TRUE ("H2 Lock")) -> ()
                                n1321 = local write "system states"(T3."H2 Ready" ("system states")) -> ()
                                n1322 = local write "H1 Lock"(FALSE ("H1 Lock")) -> ()
                                }
                                }
                                }
                                frame True {
                                n1323 = local write "H1 Lock"(TRUE ("H1 Lock")) -> ()
                                n1324 = local write "system states"(T3."H1 Ready" ("system states")) -> ()
                                n1325 = local write "H2 Lock"(FALSE ("H2 Lock")) -> ()
                                }
                              }
                            }
                            frame #1 {
                              n1326 = local read "system states"() -> (w1772:T3)
                              n1327 = case shown="\"H2 Ready\"" w1772 {
                                tunnel: w1778 -> [w1806 w1947 w2064]
                                tunnel: w1777 -> [w1797 w1938 w2066]
                                tunnel: w1776 -> [w1792 w1933 w2065]
                                tunnel: w1775 -> [w1787 w1928 _]
                                tunnel: [w1784 w1925 w2065] -> w1774
                                tunnel: [w1781 w1922 w2066] -> w1773
                                tunnel: w1771 -> [w1780 w1921 _]
                                tunnel: [w1779 w1920 w2064] -> w1770
                                frame "H1 Ready" {
                                # "testing on H1"
                                n1328 = flat-sequence {
                                tunnel: [w1812] -> w1802
                                tunnel: [w1811] -> w1798
                                tunnel: w1797 -> [w1811]
                                tunnel: [w1810] -> w1793
                                tunnel: w1792 -> [w1810]
                                tunnel: [w1809] -> w1788
                                tunnel: w1787 -> [w1809]
                                tunnel: [w1817] -> w1803
                                tunnel: w1802 -> [w1817]
                                tunnel: [w1816] -> w1799
                                tunnel: w1798 -> [w1816]
                                tunnel: [w1815] -> w1794
                                tunnel: w1793 -> [w1815]
                                tunnel: [w1814] -> w1789
                                tunnel: w1788 -> [w1814]
                                tunnel: [w1827] -> w1807
                                tunnel: [w1826] -> w1804
                                tunnel: w1803 -> [w1826]
                                tunnel: [w1825] -> w1800
                                tunnel: w1799 -> [w1825]
                                tunnel: [w1824] -> w1795
                                tunnel: w1794 -> [w1824]
                                tunnel: [w1823] -> w1790
                                tunnel: w1789 -> [w1823]
                                tunnel: [w1842] -> w1808
                                tunnel: w1807 -> [w1842]
                                tunnel: [w1841] -> w1805
                                tunnel: w1804 -> [w1841]
                                tunnel: [w1839] -> w1801
                                tunnel: w1800 -> [w1839]
                                tunnel: [w1838] -> w1796
                                tunnel: w1795 -> [w1838]
                                tunnel: [w1837] -> w1791
                                tunnel: w1790 -> [w1837]
                                tunnel: w1808 -> [w1856]
                                tunnel: w1806 -> [w1854]
                                tunnel: w1805 -> [w1853]
                                tunnel: w1801 -> [w1849]
                                tunnel: w1796 -> [w1848]
                                tunnel: w1791 -> [w1850]
                                tunnel: [w1846] -> w1786
                                tunnel: [w1845] -> w1783
                                tunnel: w1780 -> [w1851]
                                tunnel: w1786 -> [w1878]
                                tunnel: [w1878] -> w1785
                                tunnel: w1783 -> [w1877]
                                tunnel: [w1877] -> w1782
                                tunnel: [w1876] -> w1779
                                tunnel: w1785 -> [w1908]
                                tunnel: [w1908] -> w1784
                                tunnel: w1782 -> [w1907]
                                tunnel: [w1907] -> w1781
                                frame #0 {
                                # "SOT"
                                n1329 = Tick Count (ms)() -> (millisecond timer value=w1812:u32)
                                n1330 = local write "H1 Lock"(TRUE ("H1 Lock")) -> ()
                                }
                                frame #1 {
                                n1331 = local write "H1 Waiting"(FALSE ("H1 Ready")) -> ()
                                n1332 = local write "H1 Testing"(TRUE ("H1 Testing")) -> ()
                                n1333 = local write "H1 Pass"(TRUE ("H1 Result")) -> ()
                                }
                                frame #2 {
                                # "test time"
                                # "testing"
                                n1334 = local read "Test time\nvariation (%)"() -> (w1832:i32)
                                n1335 = local read "Test time set"() -> (w1821:dbl)
                                n1336 = Divide(x=w1832, y=100.0) -> (x/y=w1831:dbl)
                                n1337 = Multiply(x=w1831, y=w1821) -> (x*y=w1834:dbl)
                                n1338 = Random Number (0-1)() -> (number: 0 to 1=w1836:dbl)
                                n1339 = Multiply(x=w1834, y=w1836) -> (x*y=w1835:dbl)
                                n1340 = local read "Time Accerlation  Factor"() -> (w1822:dbl)
                                n1341 = Add(x=w1835, y=w1821) -> (x+y=w1830:dbl)
                                n1342 = Multiply(x=w1830, y=1000.0) -> (x*y=w1828:dbl)
                                n1343 = Divide(x=w1828, y=w1822) -> (x/y=w1827:dbl)
                                n1344 = Wait (ms)(milliseconds to wait=w1827) -> ()  [unwired: 1 out]
                                }
                                frame #3 {
                                n1345 = local write "H1 results"(u32 0 ("H1 Results")) -> ()
                                n1346 = local write "H1 Testing"(FALSE ("H1 Testing")) -> ()
                                }
                                frame #4 {
                                n1347 = local read "Parallelism"() -> (w1858:u32)
                                n1348 = Subtract(x=w1853, y=w1854) -> (x-y=w1857:u32)
                                n1349 = Add(x=w1856, y=w1857) -> (x+y=w1855:dbl)
                                n1350 = for {
                                N: w1858 -> [_]
                                # "binning results"
                                n1351 = local read "H1 yield\nvariation (%)"() -> (w1865:i32)
                                n1352 = local read "H1 yield  set"() -> (w1864:dbl)
                                n1353 = Divide(x=w1865, y=100.0) -> (x/y=w1867:dbl)
                                n1354 = Random Number (0-1)() -> (number: 0 to 1=w1868:dbl)
                                n1355 = Multiply(x=w1868, y=w1867) -> (x*y=w1862:dbl)
                                n1356 = Divide(x=w1864, y=100.0) -> (x/y=w1863:dbl)
                                n1357 = Subtract(x=w1863, y=w1862) -> (x-y=w1861:dbl)
                                n1358 = Subtract(x=1.0, y=w1861) -> (x-y=w1871:dbl)
                                n1359 = Random Number (0-1)() -> (number: 0 to 1=w1872:dbl)
                                n1360 = Greater?(x=w1872, y=w1871) -> (0:w1873:bool)
                                n1361 = case shown="True" w1873 {
                                frame False {
                                }
                                frame True {
                                n1362 = local read "H1 results"() -> (w1875:u32)
                                n1363 = Increment(x=w1875) -> (x+1=w1874:u32)
                                n1364 = local write "H1 results"(w1874) -> ()
                                }
                                }
                                }
                                n1365 = Divide(x=w1856, y=w1855) -> (x/y=w1859:dbl)
                                n1366 = Multiply(x=100.0, y=w1859) -> (x*y=w1844:dbl)
                                n1367 = call "moving_avg_core.vi"("Array in"=w1848, "avg"=w1851, "accumulator in"=w1849, "i"=w1850, "data in"=w1844) -> ("Array out"=w1846:dbl[], "accumulator out"=w1845:dbl, "rolling avg out"=w1847:dbl)  [unwired: 4 in]
                                n1368 = local write "Sys utilization"(w1847) -> ()
                                n1369 = Bundle(w1844, "rolling avg out"=w1847) -> (w1852:cluster{dbl, "rolling avg out":dbl})  [unwired: 1 in]
                                n1370 = local write "SysUtilMon"(w1852) -> ()
                                }
                                frame #5 {
                                # "start EOT timer"
                                n1371 = local write "H1 Lock"(FALSE ("H1 Lock")) -> ()
                                n1372 = Tick Count (ms)() -> (millisecond timer value=w1876:u32)
                                }
                                frame #6 {
                                n1373 = local read "H2 online"() -> (w1896:bool)
                                n1374 = case shown="False" w1896 {
                                tunnel: [0 w1918] -> w1897
                                frame False {
                                }
                                frame True {
                                n1375 = local read "H2 UPH"() -> (w1919:cluster{u32, u32})
                                n1376 = Unbundle(w1919) -> (w1918:u32)  [unwired: 1 out]
                                }
                                }
                                n1377 = local read "Tandem hourly\ncost ($/hr)"() -> (w1911:dbl)
                                n1378 = local read "H1 UPH"() -> (w1912:cluster{u32, u32})
                                n1379 = local read "Tandem\nfloorspace area"() -> (w1915:dbl)
                                n1380 = local read "Std cell \nfloorspace area"() -> (w1914:i32)
                                n1381 = local read "Std hourly\ncost ($/hr)"() -> (w1910:dbl)
                                n1382 = local read "H1 calc UPH"() -> (w1916:dbl)
                                n1383 = local read "System UPH"() -> (w1906:u32)
                                n1384 = local read "H1 calc UPH"() -> (w1909:dbl)
                                n1385 = Unbundle(w1912) -> (w1898:u32)  [unwired: 1 out]
                                n1386 = Add(x=w1898, y=w1897) -> (x+y=w1885:u32)
                                n1387 = local write "Sim H1 UPH"(w1898) -> ()
                                n1388 = local write "Sim H2 UPH"(w1897) -> ()
                                n1389 = Divide(x=w1906, y=w1915) -> (x/y=w1913:dbl)
                                n1390 = Divide(x=w1916, y=w1914) -> (x/y=w1904:dbl)
                                "H1 UPH per unit area" <- w1904
                                n1391 = Divide(x=w1911, y=w1885) -> (x/y=w1900:dbl)
                                n1392 = Divide(x=w1910, y=w1909) -> (x/y=w1902:dbl)
                                n1393 = Bundle(w1913, w1904) -> (w1905:cluster{dbl, dbl})  [unwired: 1 in]
                                n1394 = local write "System UPH"(w1885) -> ()
                                n1395 = local write "UPH per unit area"(w1905) -> ()
                                n1396 = local write "Simulated\nsystem UPH"(w1885) -> ()
                                n1397 = Multiply(x=w1900, y=100.0) -> (x*y=w1880:dbl)
                                n1398 = Multiply(x=w1902, y=100.0) -> (x*y=w1881:dbl)
                                n1399 = Subtract(x=w1881, y=w1880) -> (x-y=w1884:dbl)
                                n1400 = local read "# of devices to test"() -> (w1883:u32)
                                n1401 = local read "Hours per month"() -> (w1890:i32)
                                n1402 = local read "Utilization (%)"() -> (w1889:u32)
                                n1403 = Multiply(x=w1883, y=w1884) -> (x*y=w1882:dbl)
                                n1404 = local write "$ saved"(w1882) -> ()
                                n1405 = local read "# of devices to test"() -> (w1895:u32)
                                n1406 = local write "Tandem unit cost\n(cents/device)"(w1880) -> ()
                                n1407 = local write "Std unit cost\n(cents/device)"(w1881) -> ()
                                n1408 = Bundle(w1880, w1881) -> (w1903:cluster{dbl, dbl})  [unwired: 1 in]
                                n1409 = Divide(x=w1889, y=u32 100) -> (x/y=w1888:dbl)
                                n1410 = local write "Unit cost (cents/device)"(w1903) -> ()
                                n1411 = Multiply(x=w1890, y=w1888) -> (x*y=w1886:dbl)
                                n1412 = Divide(x=w1895, y=w1885) -> (x/y=w1894:dbl)
                                n1413 = Divide(x=w1894, y=w1886) -> (x/y=w1893:dbl)
                                n1414 = Multiply(x=w1893, y=30) -> (x*y=w1891:dbl)
                                n1415 = local write "Calendar days required\nfor testing all units"(w1891) -> ()
                                }
                                }
                                }
                                frame "H2 Ready" {
                                # "testing on H2"
                                n1416 = flat-sequence {
                                tunnel: [w1953] -> w1943
                                tunnel: [w1952] -> w1939
                                tunnel: w1938 -> [w1952]
                                tunnel: [w1951] -> w1934
                                tunnel: w1933 -> [w1951]
                                tunnel: [w1950] -> w1929
                                tunnel: w1928 -> [w1950]
                                tunnel: [w1958] -> w1944
                                tunnel: w1943 -> [w1958]
                                tunnel: [w1957] -> w1940
                                tunnel: w1939 -> [w1957]
                                tunnel: [w1956] -> w1935
                                tunnel: w1934 -> [w1956]
                                tunnel: [w1955] -> w1930
                                tunnel: w1929 -> [w1955]
                                tunnel: [w1968] -> w1949
                                tunnel: [w1967] -> w1945
                                tunnel: w1944 -> [w1967]
                                tunnel: [w1966] -> w1941
                                tunnel: w1940 -> [w1966]
                                tunnel: [w1965] -> w1936
                                tunnel: w1935 -> [w1965]
                                tunnel: [w1964] -> w1931
                                tunnel: w1930 -> [w1964]
                                tunnel: w1949 -> [w1984]
                                tunnel: [w1984] -> w1948
                                tunnel: [w1982] -> w1946
                                tunnel: w1945 -> [w1982]
                                tunnel: [w1980] -> w1942
                                tunnel: w1941 -> [w1980]
                                tunnel: [w1979] -> w1937
                                tunnel: w1936 -> [w1979]
                                tunnel: [w1978] -> w1932
                                tunnel: w1931 -> [w1978]
                                tunnel: w1948 -> [w1996]
                                tunnel: w1947 -> [w1995]
                                tunnel: w1946 -> [w1994]
                                tunnel: w1942 -> [w1990]
                                tunnel: w1937 -> [w1991]
                                tunnel: w1932 -> [w1992]
                                tunnel: [w1986] -> w1927
                                tunnel: [w1987] -> w1924
                                tunnel: w1921 -> [w1985]
                                tunnel: w1927 -> [w2019]
                                tunnel: [w2019] -> w1926
                                tunnel: w1924 -> [w2018]
                                tunnel: [w2018] -> w1923
                                tunnel: [w2017] -> w1920
                                tunnel: w1926 -> [w2051]
                                tunnel: [w2051] -> w1925
                                tunnel: w1923 -> [w2050]
                                tunnel: [w2050] -> w1922
                                frame #0 {
                                # "SOT"
                                n1417 = local write "H2 Lock"(TRUE ("H2 Lock")) -> ()
                                n1418 = Tick Count (ms)() -> (millisecond timer value=w1953:u32)
                                }
                                frame #1 {
                                n1419 = local write "H2 Waiting"(FALSE ("H2 Testing")) -> ()
                                n1420 = local write "H2 Testing"(TRUE ("H2 Testing")) -> ()
                                n1421 = local write "H2 Pass"(TRUE ("H2 Result")) -> ()
                                }
                                frame #2 {
                                # "test time"
                                # "testing"
                                n1422 = local read "Test time\nvariation (%)"() -> (w1974:i32)
                                n1423 = local read "Test time set"() -> (w1962:dbl)
                                n1424 = Divide(x=w1974, y=100.0) -> (x/y=w1972:dbl)
                                n1425 = Multiply(x=w1972, y=w1962) -> (x*y=w1975:dbl)
                                n1426 = Random Number (0-1)() -> (number: 0 to 1=w1977:dbl)
                                n1427 = local read "Time Accerlation  Factor"() -> (w1963:dbl)
                                n1428 = Multiply(x=w1975, y=w1977) -> (x*y=w1976:dbl)
                                n1429 = Add(x=w1976, y=w1962) -> (x+y=w1970:dbl)
                                n1430 = Multiply(x=w1970, y=1000.0) -> (x*y=w1969:dbl)
                                n1431 = Divide(x=w1969, y=w1963) -> (x/y=w1968:dbl)
                                n1432 = Wait (ms)(milliseconds to wait=w1968) -> ()  [unwired: 1 out]
                                }
                                frame #3 {
                                n1433 = local write "H2 results"(u32 0 ("H2 Results")) -> ()
                                n1434 = local write "H2 Testing"(FALSE ("H2 Testing")) -> ()
                                }
                                frame #4 {
                                n1435 = local read "Parallelism"() -> (w1997:u32)
                                n1436 = Subtract(x=w1994, y=w1995) -> (x-y=w1998:u32)
                                n1437 = Add(x=w1996, y=w1998) -> (x+y=w1999:dbl)
                                n1438 = Divide(x=w1996, y=w1999) -> (x/y=w2000:dbl)
                                n1439 = for {
                                N: w1997 -> [_]
                                # "binning results"
                                n1440 = local read "H2 yield\nvariation (%)"() -> (w2002:i32)
                                n1441 = local read "H2 yield set"() -> (w2003:dbl)
                                n1442 = Divide(x=w2002, y=100.0) -> (x/y=w2009:dbl)
                                n1443 = Random Number (0-1)() -> (number: 0 to 1=w2010:dbl)
                                n1444 = Multiply(x=w2010, y=w2009) -> (x*y=w2006:dbl)
                                n1445 = Divide(x=w2003, y=100.0) -> (x/y=w2007:dbl)
                                n1446 = Subtract(x=w2007, y=w2006) -> (x-y=w2005:dbl)
                                n1447 = Subtract(x=1.0, y=w2005) -> (x-y=w2013:dbl)
                                n1448 = Random Number (0-1)() -> (number: 0 to 1=w2014:dbl)
                                n1449 = Greater?(x=w2014, y=w2013) -> (0:w2004:bool)
                                n1450 = case shown="True" w2004 {
                                frame False {
                                }
                                frame True {
                                n1451 = local read "H2 results"() -> (w2016:u32)
                                n1452 = Increment(x=w2016) -> (x+1=w2015:u32)
                                n1453 = local write "H2 results"(w2015) -> ()
                                }
                                }
                                }
                                n1454 = Multiply(x=100.0, y=w2000) -> (x*y=w1989:dbl)
                                n1455 = call "moving_avg_core.vi"("Array in"=w1991, "avg"=w1985, "accumulator in"=w1990, "i"=w1992, "data in"=w1989) -> ("Array out"=w1986:dbl[], "accumulator out"=w1987:dbl, "rolling avg out"=w1988:dbl)  [unwired: 4 in]
                                n1456 = Bundle(w1989, "rolling avg out"=w1988) -> (w1993:cluster{dbl, "rolling avg out":dbl})  [unwired: 1 in]
                                n1457 = local write "Sys utilization"(w1989) -> ()
                                n1458 = local write "SysUtilMon"(w1993) -> ()
                                }
                                frame #5 {
                                # "start EOT timer"
                                n1459 = local write "H2 Lock"(FALSE ("H2 Lock")) -> ()
                                n1460 = Tick Count (ms)() -> (millisecond timer value=w2017:u32)
                                }
                                frame #6 {
                                n1461 = local read "H1 online"() -> (w2037:bool)
                                n1462 = local read "Std hourly\ncost ($/hr)"() -> (w2053:dbl)
                                n1463 = case shown="False" w2037 {
                                tunnel: [0 w2062] -> w2048
                                frame False {
                                }
                                frame True {
                                n1464 = local read "H1 UPH"() -> (w2063:cluster{u32, u32})
                                n1465 = Unbundle(w2063) -> (w2062:u32)  [unwired: 1 out]
                                }
                                }
                                "Sim H1 UPH" <- w2048
                                n1466 = local read "Std cell \nfloorspace area"() -> (w2046:i32)
                                n1467 = local read "H1 calc UPH"() -> (w2052:dbl)
                                n1468 = local read "Tandem\nfloorspace area"() -> (w2059:dbl)
                                n1469 = local read "Std cell \nfloorspace area"() -> (w2058:i32)
                                n1470 = local read "Tandem hourly\ncost ($/hr)"() -> (w2054:dbl)
                                n1471 = local read "H2 UPH"() -> (w2056:cluster{u32, u32})
                                n1472 = local read "H2 calc UPH"() -> (w2047:dbl)
                                n1473 = local read "H1 calc UPH"() -> (w2060:dbl)
                                n1474 = local read "System UPH"() -> (w2057:u32)
                                n1475 = Divide(x=w2053, y=w2052) -> (x/y=w2041:dbl)
                                n1476 = Unbundle(w2056) -> (w2055:u32)  [unwired: 1 out]
                                "Sim H2 UPH" <- w2055
                                n1477 = Add(x=w2048, y=w2055) -> (x+y=w2030:u32)
                                "System UPH" <- w2030
                                "Simulated\nsystem UPH" <- w2030
                                n1478 = Divide(x=w2047, y=w2046) -> (x/y=→"H2 UPH per unit area":dbl)
                                n1479 = Divide(x=w2057, y=w2059) -> (x/y=w2042:dbl)
                                "Tandem UPH\nper unit area" <- w2042
                                n1480 = Divide(x=w2060, y=w2058) -> (x/y=w2049:dbl)
                                n1481 = Multiply(x=w2041, y=100.0) -> (x*y=w2036:dbl)
                                "Std unit cost\n(cents/device)" <- w2036
                                n1482 = Bundle(w2042, w2049) -> (w2044:cluster{dbl, dbl})  [unwired: 1 in]
                                n1483 = Divide(x=w2054, y=w2030) -> (x/y=w2039:dbl)
                                n1484 = local read "Hours per month"() -> (w2025:i32)
                                n1485 = local read "Utilization (%)"() -> (w2024:u32)
                                n1486 = local write "UPH per unit area"(w2044) -> ()
                                n1487 = local read "# of devices to test"() -> (w2031:u32)
                                n1488 = Multiply(x=w2039, y=100.0) -> (x*y=w2035:dbl)
                                "Tandem unit cost\n(cents/device)" <- w2035
                                n1489 = Divide(x=w2024, y=u32 100) -> (x/y=w2023:dbl)
                                n1490 = Subtract(x=w2036, y=w2035) -> (x-y=w2034:dbl)
                                n1491 = Multiply(x=w2025, y=w2023) -> (x*y=w2021:dbl)
                                n1492 = local read "# of devices to test"() -> (w2033:u32)
                                n1493 = Bundle(w2035, w2036) -> (w2043:cluster{dbl, dbl})  [unwired: 1 in]
                                n1494 = Multiply(x=w2033, y=w2034) -> (x*y=w2032:dbl)
                                n1495 = local write "Unit cost (cents/device)"(w2043) -> ()
                                n1496 = local write "$ saved"(w2032) -> ()
                                n1497 = Divide(x=w2031, y=w2030) -> (x/y=w2029:dbl)
                                n1498 = Divide(x=w2029, y=w2021) -> (x/y=w2028:dbl)
                                n1499 = Multiply(x=w2028, y=30) -> (x*y=w2026:dbl)
                                n1500 = local write "Calendar days required\nfor testing all units"(w2026) -> ()
                                }
                                }
                                }
                                frame "No Handler Ready", Default {
                                }
                              }
                            }
                          }
                        }
                      }
                    }
                  }
                  n1501 = Not(x=w1721) -> (.not. x?=w1724:bool)
                  n1502 = Not(x=w1720) -> (.not. x?=w1723:bool)
                  n1503 = Compound Arithmetic op=OR(w1724, w1723) -> (w1722:bool)
                  n1504 = Wait (ms)(milliseconds to wait=u32 10) -> ()  [unwired: 1 out]
                }
              }
            }
          }
        }
      }
    }
  }
